vi "WVDIAL+HSRL_v5.7.vi"() -> ()   [LabVIEW 2012]
uses:
  C:/Users/eol-lidar/Desktop/20171016_WVDIALLabviewSlimmed/DLLs/PowerMeterCommands.dll
  DLLs/PowerMeterCommands.dll
  <vilib>/DAQmx/write.llb/DAQmx Write (Digital 1D Bool NChan 1Samp 1Line).vi
  <vilib>/DAQmx/miscellaneous.llb/DAQmx Fill In Error Info.vi
  <vilib>/Analysis/baseanly.llb/Mean (DBL).vi
  WVD-MCSupdate/WVDMCSupdate/Subroutines/AMCS_Data.vi
  Shared Telescope WV DIAL Code/Libraries and VIs/Scalar_Data.vi
  <vilib>/Analysis/NI_AALBase.lvlib
  Shared Telescope WV DIAL Code/Libraries and VIs/Scalar_Data_2.vi
  Shared Telescope WV DIAL Code/Libraries and VIs/Scalar_Data_4.vi
  Shared Telescope WV DIAL Code/Libraries and VIs/Scalar_Data_3.vi
  DLLs/CLDevIFace.dll
panel:
  out "WV_averaged_energy":dbl
  out "HSRL Pulse Energy":dbl=268435849.0
  out "sigma_off_total":dbl[](array[numeric])=[2.332364381390243e-25, 2.320697167741241e-25, 2.3090708671335277e-25, 2.2974854045109554e-25, 2.2859407047236247e-25, 2.2744366925441805e-25, 2.26297329267526e-25, 2.251550429733533e-25, 2.2401680282644585e-25, 2.2288260127492416e-25, 2.2175243076078264e-25, 2.206262837187045e-25, 2.1950415257769166e-25, 2.1838602976065434e-25, 2.1727190768500615e-25, 2.161617787640884e-25, 2.150556354040113e-25, 2.139534700076229e-25, 2.128552749731104e-25, 2.1176104269312273e-25, 2.106707655578666e-25, 2.095844359523096e-25, 2.0850204625897537e-25, 2.07423588855007e-25, 2.0634905611586077e-25, 2.0527844041435244e-25, 2.042117341187966e-25, 2.0314892959637173e-25, 2.0209001921078091e-25, 2.0103499532413001e-25, 1.999838502961473e-25, 1.9893657648563364e-25, 1.9789316624809672e-25, 1.968536119385491e-25, 1.9581790591098874e-25, 1.9478604051732858e-25, 1.9375800811030392e-25, 1.927338010402081e-25, 1.9171341165660125e-25, 1.906968323104925e-25, 1.896840553510801e-25, 1.886750731283709e-25, 1.8766987799273976e-25, 1.8666846229359852e-25, 1.8567081838116636e-25, 1.8467693860806868e-25, 1.836868153253588e-25, 1.8270044088719615e-25, 1.817178076472234e-25, 1.8073890796061964e-25, 1.79763734185635e-25, 1.7879227868062795e-25, 1.7782453380578935e-25, 1.768604919240875e-25, 1.7590014540037582e-25, 1.749434866014823e-25, 1.7399050789715296e-25, 1.730412016588477e-25, 1.7209556026229894e-25, 1.7115357608504846e-25, 1.702152415083449e-25, 1.6928054891539068e-25, 1.683494906948679e-25, 1.6742205923727613e-25, 1.6649824693748224e-25, 1.6557804619481728e-25, 1.6466144941105022e-25, 1.6374844899312795e-25, 1.628390373525037e-25, 1.6193320690437255e-25, 1.6103095006874383e-25, 1.6013225927008365e-25, 1.5923712693844951e-25, 1.583455455079352e-25, 1.574575074182417e-25, 1.5657300511364835e-25, 1.5569203104400362e-25, 1.5481457766563459e-25, 1.5394063743870112e-25, 1.5307020282994145e-25, 1.5220326631172624e-25, 1.5133982036225366e-25, 1.504798574650267e-25, 1.4962337011087375e-25, 1.487703507953352e-25, 1.4792079202121825e-25, 1.4707468629670718e-25, 1.4623202613699525e-25, 1.4539280406325658e-25, 1.445570126035909e-25, 1.437246442916907e-25, 1.4289569166816877e-25, 1.420701472813628e-25, 1.4124800368397896e-25, 1.404292534373148e-25, 1.3961388910802234e-25, 1.3880190327064917e-25, 1.379932885048454e-25, 1.3718803739826132e-25, 1.363861425446402e-25, 1.3558759654469082e-25, 1.3479239200466308e-25, 1.340005215388192e-25, 1.3321197776706568e-25, 1.3242675331561804e-25, 1.3164484081795858e-25, 1.3086623291318859e-25, 1.3009092224713183e-25, 1.2931890147120559e-25, 1.2855016324406373e-25, 1.2778470022930174e-25, 1.2702250509659302e-25, 1.262635705221593e-25, 1.2550788918685104e-25, 1.247554537782134e-25, 1.2400625698773462e-25, 1.2326029151422749e-25, 1.2251755005947574e-25, 1.217780253321077e-25, 1.210417100438592e-25, 1.2030859691283492e-25, 1.195786786605972e-25, 1.18851948012544e-25, 1.1812839769908239e-25, 1.1740802045427834e-25, 1.1669080901584555e-25, 1.159767561249783e-25, 1.152658545258569e-25, 1.1455809696620013e-25, 1.1385347619616093e-25, 1.131519849688941e-25, 1.1245361603937508e-25, 1.117583621651525e-25, 1.1106621610513389e-25, 1.1037717062058639e-25, 1.0969121847338734e-25, 1.0900835242690863e-25, 1.083285652457594e-25, 1.0765184969416566e-25, 1.0697819853741232e-25, 1.0630760454058555e-25, 1.0564006046922136e-25, 1.0497555908692916e-25, 1.0431409315784699e-25, 1.0365565544491242e-25, 1.0300023870946222e-25, 1.0234783571134161e-25, 1.0169843920857879e-25, 1.0105204195706285e-25, 1.0040863671053026e-25, 9.976821621998412e-26, 9.913077323333622e-26, 9.849630049554962e-26, 9.786479074821712e-26, 9.723623672876652e-26, 9.661063117109184e-26, 9.598796680486343e-26, 9.536823635511549e-26, 9.475143254257759e-26, 9.413754808236696e-26, 9.352657568504201e-26, 9.291850805513504e-26, 9.23133378922368e-26, 9.171105788951196e-26, 9.111166073406451e-26, 9.051513910691544e-26, 8.992148568247254e-26, 8.933069312831499e-26, 8.874275410530924e-26, 8.81576612669431e-26, 8.757540725943283e-26, 8.699598472176303e-26, 8.641938628496673e-26, 8.584560457246932e-26, 8.527463219959786e-26, 8.470646177359393e-26, 8.414108589358719e-26, 8.357849715001561e-26, 8.301868812469757e-26, 8.246165139113372e-26, 8.190737951368418e-26, 8.135586504842031e-26, 8.080710054163341e-26, 8.026107853101331e-26, 7.971779154486073e-26, 7.917723210229574e-26, 7.863939271325362e-26, 7.810426587789643e-26, 7.757184408704574e-26, 7.704211982217247e-26, 7.651508555513636e-26, 7.599073374786113e-26, 7.546905685292702e-26, 7.495004731290133e-26, 7.443369756106717e-26, 7.392000002064816e-26, 7.340894710500448e-26, 7.290053121808379e-26, 7.239474475327379e-26, 7.189158009533459e-26, 7.139102961790172e-26, 7.08930856857546e-26, 7.039774065355878e-26, 6.990498686564234e-26, 6.941481665748396e-26, 6.892722235390593e-26, 6.844219627029562e-26, 6.795973071186417e-26, 6.747981797479669e-26, 6.700245034457727e-26, 6.65276200971648e-26, 6.605531949891227e-26, 6.558554080616818e-26, 6.511827626512511e-26, 6.465351811259903e-26, 6.419125857514812e-26, 6.373148986943393e-26, 6.327420420220038e-26, 6.281939377011968e-26, 6.236705075965837e-26, 6.191716734741186e-26, 6.146973569929855e-26, 6.102474797122153e-26, 6.058219630831991e-26, 6.014207284541432e-26, 5.970436970619037e-26, 5.926907900376932e-26, 5.883619284018171e-26, 5.840570330591657e-26, 5.797760248023143e-26, 5.755188243052344e-26, 5.7128535211937e-26, 5.67075528677253e-26, 5.628892742806664e-26, 5.587265091058773e-26, 5.545871531927239e-26, 5.504711264423169e-26, 5.463783486157487e-26, 5.423087393251913e-26, 5.382622180326292e-26, 5.342387040404202e-26, 5.302381164874635e-26, 5.262603743431294e-26, 5.223053963979678e-26, 5.183731012619226e-26, 5.1446340734933826e-26, 5.1057623287742163e-26, 5.0671149585204396e-26, 5.02869114061869e-26, 4.9904900506887876e-26, 4.952510861986862e-26, 4.914752745251303e-26, 4.8772148686291695e-26, 4.8398963975726275e-26, 4.802796494689824e-26, 4.7659143195831185e-26, 4.7292490287976645e-26, 4.6927997756069023e-26, 4.656565709905916e-26, 4.6205459780420596e-26, 4.5847397226655986e-26, 4.5491460825835027e-26, 4.5137641925350806e-26, 4.4785931831311394e-26, 4.443632180571596e-26, 4.408880306506575e-26, 4.3743366778969376e-26, 4.340000406767262e-26, 4.3058706000731246e-26, 4.2719463594760814e-26, 4.238226781216286e-26, 4.204710955839959e-26, 4.171397968143844e-26, 4.138286896858962e-26, 4.10537681461195e-26, 4.072666787674034e-26, 4.040155875820923e-26, 4.0078431322471164e-26, 3.9757276033364395e-26, 3.9438083286394643e-26, 3.912084340726284e-26, 3.880554665095062e-26, 3.849218320163894e-26, 3.8180743171758126e-26, 3.7871216602626614e-26, 3.756359346426346e-26, 3.725786365612738e-26, 3.695401700813683e-26, 3.66520432821765e-26, 3.63519321737591e-26, 3.60536733146003e-26, 3.5757256275222147e-26, 3.546267056861835e-26, 3.516990565412017e-26, 3.48789509420622e-26, 3.458979579878315e-26, 3.430242955313054e-26, 3.40168415023669e-26, 3.3733020919928976e-26, 3.345095706363949e-26, 3.317063918393493e-26, 3.2892056533936244e-26, 3.2615198379443223e-26, 3.234005401005175e-26, 3.206661275068879e-26, 3.179486397425954e-26, 3.1524797114255725e-26, 3.125640167867499e-26, 3.09896672641198e-26, 3.0724583570023383e-26, 3.046114041394335e-26, 3.0199327746539526e-26, 2.9939135667250263e-26, 2.968055443914684e-26, 2.9423574505128714e-26, 2.9168186502296844e-26, 2.891438127743385e-26, 2.8662149900966553e-26, 2.841148368095994e-26, 2.816237417598619e-26, 2.791481320722609e-26, 2.7668792869488795e-26, 2.742430554080934e-26, 2.718134389112318e-26, 2.693990088912774e-26, 2.66999698074146e-26, 2.6461544226517236e-26, 2.6224618036475193e-26, 2.598918543714353e-26, 2.5755240935978997e-26, 2.55227793446944e-26, 2.5291795773344677e-26, 2.506228562275398e-26, 2.4834244575138018e-26, 2.4607668582883306e-26, 2.438255385569937e-26, 2.4158896845945432e-26, 2.3936694232798251e-26, 2.371594290486372e-26, 2.349663994197427e-26, 2.3278782595424064e-26, 2.3062368268002568e-26, 2.2847394493076405e-26, 2.2633858913405882e-26, 2.2421759259664502e-26, 2.2211093328951717e-26, 2.2001858963497252e-26, 2.1794054029696938e-26, 2.158767639770168e-26, 2.138272392158188e-26, 2.1179194420452825e-26, 2.0977085660508756e-26, 2.0776395337905693e-26, 2.0577121063165076e-26, 2.037926034667947e-26, 2.018281058531128e-26, 1.99877690506497e-26, 1.9794132878407814e-26, 1.9601899059288993e-26, 1.9411064431318812e-26, 1.9221625673258913e-26, 1.9033579299585288e-26, 1.8846921656793268e-26, 1.8661648920586673e-26, 1.847775709457811e-26, 1.8295242010014096e-26, 1.8114099326188242e-26, 1.7934324532407428e-26, 1.775591295030433e-26, 1.7578859736980766e-26, 1.7403159889222226e-26, 1.7228808247949143e-26, 1.7055799503287488e-26, 1.688412820024058e-26, 1.6713788744552824e-26, 1.6544775409065492e-26, 1.637708234013833e-26, 1.621070356441011e-26, 1.6045632995668e-26, 1.588186444155174e-26, 1.571939161069008e-26, 1.5558208119481574e-26, 1.539830749889085e-26, 1.5239683201286934e-26, 1.5082328606968512e-26, 1.492623703067143e-26, 1.4771401727800933e-26, 1.461781590053534e-26, 1.4465472703745876e-26, 1.4314365250563953e-26, 1.4164486617845617e-26, 1.4015829851356042e-26, 1.3868387970670347e-26, 1.372215397393606e-26, 1.3577120842198647e-26, 1.3433281543732342e-26, 1.3290629037929928e-26, 1.3149156278959545e-26, 1.3008856219417433e-26, 1.2869721813426649e-26, 1.2731746019815118e-26, 1.2594921804819474e-26, 1.245924214476847e-26, 1.2324700028536295e-26, 1.2191288459758865e-26, 1.205900045887559e-26, 1.1927829065033005e-26, 1.1797767337869046e-26, 1.1668808358980381e-26, 1.1540945233430018e-26, 1.1414171091057127e-26, 1.1288479087555434e-26, 1.1163862405612263e-26, 1.104031425576237e-26, 1.091782787727406e-26, 1.0796396538871236e-26, 1.0676013539317827e-26, 1.0556672208023929e-26, 1.0438365905502061e-26, 1.0321088023734669e-26, 1.0204831986549954e-26, 1.0089591249905554e-26, 9.975359302025957e-27, 9.862129663617662e-27, 9.749895887973517e-27, 9.63865156105144e-27, 9.528390301448673e-27, 9.419105760458501e-27, 9.310791622019825e-27, 9.203441602575011e-27, 9.097049451061688e-27, 8.991608948776884e-27, 8.887113909137442e-27, 8.783558177658376e-27, 8.680935631666101e-27, 8.579240180169365e-27, 8.478465763623746e-27, 8.378606353692343e-27, 8.279655953065625e-27, 8.181608595193189e-27, 8.084458344058879e-27, 7.988199293893197e-27, 7.892825568987107e-27, 7.798331323397119e-27, 7.704710740628208e-27, 7.611958033526109e-27, 7.520067443844823e-27, 7.429033242095497e-27, 7.338849727257468e-27, 7.249511226494639e-27, 7.161012094933005e-27, 7.073346715375045e-27, 6.986509498044532e-27, 6.90049488038543e-27, 6.81529732672126e-27, 6.730911328102361e-27, 6.64733140200458e-27, 6.564552092115001e-27, 6.482567968084595e-27, 6.401373625321456e-27, 6.320963684734177e-27, 6.2413327925242824e-27, 6.162475619977861e-27, 6.084386863225426e-27, 6.0070612430594456e-27, 5.93049350473708e-27, 5.854678417728619e-27, 5.7796107755822155e-27, 5.705285395699283e-27, 5.631697119157481e-27, 5.558840810516501e-27, 5.486711357676057e-27, 5.415303671645201e-27, 5.3446126864241e-27, 5.274633358812004e-27, 5.205360668273596e-27, 5.136789616728847e-27, 5.068915228464904e-27, 5.001732549942197e-27, 4.935236649672937e-27, 4.869422618068433e-27, 4.804285567298274e-27, 4.7398206311792526e-27, 4.67602296502107e-27, 4.612887745512478e-27, 4.5504101705978505e-27, 4.488585459351163e-27, 4.4274088518740324e-27, 4.366875609158459e-27, 4.306981013010063e-27, 4.247720365906535e-27, 4.18908899092025e-27, 4.1310822316100614e-27, 4.0736954519098816e-27, 4.016924036061156e-27, 3.960763388494195e-27, 3.905208933744127e-27, 3.850256116386455e-27, 3.79590040090594e-27, 3.742137271667819e-27, 3.6889622327949254e-27, 3.63637080812266e-27, 3.58435854108821e-27, 3.532920994696357e-27, 3.482053751411668e-27, 3.4317524131156784e-27, 3.3820126010277366e-27, 3.332829955639945e-27, 3.284200136649963e-27, 3.2361188229165776e-27, 3.1885817123724097e-27, 3.1415845219948863e-27, 3.095122987735941e-27, 3.0491928644700905e-27, 3.0037899259518407e-27, 2.958909964743249e-27, 2.914548792187844e-27, 2.8707022383363006e-27, 2.8273661519104936e-27, 2.7845364002578585e-27, 2.742208869297717e-27, 2.700379463492681e-27, 2.659044105789684e-27, 2.6181987375948592e-27, 2.5778393187241496e-27, 2.5379618273728972e-27, 2.4985622600683314e-27, 2.4596366316510014e-27, 2.4211809752142476e-27, 2.3831913420937183e-27, 2.3456638018206104e-27, 2.3085944420907525e-27, 2.271979368742305e-27, 2.235814705714131e-27, 2.200096595014933e-27, 2.164821196714334e-27, 2.1299846888874138e-27, 2.0955832676121665e-27, 2.061613146922824e-27, 2.0280705588054778e-27, 1.9949517531484858e-27, 1.9622529977418628e-27, 1.929970578245345e-27, 1.8981007981568767e-27, 1.866639978803457e-27, 1.8355844593123698e-27, 1.804930596599854e-27, 1.774674765337153e-27, 1.7448133579373653e-27, 1.715342784545853e-27, 1.686259473007412e-27, 1.657559868855308e-27, 1.629240435298082e-27, 1.6012976531931827e-27, 1.5737280210392883e-27, 1.5465280549576587e-27, 1.5196942886780578e-27]
  out "sigma_on_total":dbl[](array[numeric])=[2.4625508330472582e-23, 2.4527159853669705e-23, 2.4428740710389365e-23, 2.4330256235021162e-23, 2.4231711731485397e-23, 2.413311246438279e-23, 2.4034463665998014e-23, 2.3935770531217886e-23, 2.3837038220808932e-23, 2.3738271855481437e-23, 2.363947652194091e-23, 2.354065726790698e-23, 2.3441819104494084e-23, 2.3342967003119844e-23, 2.3244105897895672e-23, 2.31452406834776e-23, 2.304637621655468e-23, 2.2947517312839898e-23, 2.284866874947935e-23, 2.274983526208387e-23, 2.2651021548034267e-23, 2.2552232261770784e-23, 2.2453472020760115e-23, 2.2354745396413204e-23, 2.2256056922707838e-23, 2.2157411090680185e-23, 2.2058812350863854e-23, 2.1960265109616345e-23, 2.186177373417321e-23, 2.176334254726737e-23, 2.16649758304535e-23, 2.1566677823093633e-23, 2.1468452720517898e-23, 2.137030467733218e-23, 2.1272237803888927e-23, 2.1174256167903837e-23, 2.1076363794365574e-23, 2.0978564665455582e-23, 2.0880862718807766e-23, 2.0783261851638762e-23, 2.0685765914020924e-23, 2.0588378716350403e-23, 2.049110402431887e-23, 2.039394555974215e-23, 2.0296907001380106e-23, 2.019999198493379e-23, 2.0103204103051482e-23, 2.0006546904536104e-23, 1.991002389599258e-23, 1.981363853864059e-23, 1.9717394252391202e-23, 1.9621294413479896e-23, 1.952534235533098e-23, 1.9429541367045723e-23, 1.9333894696646757e-23, 1.9238405547999238e-23, 1.914307708248763e-23, 1.9047912419885998e-23, 1.895291463612763e-23, 1.8858086764984376e-23, 1.876343179818248e-23, 1.8668952684763187e-23, 1.857465233274633e-23, 1.8480533606982316e-23, 1.8386599332337e-23, 1.8292852289311177e-23, 1.8199295218736272e-23, 1.8105930821158984e-23, 1.801276175403204e-23, 1.7919790634879415e-23, 1.782702003925766e-23, 1.7734452504618375e-23, 1.764209052536127e-23, 1.754993655815298e-23, 1.7457993017035543e-23, 1.736626227799225e-23, 1.7274746676980947e-23, 1.718344851157997e-23, 1.7092370038359167e-23, 1.7001513476664478e-23, 1.6910881006007085e-23, 1.682047476841214e-23, 1.673029686585863e-23, 1.664034936539259e-23, 1.6550634294490077e-23, 1.6461153642030332e-23, 1.637190936129231e-23, 1.6282903368814e-23, 1.6194137543294374e-23, 1.6105613727888785e-23, 1.601733372844626e-23, 1.5929299315126343e-23, 1.584151222397945e-23, 1.5753974153233175e-23, 1.566668676754455e-23, 1.5579651696281607e-23, 1.5492870534454802e-23, 1.5406344842343154e-23, 1.53200761464224e-23, 1.5234065938363693e-23, 1.5148315678510935e-23, 1.506282679169264e-23, 1.497760067132952e-23, 1.4892638678431833e-23, 1.4807942139395617e-23, 1.4723512351289847e-23, 1.4639350577157742e-23, 1.4555458050642286e-23, 1.4471835972573456e-23, 1.4388485513719354e-23, 1.430540781325041e-23, 1.422260398085087e-23, 1.414007509639349e-23, 1.4057822209041305e-23, 1.397584633933156e-23, 1.3894148477689867e-23, 1.3812729587076428e-23, 1.373159060034607e-23, 1.365073242288479e-23, 1.35701559323074e-23, 1.3489861978173715e-23, 1.340985138229009e-23, 1.3330124939573234e-23, 1.3250683417775063e-23, 1.3171527559452338e-23, 1.3092658079451777e-23, 1.3014075666890917e-23, 1.2935780985987886e-23, 1.2857774674695026e-23, 1.278005734609298e-23, 1.2702629589208426e-23, 1.2625491966604325e-23, 1.2548645018972756e-23, 1.2472089261122236e-23, 1.2395825185468206e-23, 1.2319853260187866e-23, 1.2244173930563517e-23, 1.2168787619771422e-23, 1.2093694727085487e-23, 1.201889563074398e-23, 1.1944390685652608e-23, 1.1870180226217995e-23, 1.1796264564579593e-23, 1.172264399190066e-23, 1.164931877912693e-23, 1.1576289174773247e-23, 1.1503555409156319e-23, 1.1431117690705314e-23, 1.1358976208694298e-23, 1.1287131133002929e-23, 1.1215582613893397e-23, 1.1144330782277625e-23, 1.1073375750454047e-23, 1.1002717612825146e-23, 1.0932356443802581e-23, 1.0862292301349351e-23, 1.0792525225341324e-23, 1.072305523736658e-23, 1.0653882341902861e-23, 1.0585006526555719e-23, 1.0516427762743505e-23, 1.0448146003690532e-23, 1.0380161187372578e-23, 1.0312473235839991e-23, 1.02450820545726e-23, 1.017798753360374e-23, 1.01111895481767e-23, 1.0044687956810886e-23, 9.978482604560173e-24, 9.912573321075102e-24, 9.846959922109027e-24, 9.781642208049517e-24, 9.716619965832612e-24, 9.651892968316416e-24, 9.587460975732818e-24, 9.52332373302031e-24, 9.459480973330377e-24, 9.395932416584771e-24, 9.332677769690737e-24, 9.269716726754081e-24, 9.207048969290063e-24, 9.144674167996041e-24, 9.082591980187603e-24, 9.02080205158559e-24, 8.959304016889022e-24, 8.898097498808089e-24, 8.83718210940996e-24, 8.776557449163434e-24, 8.7162231078921e-24, 8.656178665324571e-24, 8.596423689788587e-24, 8.536957739886005e-24, 8.477780363928673e-24, 8.418891100483173e-24, 8.360289478541112e-24, 8.301975016976582e-24, 8.243947225442954e-24, 8.18620560453709e-24, 8.128749645613794e-24, 8.071578831649707e-24, 8.014692636017133e-24, 7.958090524040087e-24, 7.901771952798669e-24, 7.845736370274257e-24, 7.789983217537724e-24, 7.734511926875921e-24, 7.679321923290004e-24, 7.624412623323213e-24, 7.569783437184724e-24, 7.515433766925708e-24, 7.461363007572737e-24, 7.40757054726645e-24, 7.354055767082815e-24, 7.300818041492451e-24, 7.247856738183225e-24, 7.195171218202832e-24, 7.142760836711679e-24, 7.090624942188402e-24, 7.038762877181533e-24, 6.987173978433868e-24, 6.935857576708368e-24, 6.884812996920365e-24, 6.834039558853511e-24, 6.783536576104506e-24, 6.733303357674044e-24, 6.683339207201171e-24, 6.633643422518733e-24, 6.584215297489166e-24, 6.535054120403026e-24, 6.486159174952553e-24, 6.437529740614361e-24, 6.389165091649568e-24, 6.341064498325356e-24, 6.293227226467728e-24, 6.2456525381077956e-24, 6.1983396902435295e-24, 6.151287936822558e-24, 6.104496527501172e-24, 6.0579647080188635e-24, 6.011691720302102e-24, 5.965676803332971e-24, 5.919919192206112e-24, 5.8744181179864905e-24, 5.829172809574231e-24, 5.784182492018668e-24, 5.7394463868786454e-24, 5.694963713545303e-24, 5.650733687844412e-24, 5.6067555226267894e-24, 5.5630284285725715e-24, 5.519551613069912e-24, 5.476324281024295e-24, 5.43334563516773e-24, 5.3906148752017374e-24, 5.34813119904406e-24, 5.3058938017475215e-24, 5.2639018765006215e-24, 5.222154614242014e-24, 5.180651203738997e-24, 5.13939083210488e-24, 5.0983726842026865e-24, 5.057595942945583e-24, 5.017059789585322e-24, 4.976763403989191e-24, 4.936705964060656e-24, 4.896886645818459e-24, 4.857304624305925e-24, 4.817959073015348e-24, 4.778849163546343e-24, 4.7399740669056344e-24, 4.7013329523320734e-24, 4.662924987776317e-24, 4.624749340755355e-24, 4.586805176615996e-24, 4.549091660777239e-24, 4.5116079568120655e-24, 4.474353227687181e-24, 4.437326635994939e-24, 4.400527342481393e-24, 4.363954508194969e-24, 4.327607292829392e-24, 4.291484855352226e-24, 4.255586354786274e-24, 4.21991094878835e-24, 4.1844577951629254e-24, 4.149226050818604e-24, 4.114214872712741e-24, 4.079423416657998e-24, 4.044850839129298e-24, 4.010496295553295e-24, 3.976358941574372e-24, 3.942437932236539e-24, 3.908732422878395e-24, 3.875241568493912e-24, 3.841964524111771e-24, 3.8089004445060674e-24, 3.77604848472963e-24, 3.743407799821842e-24, 3.7109775448496736e-24, 3.6787568751051834e-24, 3.646744945826577e-24, 3.614940912861531e-24, 3.583343931919993e-24, 3.551953159080269e-24, 3.520767750819167e-24, 3.48978686389268e-24, 3.459009655371579e-24, 3.428435282822815e-24, 3.398062904337347e-24, 3.367891678126286e-24, 3.3379207634216245e-24, 3.308149319353983e-24, 3.278576506269015e-24, 3.2492014844797096e-24, 3.2200234154212834e-24, 3.1910414609759742e-24, 3.1622547835091576e-24, 3.1336625464392295e-24, 3.105263913718335e-24, 3.077058049866742e-24, 3.0490441205265137e-24, 3.0212212919554575e-24, 2.993588731187521e-24, 2.9661456063117672e-24, 2.938891086110655e-24, 2.9118243402152735e-24, 2.8849445392530034e-24, 2.8582508548661334e-24, 2.83174245960934e-24, 2.805418526973212e-24, 2.7792782314072863e-24, 2.7533207485771068e-24, 2.7275452549106983e-24, 2.7019509282066268e-24, 2.676536946955093e-24, 2.65130249127828e-24, 2.6262467418057974e-24, 2.601368880939825e-24, 2.5766680916364768e-24, 2.552143558429287e-24, 2.5277944668893196e-24, 2.5036200038621456e-24, 2.4796193572700426e-24, 2.4557917163440066e-24, 2.432136271843243e-24, 2.408652215237557e-24, 2.3853387397641406e-24, 2.3621950397159215e-24, 2.3392203108656813e-24, 2.3164137500783173e-24, 2.2937745558238835e-24, 2.2713019277921793e-24, 2.2489950670083638e-24, 2.22685317584767e-24, 2.2048754582373562e-24, 2.1830611194759734e-24, 2.1614093661554926e-24, 2.1399194064524524e-24, 2.118590449772077e-24, 2.0974217072161272e-24, 2.0764123913175484e-24, 2.0555617157912343e-24, 2.0348688963376748e-24, 2.014333149601918e-24, 1.9939536942280065e-24, 1.9737297501740007e-24, 1.9536605387321687e-24, 1.9337452830413488e-24, 1.9139832077558902e-24, 1.8943735388152807e-24, 1.8749155039447973e-24, 1.8556083325745714e-24, 1.836451255374024e-24, 1.8174435048180336e-24, 1.7985843149555666e-24, 1.779872921494777e-24, 1.7613085616590394e-24, 1.7428904742740746e-24, 1.7246178999963703e-24, 1.706490080876167e-24, 1.688506260735766e-24, 1.67066568509952e-24, 1.652967600988165e-24, 1.6354112573505205e-24, 1.6179959045079075e-24, 1.6007207947196642e-24, 1.5835851817734365e-24, 1.5665883211992682e-24, 1.549729470273379e-24, 1.5330078878919895e-24, 1.5164228347105305e-24, 1.4999735731470965e-24, 1.4836593672601718e-24, 1.4674794829453382e-24, 1.4514331876891116e-24, 1.4355197508254798e-24, 1.419738443475347e-24, 1.4040885383117088e-24, 1.388569310046027e-24, 1.3731800348365029e-24, 1.3579199909426112e-24, 1.342788458086281e-24, 1.327784718035644e-24, 1.3129080540946768e-24, 1.2981577515607805e-24, 1.2835330973375337e-24, 1.26903338027142e-24, 1.2546578909355328e-24, 1.2404059216902307e-24, 1.2262767667918795e-24, 1.2122697222380488e-24, 1.1983840857753642e-24, 1.1846191571075761e-24, 1.1709742376439593e-24, 1.1574486307543798e-24, 1.1440416414751332e-24, 1.1307525767609108e-24, 1.1175807454362942e-24, 1.1045254581039964e-24, 1.0915860272441287e-24, 1.0787617671245363e-24, 1.0660519939877606e-24, 1.0534560258245474e-24, 1.04097318247118e-24, 1.0286027857002782e-24, 1.0163441591336192e-24, 1.0041966282035836e-24, 9.92159520201455e-25, 9.802321644465981e-25, 9.684138919121806e-25, 9.56704035604766e-25, 9.451019303983845e-25, 9.336069129593208e-25, 9.222183219101463e-25, 9.109354977514304e-25, 8.997577829031332e-25, 8.886845216306286e-25, 8.77715060087434e-25, 8.668487464281262e-25, 8.560849305520192e-25, 8.454229644363315e-25, 8.348622018112683e-25, 8.244019984154291e-25, 8.1404171188931855e-25, 8.037807017106822e-25, 7.936183294026076e-25, 7.835539582967759e-25, 7.735869536732837e-25, 7.637166827936458e-25, 7.539425147725231e-25, 7.442638207102039e-25, 7.346799736295037e-25, 7.251903484175774e-25, 7.157943220136464e-25, 7.064912731956171e-25, 6.9728058273561595e-25, 6.88161633340924e-25, 6.791338096567603e-25, 6.701964982690402e-25, 6.61349087734962e-25, 6.525909685563692e-25, 6.439215331824889e-25, 6.353401760126324e-25, 6.268462934252213e-25, 6.184392837266436e-25, 6.101185472583387e-25, 6.0188348621694805e-25, 5.937335048636966e-25, 5.8566800942157565e-25, 5.776864079808227e-25, 5.697881107478359e-25, 5.619725298250847e-25, 5.542390792885821e-25, 5.465871752134281e-25, 5.390162356973914e-25, 5.315256807486063e-25, 5.241149324030067e-25, 5.1678341470200395e-25, 5.095305536292852e-25, 5.023557772008194e-25, 4.952585154435521e-25, 4.882382003144208e-25, 4.812942658286226e-25, 4.744261479979235e-25, 4.676332848135732e-25, 4.609151162889621e-25, 4.542710844416201e-25, 4.477006333333286e-25, 4.412032089587425e-25, 4.347782594176257e-25, 4.284252347666972e-25, 4.221435871147735e-25, 4.159327705702398e-25, 4.097922412620583e-25, 4.0372145739307014e-25, 3.97719879138551e-25, 3.9178696871826257e-25, 3.8592219041386377e-25, 3.801250105051675e-25, 3.743948973222074e-25, 3.687313212310302e-25, 3.6313375466665607e-25, 3.57601672058255e-25, 3.521345499384773e-25, 3.4673186682507077e-25, 3.41393103342396e-25, 3.361177421349018e-25, 3.309052679134557e-25, 3.2575516744308053e-25, 3.2066692955889386e-25, 3.156400451278687e-25, 3.1067400711850723e-25, 3.057683105489688e-25, 3.0092245249061445e-25, 2.9613593210871453e-25, 2.9140825062631734e-25, 2.8673891136375487e-25, 2.8212741969193266e-25, 2.775732830716305e-25, 2.7307601105501903e-25, 2.686351152759651e-25, 2.6425010943041874e-25, 2.5992050934598855e-25, 2.5564583291660275e-25, 2.5142560011733776e-25, 2.472593330387952e-25, 2.4314655586748254e-25, 2.390867948982882e-25, 2.35079578506624e-25, 2.3112443719124123e-25, 2.2722090354652053e-25, 2.233685122844375e-25, 2.195668002362015e-25, 2.158153063268651e-25, 2.121135716059416e-25, 2.0846113925777074e-25, 2.0485755456818577e-25, 2.0130236495370295e-25, 1.977951199549295e-25, 1.9433537124710145e-25, 1.9092267261784236e-25, 1.8755658001017306e-25, 1.8423665149969254e-25, 1.809624472667617e-25, 1.7773352967583335e-25, 1.7454946320086584e-25, 1.7140981448046972e-25, 1.683141522831366e-25, 1.6526204752468635e-25, 1.6225307329089313e-25, 1.592868047980234e-25, 1.5636281943616514e-25, 1.5348069673765125e-25, 1.5064001839312553e-25, 1.4784036827229053e-25, 1.450813323820404e-25, 1.423624989244445e-25]
  out "FileHour":i32=6
  out "L_Count":i32
  out "background start":u32=534
  in  "Tab Control 2":enum32{"WV ND ", "Aerosol Backscatter"}(tab)=enum."Aerosol Backscatter"
  out "Absolute Humdity":dbl[][](graph)=[[3.7891452578622107, 3.6848538050283244, 3.4581562862034234, 2.778190123006674, 0.7605224233485954, 2.7235239960819384, 1.8477030284137896, 1.3789174154224018, 3.858909817141913, 2.2998052504653157, 1.8697427873996968, 2.720429333025646, 1.7582764295120719, 1.8343313251572997, 1.160757957156007, 1.3664787572167836, 1.0278245657680662, 0.9747102705897372, 2.2692052714590547, 2.447303873258803, 2.2600819196275466, 2.0700601873456366, 2.0466223675290682, 1.6983309570610874, 1.7492798993149568, 1.7861585039993737, 1.5832308094702108, 1.5864879871964421, 1.5030372754279626, 1.4564317158867097, 1.4228817850819906, 2.096958434429432, 2.4022604300017574, 2.66591970440604, 2.8116941850803556, 1.9044240843725713, 1.66818020635356, 1.534265057004012, 1.772166434272927, 2.497662922277854, 1.6957482922208336, 1.2977864394369667, 1.362279941674365, 1.629191662274515, 1.657338578258699, 1.6301344411474732, 1.516535077188046, 1.3406588492672837, 1.6412452976171872, 1.8344293332702541, 1.9351027937999632, 2.5531676991990513, 2.659011166233257, 1.742648255830912, 1.7524741749995578, 1.6769853502577594, 1.4000548013411225, 1.4245808617975315, 1.37878612948763, 1.7417128820940007, 1.7571933484059967, 1.4600862013864073, 1.1537350022625028, 1.4142394580617093, 1.1174683443965145, 1.2022225697660078, 1.4769074840251073, 1.6984425714113995, 1.8751873013694706, 0.7714280687239269, 0.7769992656400687, 0.9738206307167362, 1.0399777595055186, 1.5775455874643123, 1.9662515652956385, 2.890017835586726, 2.984091683481171, 1.7840363622336388, 1.5747914857098424, 3.3692935433573963, 3.9625775177433993, 2.7959569186438222, 2.8123955756125945, 2.372892243619342, 1.4831028352176765, 0.06273774369447636, -0.5977961214933015, 1.5843209354443428, 2.8625329307407408, 2.5733621942741647, 0.6933039516447836, 0.6539560692382185, 0.8040980030154087, 0.8084018088922339, 1.6344508657792636, 0.37454636863898716, 0.440972361188328, 1.373103149482538, 0.7494498912843306, -1.4788274396233316, -1.1562199736918923, -0.5463545775679522, 1.0349505513673738, 1.138127242006889, -1.0589464926009615, 1.9469246537317555, 2.688644087271129, -0.2951872731857954, -2.6561570659511995, -1.4087504983005419, 0.9568858008879041, -0.27670896981197296, -2.0798321684324503, -0.0002528932543105229, 6.422466595855947, 4.958249789600535, -0.772999155805734, -1.1846414669496275, 0.052326411990904466, -0.47672243031922984, -0.17931113920046696, 5.842686469331913, 3.28233118981728, -0.9449483030259822, -0.32664929120777414, -1.5692345779065195, 4.032753921147751, 9.877331127854655, 8.25122205980245, 7.00075444422831, -0.5203550683182948, -7.139395363542666, -2.245960526012101, 0.9022165152520595, 2.163914779345491, 2.217229143883716, 1.0363924828691926, -1.3944188053069932, -4.557806574544715, 2.1301279232496753, 11.253191554758521, 2.064944061831564, -2.6177477476732083, 1.6398384571905356, -4.091283656679752, -8.308017355766843, -8.23837798110966, -9.616699249521794, -3.0581988015017414, -5.361741358485176, -5.748951386641595, 7.916782763362802, 8.58613890353965, 1.805003746330035, -2.7606593015623857, 2.8229983856836904, 8.179047139473575, -1.0584671044673364, -2.6399610247117584, 0.237764480846984, -8.03257612525808, -1.9612530530287045, -0.6576984232446915, -1.0310392201536338, 4.081560129871335, 5.607657340538373, -1.9846456305856168, -3.748929894242704, 9.722430027786967, 13.624903283470438, 11.587839001539427, -2.055100939382735, -9.402788923073796, 10.094955958347954, 13.62741394978795, -10.632580762183446, -12.734663168850785, 10.311651343461506, 20.85224512815382, -4.3275848189848425, -5.989923962964441, 5.178401649012232, 10.319226015000389, 2.5382716479921736, 10.949170850907755, 32.327800616503794, 45.83620146719581, 38.116654598360626, -24.661951290179545, -21.930144450377615, 4.687848975824733, -11.869457319667122, -4.929093686741239, 26.118574237518214, 0.3978284325576861, -10.279325555109535, -39.884984474783764, -52.386616489245945, 14.978277519868852, 39.35943905108406, 22.648280256525634, 26.27910985615595, 15.653043046574338, -2.153617510982033, 2.7151347485545148, -4.225796293412116, 13.941645753941094, -2.4014760480976967, -32.47515403044753, -26.04348444985774, -21.11142576095537, 6.588726145252684, 32.710853341574456, -6.867298147707661, -7.8382790473753206, -1.3192131900762427, -30.277295702455284, -7.683781400205925, 21.229002625990447, 17.554097782409254, 9.57279553418554, -22.841402169478357, -58.25256018396276, -49.69608950783632, -56.94824512078988, -35.259449579757224, 6.158572431930525, 15.224298784487187, -13.68715652650741, -49.62018273724492, -21.05078140588219, 0.0021830788129874375, 10.687032340398043, 71.35524204081668, 86.33524750768028, 37.130163911814606, 21.443941954669604, 19.156569157740908, 16.3362725474402, 34.76161064908747, -23.80598198719804, -17.464931362142504, 26.53857841970044, -47.46454821109903, -43.310613526313446, 42.05912741409695, 29.89120971129882, -22.772869569089604, -11.34748079308518, 27.089137996134312, 51.58360797663678, 519.5216737651713, 267.90532470515126, -3.8406150092167337, -33.96897578835663, -72.09049673577762, -33.68326806976822, -38.07872702781121, -51.10703820612141, -15.525332356936735, -47.815517079384435, -544.6933847259934, -334.25449125707706, 26.127866920500402, 73.36798280169113, -15.270782998101042, -17.48610203876438, 52.828253341246125, 62.303899593586806, -16.50288980048265, 19.969658387364394, 36.46081737344103, 39.51915177206713, -28.356294716050183, -44.492871490811794, 44.29362891629997, 35.48733731073473, 4.194075784201305, 2.095847410586148, 24.171725569204437, 20.01904503791074, 10.50035475239806, 17.83235800493499, -3.4224236879255336, -78.87187438004007, -94.81248998820931, 87.86322549359974, 247.39835388441986, -17.43457965663944, -25.428031525062913, -122.75601693044112, -81.92764316479855, -19.88928623071795, -44.21108066246693, 55.09017109350039, 150.30511463298143, -158.19341303985513, -356.69290295635045, -33.09718562692851, -20.67864485957666, 33.8931351602775, 124.01000974483895, 62.36626980698904, -107.84589818593308, -101.67266701731596, -245.1081550291804, -35.19835381490422, 188.1152914234046, -29.566356703706784, 44.86913335259721, 92.64476538761167, -39.16590666833693, -115.14393723590348, 418.7096326303462, 39.2917301702867, 472.37361036549163, 102.40312762280362, -183.00844504061064, 18.482851898926672, -55.16435420299342, 95.97084035327337, -55.93876185079815, 334.1340494792696, -226.31634564517833, 105.8703342150248, -79.40424453497434, -134.04960975245834, 251.12510765502915, -80.98998024227055, -252.76662576333678, 108.70915319573854, 19.096752246660266, -333.611892349151, -17.89108575609415, 60.895773394876876, -240.4838824781284, 182.8829822532551, -118.42442070761707, -83.25810028510192, 52.192223057925474, -838.65983196708, 249.97784369432594, 59.36087636245584, -79.92236485506722, -266.64510264213305, -249.26521570172204, -193.66047759048476, -98.8781564717847, 174.56192059816868, 279.80223640531045, 596.1125725480475, -187.19813920651282, 151.4100790790567, 270.68515987663557, -76.09001228539832, -218.57131022295502, -217.6303286775662, 82.14828593934855, 558.4170943181765, -249.38651639694498, -354.8232394089802, -108.17912895447277, 75.81909810073923, -439.57674462484505, 677.522117376858, 453.4638761137788, 174.05803558045963, -292.8657137732941, -670.1998920169691, 106.56626857230592, 435.35535825156376, 62.76307965005727, 37.71263794469746, -192.29584269690054, -798.9239547108301, 100.5167007167806, 141.62062704412352, 480.279457941861, 125.64316156897276, -154.80092143614473, -659.5268368862085, -820.2356625580233, -536.0990382961583, 993.9553843130275, 267.9571397651825, 37.14505704952786, -297.01747669244173, -1324.2132172245103, -1311.3205571152982, 508.58289607659736, 1097.1708071591079, 66.58310375415361, 16.26303923273612, -1247.133159983727, -726.6196253064362, 43.71040394718472, 427.9382917880595, 1595.3253551307507, 1139.0822537618337, -448.69246220068464, -334.7705466259942, 190.482633701428, -1199.5255614849482, -51.14419897443197, 1397.5822325414642, -154.5107028559919, -219.57153056271454, -633.1290478570163, -128.5457652537974, -417.97323330579326, -210.69341672612083, 926.4212039947977, 1753.780308170262, 208.3990380132587, -814.0634849813144, -698.1146115626569, 829.1423962858821, 166.17667567279784, 439.4569229889019, -30.972247411393962, 179.38200940264596, 505.5911230824318, -918.2246418491548, 877.1834325018763, -172.96271214104183, -634.3396199889318, -905.3794681655005, 1005.6004239202559, 74.00757274912135, -242.1271413755767, -261.191198838452, -1483.6660198136576, 755.7939418391852, -164.48058273529773, 464.0442715930656, 419.69396401521044, -154.993036378201, -542.0981883975094, -199.91160457006708, 467.6080881758015, -84.3906123421621, 828.58413464251, -633.1581916903907, -1168.6653917890994, -666.9836750340943, 466.7676012644678, -1559.982584274613, -1200.0308972871112, -820.5177152473607, -1372.3514036116119, -947.4733929751944, -623.3661340694022, 558.5685404099348, 2205.4891705284454, -416.97310893874607, 1440.9834011391074, 1405.4354183317216, -55.03931004697145, -826.1927059583878, -343.94785565379925, 1628.656121117055, -922.9170677826108, 408.1883705978928, -3138.2738676050585, 299.3685795903448, -2398.8450377266904, 386.2385382705187, -1445.7717921580922, 1395.1748385638098, -353.9937790270451, -1763.3184421397464, 1337.1494929403727, -2108.2782562757993, 251.57257689210763, 817.4918321565656, 377.7262144230666, 60.787259400091216, 1645.975719043345, -57.357168196870006, 3027.7370068355117, 216.58080107005247, -470.277313193831, 2104.4819842819625, 1975.317474173985, 1094.6716205818523, 722.7910357231889, 522.3770312481151, -1723.199954801544, -395.73758502408845, -2409.316726764381, -110.4702457244176, 394.12983818033297, -2251.591471953941, -4469.593268193903, -3357.7436822036666, 28.172754159949438, -1136.948109653774, -3397.5700401874415, 1342.8884409858586, 1506.7693189458953, 1704.6653097079704, -1090.1677301745158, 88.54938929449003, 3976.6871795479046, 1633.171202676323, -3754.546639755709, 744.4514789168554, 6416.5643521853235, 859.8818569426231, 602.7365870816462, 1120.1235987768039, 3790.8982611171255, 2637.848421630551, 249.3967546336423, 681.8093734762921, 1038.8743983525299, 870.7775894992534, -166.6296660686713, -1745.0083012879118, -1551.3328850085857, 3675.3181009519994, 4841.85927908997, -3506.466187953114, 2233.0550829048893, -1447.390366501281, 2569.198406613939, -653.2732426709086, 971.1049068314007, 2482.1525468856257, 3571.446295341718, -6647.674676255461, -7125.370977477677, 9485.106555908935, -833.2713838673917, -1550.0017462475544, -4416.63339590602, -1132.1804791240177, -3032.571375007294, 12861.657711070708, -241.5480761185041, 3248.8554971940325, -4501.5950139371835, -8900.716162175044, 3903.2352876565187, 5082.963365614041, 3267.817788107922, -450.47936593911055, 2047.9524790476805, -17650.7604544819, 1311.0641222840604, -3003.296620662897, 3073.0435587641555, 885.5662541074555, -6468.983509459631, -3296.19469372451, 493.967866263296, 0.0, 0.0, 0.0, 0.0]] caption="Water Vapor Number Density"
  out "Backscatter coef":dbl[][](graph)=[[-6.21843595794976, -6.549540022672395, -6.2422521030397515, -6.2965877173945906, -6.662418290190171, -6.429653945846613, -5.924353821499211, -6.051984355656097, -6.433612899413857, -6.599497650811813, -6.558926620056004, -6.760030632932293, -6.718925744856284, -6.809239409280793, -6.70636245157723, -6.593919782010744, -6.677612094263719, -6.670518612306596, -6.771425101476374, -6.695268049620202, -6.631570463641731, -6.7539522703696395, -6.773811177815455, -6.816445041548573, -6.749935965084725, -6.693501871437421, -6.821279586266254, -6.839849222560982, -6.802649130089231, -6.985346277759823, -7.056047751304795, -6.892559255477837, -6.7511921327643964, -6.73617500559804, -6.726884996505748, -6.749017098541033, -6.763024285766058, -6.675660469867444, -6.689268884208179, -6.7286546346820675, -6.716346198567756, -6.7456549250803635, -6.793305250625749, -6.776369910992359, -6.727919542131779, -6.643737304163345, -6.72330845447237, -6.762840576734769, -6.728860588338079, -6.7547328990229865, -6.804341984325519, -6.788695742046736, -6.628209614394328, -6.7071224164724015, -6.743027553407623, -6.706859116769193, -6.715448957373234, -6.58474249875318, -6.486435910417849, -6.645563912078905, -6.779086814441657, -6.6557890073334915, -6.682354875733151, -6.717902053687029, -6.639803234613179, -6.7392662344393015, -6.804426559970572, -6.901486104089262, -6.976476065486026, -6.811684507372176, -6.784855493192014, -6.914042819267215, -7.138490622274654, -7.147985781811261, -7.17896984010223, -7.158533342811933, -6.878657857531719, -6.953067233444325, -6.854320240892002, -6.849908073204693, -7.121245549605077, -7.155498235827838, -7.211542001154472, -6.938216843584059, -6.839598104389673, -7.270752397561136, -6.954400151067234, -6.783639622013585, -7.235012104942924, -7.012219571140947, -6.678865988943931, -7.217272626699833, -7.218877842424724, -6.81999845125471, -6.79903137402031, -6.757677277686154, -7.151873073097048, -7.243489462347358, -7.191556882387252, -6.769394897242261, -6.898269257265338, -7.168762942489076, -6.877880258424954, -6.807867815586103, -5.215817113668122, -5.971827084728676, -6.354818822995461, -6.728742048963516, -7.3134395509254935, -7.48138803327221, nan, nan, nan, -7.7356099437458425, -7.214792912117745, -6.927129142190539, -6.802121975139265, -7.7242965446392535, -7.178534250083907, -7.494256378549081, -9.706089974856223, -8.197381786330194, -7.887495891021734, -7.306689815244858, nan, -8.393503714553479, -6.92945227428538, -7.214689409139375, -7.421437399112728, -6.379785650707478, -6.288704968997288, -7.110410244318912, -7.033999863302572, -7.90540267794295, -7.387486306290954, -6.664515579597104, nan, nan, nan, nan, -7.21440086900962, -9.19841995587716, -7.298388924911925, -7.0107377266166795, -7.115510977505481, -6.743248665065608, nan, nan, -6.814683426746929, -6.680689032275566, -6.763396169407364, -7.431121033493272, -7.3919634009137924, nan, nan, -7.475268810668631, nan, nan, nan, nan, nan, -7.0253757817173295, -6.237048210058241, -7.4415539557268575, -7.345612214334548, -7.981405770636829, nan, nan, -6.741092536407123, -7.659217692822013, -6.797854926652502, nan, nan, nan, nan, nan, -6.181647882539599, -7.6962997739573975, -6.924699707914136, -6.428280425452268, -7.948150416754166, nan, nan, nan, -7.160196371581371, -6.684409828895361, nan, nan, -6.553681885488777, nan, nan, -7.743318588004079, -8.011277645187352, nan, nan, -7.349021366999787, nan, nan, -6.43777889010261, -7.432154245535317, nan, nan, -6.604563359277414, -6.2869034529791135, nan, -7.324770864464089, -7.538003639323684, -6.726761274308878, nan, nan, nan, -7.073871611914858, nan, nan, nan, nan, -8.054529169207957, nan, nan, -7.826743207082516, -7.485924982574887, nan, -8.178539334334072, nan, -7.450232617337361, nan, -7.338053388035876, nan, nan, nan, nan, nan, nan, nan, nan, nan, nan, nan, nan, nan, nan, nan, nan, nan, nan, nan, -7.352507714835287, -6.728447082486616, nan, nan, nan, nan, nan, nan, -7.554917054092685, -7.563154032406854, nan, nan, -7.795809101236794, nan, nan, nan, nan, nan, nan, nan, -7.709702113428104, -8.530020665207765, -8.218147279827184, nan, nan, nan, nan, nan, nan, nan, nan, nan, nan, nan, -5.5636441048421705, -7.859956203276619, -7.093171293035744, -7.7119948448198565, nan, nan, -6.902221719637082, -6.483175066541441, -6.07964723620741, nan, nan, nan, nan, nan, nan, nan, nan, nan, -8.010560185077477, nan, nan, nan, nan, nan, nan, nan, nan, nan, nan, nan, nan, nan, nan, nan, nan, nan, nan, nan, nan, nan, nan, nan, nan, nan, nan, nan, nan, -8.016301127150046, nan, nan, nan, nan, nan, nan, -6.104415956427648, -7.644304185816954, -7.784314455176924, nan, nan, nan, nan, nan, nan, nan, nan, nan, nan, -8.24113742062349, -7.240006895111019, -7.907909757115395, -8.05186208923642, nan, nan, nan, nan, -7.702865029263553, -9.24748744490411, nan, nan, nan, nan, -7.016742960376026, nan, nan, nan, nan, -7.4948810327872435, nan, nan, nan, nan, nan, nan, -7.886242509619053, nan, nan, nan, nan, nan, nan, -6.739532757108717, nan, nan, nan, nan, nan, nan, nan, nan, -9.340605125304167, nan, nan, nan, nan, nan, nan, nan, -7.449072053505574, nan, nan, nan, nan, nan, nan, -8.45107146001299, nan, nan, nan, nan, nan, -7.652389496071041, nan, nan, nan, nan, nan, -8.236349519985836, nan, nan, nan, -8.746136974199334, nan, nan, nan, -8.239750907734917, nan, nan, nan, nan, nan, -8.298879877613823, -9.875562065654941, nan, nan, nan, -8.180877596346638, nan, -7.320044755655616, nan, nan, nan, nan, nan, nan, nan, nan, nan, nan, nan, nan, nan, -7.9152186573270225, -8.41993205208269, nan, nan, nan, nan, nan, nan, nan, -8.255434669292468, -8.427694753620143, -9.496701810403387, nan, nan, nan, nan, nan, nan, -7.872733867729281, nan, nan, -8.703544935134733, -8.368491139959035, nan, nan, nan, nan, nan, nan, nan, nan, nan, nan, nan, nan, nan, nan, nan, nan, nan, nan, nan, nan, nan, -7.492330855999456, -8.916240882437338, nan, -9.976634894453156, nan, nan, nan, nan, nan, nan, nan, nan, nan, nan, nan, nan, nan, nan, nan, nan, nan, nan, nan, nan, -9.167391780327812, nan, nan, -7.780670055251402, nan, nan, nan, nan, nan, nan, nan, nan, nan, nan, nan, nan, nan, nan, -8.571541084375804, nan, nan, nan, -8.178952996214345, nan, nan, nan, nan, nan, nan, nan, nan, nan, nan, nan, nan, nan, nan, nan, 0.0, 0.0, 0.0]] caption="Water Vapor Number Density"
  out "CH3 RingBuffer short":dbl[][](array[numeric])=[[99.44, 31.439999999999998, 23.439999999999998, 27.439999999999998, 21.439999999999998, 14.44, 15.44, 44.44, 33.44, 38.44, 39.44, 40.44, 50.44, 72.44, 85.44, 99.44, 134.44, 134.44, 143.44, 170.44, 210.44, 171.44, 221.44, 210.44, 207.44, 228.44, 233.44, 215.44, 238.44, 217.44, 170.44, 197.44, 178.44, 224.44, 214.44, 192.44, 197.44, 204.44, 170.44, 194.44, 154.44, 160.44, 165.44, 163.44, 156.44, 155.44, 169.44, 150.44, 160.44, 150.44, 132.44, 144.44, 132.44, 133.44, 120.44, 123.44, 134.44, 114.44, 109.44, 132.44, 101.44, 102.44, 86.44, 88.44, 63.44, 76.44, 75.44, 76.44, 76.44, 40.44, 49.44, 64.44, 52.44, 36.44, 39.44, 28.439999999999998, 33.44, 65.44, 45.44, 41.44, 55.44, 35.44, 22.439999999999998, 30.439999999999998, 31.439999999999998, 28.439999999999998, 34.44, 38.44, 21.439999999999998, 38.44, 18.439999999999998, 41.44, 29.439999999999998, 33.44, 19.439999999999998, 27.439999999999998, 19.439999999999998, 14.44, 29.439999999999998, 21.439999999999998, 16.439999999999998, 23.439999999999998, 24.439999999999998, 20.439999999999998, 24.439999999999998, 11.44, 17.439999999999998, 15.44, 14.44, 14.44, 13.44, 8.44, 13.44, 13.44, 17.439999999999998, 13.44, 11.44, 10.44, 3.4399999999999995, 16.439999999999998, 9.44, 17.439999999999998, 13.44, 9.44, 21.439999999999998, 3.4399999999999995, 11.44, 5.4399999999999995, 11.44, 12.44, 22.439999999999998, 13.44, 16.439999999999998, 9.44, 2.4399999999999995, 18.439999999999998, 13.44, 10.44, 8.44, 7.4399999999999995, 12.44, 8.44, 6.4399999999999995, 7.4399999999999995, 7.4399999999999995, 2.4399999999999995, 0.4399999999999995, 10.44, 5.4399999999999995, 5.4399999999999995, 6.4399999999999995, -0.5600000000000005, 3.4399999999999995, 4.4399999999999995, -2.5600000000000005, 13.44, 8.44, 8.44, 4.4399999999999995, 5.4399999999999995, 7.4399999999999995, 3.4399999999999995, 7.4399999999999995, 9.44, 5.4399999999999995, 6.4399999999999995, 9.44, 9.44, 6.4399999999999995, 4.4399999999999995, 5.4399999999999995, 1.4399999999999995, 8.44, 7.4399999999999995, 7.4399999999999995, 8.44, 10.44, 3.4399999999999995, 7.4399999999999995, 2.4399999999999995, 7.4399999999999995, 2.4399999999999995, 4.4399999999999995, 7.4399999999999995, 2.4399999999999995, 4.4399999999999995, 8.44, 9.44, 6.4399999999999995, 5.4399999999999995, 4.4399999999999995, 1.4399999999999995, 1.4399999999999995, 4.4399999999999995, 5.4399999999999995, 8.44, 21.439999999999998, 1.4399999999999995, -1.5600000000000005, 9.44, 3.4399999999999995, 0.4399999999999995, 3.4399999999999995, 6.4399999999999995, 0.4399999999999995, 2.4399999999999995, 1.4399999999999995, 2.4399999999999995, 5.4399999999999995, 9.44, 6.4399999999999995, 6.4399999999999995, 7.4399999999999995, 3.4399999999999995, 4.4399999999999995, -2.5600000000000005, -2.5600000000000005, 1.4399999999999995, -0.5600000000000005, 3.4399999999999995, 5.4399999999999995, 3.4399999999999995, 1.4399999999999995, 5.4399999999999995, 1.4399999999999995, 2.4399999999999995, -8.56, 2.4399999999999995, -3.5600000000000005, 4.4399999999999995, 5.4399999999999995, -0.5600000000000005, -2.5600000000000005, 6.4399999999999995, 5.4399999999999995, 3.4399999999999995, -5.5600000000000005, 4.4399999999999995, 4.4399999999999995, -0.5600000000000005, 4.4399999999999995, 1.4399999999999995, -1.5600000000000005, -0.5600000000000005, 6.4399999999999995, -0.5600000000000005, 2.4399999999999995, -2.5600000000000005, -1.5600000000000005, -1.5600000000000005, -3.5600000000000005, 2.4399999999999995, 6.4399999999999995, -2.5600000000000005, 0.4399999999999995, -2.5600000000000005, 5.4399999999999995, 0.4399999999999995, -2.5600000000000005, 6.4399999999999995, -0.5600000000000005, -1.5600000000000005, -5.5600000000000005, -2.5600000000000005, 7.4399999999999995, 6.4399999999999995, -3.5600000000000005, 0.4399999999999995, 0.4399999999999995, -0.5600000000000005, -2.5600000000000005, -3.5600000000000005, -0.5600000000000005, -0.5600000000000005, 7.4399999999999995, 13.44, 15.44, 23.439999999999998, 21.439999999999998, 9.44, 7.4399999999999995, 11.44, 6.4399999999999995, 6.4399999999999995, 0.4399999999999995, 1.4399999999999995, 11.44, 25.439999999999998, 23.439999999999998, 16.439999999999998, 3.4399999999999995, -0.5600000000000005, 1.4399999999999995, -4.5600000000000005, 0.4399999999999995, -5.5600000000000005, 2.4399999999999995, 2.4399999999999995, 5.4399999999999995, -4.5600000000000005, -1.5600000000000005, 3.4399999999999995, 9.44, 0.4399999999999995, 6.4399999999999995, 0.4399999999999995, -0.5600000000000005, -0.5600000000000005, -4.5600000000000005, 1.4399999999999995, 3.4399999999999995, 4.4399999999999995, 2.4399999999999995, -1.5600000000000005, -2.5600000000000005, 7.4399999999999995, 7.4399999999999995, 1.4399999999999995, -1.5600000000000005, -4.5600000000000005, 2.4399999999999995, 0.4399999999999995, -1.5600000000000005, -3.5600000000000005, -1.5600000000000005, 3.4399999999999995, 2.4399999999999995, 8.44, -3.5600000000000005, -0.5600000000000005, -1.5600000000000005, 1.4399999999999995, -0.5600000000000005, 3.4399999999999995, -1.5600000000000005, 1.4399999999999995, 2.4399999999999995, -2.5600000000000005, 6.4399999999999995, 1.4399999999999995, 4.4399999999999995, 1.4399999999999995, -4.5600000000000005, 1.4399999999999995, 1.4399999999999995, -3.5600000000000005, 5.4399999999999995, 3.4399999999999995, 1.4399999999999995, 8.44, 5.4399999999999995, 14.44, -3.5600000000000005, 0.4399999999999995, -0.5600000000000005, 3.4399999999999995, 9.44, -2.5600000000000005, 2.4399999999999995, -6.5600000000000005, 1.4399999999999995, 5.4399999999999995, 0.4399999999999995, -0.5600000000000005, -0.5600000000000005, -5.5600000000000005, -0.5600000000000005, 0.4399999999999995, -2.5600000000000005, -0.5600000000000005, 7.4399999999999995, 8.44, -0.5600000000000005, -5.5600000000000005, -4.5600000000000005, 0.4399999999999995, -1.5600000000000005, -4.5600000000000005, -3.5600000000000005, -4.5600000000000005, -3.5600000000000005, 1.4399999999999995, 7.4399999999999995, -0.5600000000000005, 2.4399999999999995, -4.5600000000000005, 4.4399999999999995, -1.5600000000000005, 4.4399999999999995, 3.4399999999999995, -2.5600000000000005, 3.4399999999999995, 4.4399999999999995, 1.4399999999999995, 10.44, 4.4399999999999995, 0.4399999999999995, 1.4399999999999995, -3.5600000000000005, 7.4399999999999995, 7.4399999999999995, -1.5600000000000005, -5.5600000000000005, -5.5600000000000005, 5.4399999999999995, -0.5600000000000005, -3.5600000000000005, 5.4399999999999995, 1.4399999999999995, 4.4399999999999995, 5.4399999999999995, -0.5600000000000005, 2.4399999999999995, 2.4399999999999995, -3.5600000000000005, 8.44, 5.4399999999999995, 3.4399999999999995, -1.5600000000000005, 6.4399999999999995, 0.4399999999999995, 3.4399999999999995, -2.5600000000000005, -1.5600000000000005, -4.5600000000000005, -2.5600000000000005, 4.4399999999999995, -1.5600000000000005, 5.4399999999999995, 0.4399999999999995, 5.4399999999999995, 11.44, -1.5600000000000005, 5.4399999999999995, 1.4399999999999995, -2.5600000000000005, -4.5600000000000005, -1.5600000000000005, -0.5600000000000005, 4.4399999999999995, 2.4399999999999995, -3.5600000000000005, 4.4399999999999995, -3.5600000000000005, -0.5600000000000005, 0.4399999999999995, 0.4399999999999995, 7.4399999999999995, 10.44, 5.4399999999999995, -0.5600000000000005, 4.4399999999999995, 3.4399999999999995, -1.5600000000000005, -3.5600000000000005, 5.4399999999999995, 1.4399999999999995, 6.4399999999999995, 4.4399999999999995, 2.4399999999999995, -0.5600000000000005, 1.4399999999999995, 1.4399999999999995, 6.4399999999999995, -1.5600000000000005, -4.5600000000000005, 1.4399999999999995, -2.5600000000000005, -4.5600000000000005, -2.5600000000000005, -4.5600000000000005, -2.5600000000000005, -0.5600000000000005, 3.4399999999999995, 2.4399999999999995, 3.4399999999999995, 4.4399999999999995, 0.4399999999999995, 1.4399999999999995, 6.4399999999999995, -3.5600000000000005, 1.4399999999999995, -2.5600000000000005, 2.4399999999999995, -5.5600000000000005, 0.4399999999999995, 0.4399999999999995, -2.5600000000000005, 1.4399999999999995, -1.5600000000000005, -3.5600000000000005, 5.4399999999999995, 5.4399999999999995, 4.4399999999999995, 2.4399999999999995, -0.5600000000000005, 5.4399999999999995, -2.5600000000000005, -0.5600000000000005, -3.5600000000000005, -0.5600000000000005, 4.4399999999999995, 1.4399999999999995, -1.5600000000000005, -4.5600000000000005, -3.5600000000000005, -2.5600000000000005, -3.5600000000000005, 2.4399999999999995, -2.5600000000000005, -2.5600000000000005, -4.5600000000000005, 3.4399999999999995, -2.5600000000000005, -1.5600000000000005, -1.5600000000000005, 4.4399999999999995, 7.4399999999999995, -2.5600000000000005, 1.4399999999999995, -3.5600000000000005, -4.5600000000000005, -4.5600000000000005, 2.4399999999999995, 3.4399999999999995, -8.56, 7.4399999999999995, 6.4399999999999995, 1.4399999999999995, 3.4399999999999995, -4.5600000000000005, -1.5600000000000005, 9.44, 2.4399999999999995, -0.5600000000000005, -0.5600000000000005, 2.4399999999999995, -6.5600000000000005, -4.5600000000000005, -3.5600000000000005, 2.4399999999999995, 0.4399999999999995, 5.4399999999999995, 2.4399999999999995, -1.5600000000000005, -2.5600000000000005, -3.5600000000000005, 0.4399999999999995, -1.5600000000000005, -1.5600000000000005, 4.4399999999999995, 2.4399999999999995, -0.5600000000000005, 0.4399999999999995, -1.5600000000000005, 2.4399999999999995, 7.4399999999999995, -5.5600000000000005, 3.4399999999999995], [99.44, 31.439999999999998, 23.439999999999998, 27.439999999999998, 21.439999999999998, 14.44, 15.44, 44.44, 33.44, 38.44, 39.44, 40.44, 50.44, 72.44, 85.44, 99.44, 134.44, 134.44, 143.44, 170.44, 210.44, 171.44, 221.44, 210.44, 207.44, 228.44, 233.44, 215.44, 238.44, 217.44, 170.44, 197.44, 178.44, 224.44, 214.44, 192.44, 197.44, 204.44, 170.44, 194.44, 154.44, 160.44, 165.44, 163.44, 156.44, 155.44, 169.44, 150.44, 160.44, 150.44, 132.44, 144.44, 132.44, 133.44, 120.44, 123.44, 134.44, 114.44, 109.44, 132.44, 101.44, 102.44, 86.44, 88.44, 63.44, 76.44, 75.44, 76.44, 76.44, 40.44, 49.44, 64.44, 52.44, 36.44, 39.44, 28.439999999999998, 33.44, 65.44, 45.44, 41.44, 55.44, 35.44, 22.439999999999998, 30.439999999999998, 31.439999999999998, 28.439999999999998, 34.44, 38.44, 21.439999999999998, 38.44, 18.439999999999998, 41.44, 29.439999999999998, 33.44, 19.439999999999998, 27.439999999999998, 19.439999999999998, 14.44, 29.439999999999998, 21.439999999999998, 16.439999999999998, 23.439999999999998, 24.439999999999998, 20.439999999999998, 24.439999999999998, 11.44, 17.439999999999998, 15.44, 14.44, 14.44, 13.44, 8.44, 13.44, 13.44, 17.439999999999998, 13.44, 11.44, 10.44, 3.4399999999999995, 16.439999999999998, 9.44, 17.439999999999998, 13.44, 9.44, 21.439999999999998, 3.4399999999999995, 11.44, 5.4399999999999995, 11.44, 12.44, 22.439999999999998, 13.44, 16.439999999999998, 9.44, 2.4399999999999995, 18.439999999999998, 13.44, 10.44, 8.44, 7.4399999999999995, 12.44, 8.44, 6.4399999999999995, 7.4399999999999995, 7.4399999999999995, 2.4399999999999995, 0.4399999999999995, 10.44, 5.4399999999999995, 5.4399999999999995, 6.4399999999999995, -0.5600000000000005, 3.4399999999999995, 4.4399999999999995, -2.5600000000000005, 13.44, 8.44, 8.44, 4.4399999999999995, 5.4399999999999995, 7.4399999999999995, 3.4399999999999995, 7.4399999999999995, 9.44, 5.4399999999999995, 6.4399999999999995, 9.44, 9.44, 6.4399999999999995, 4.4399999999999995, 5.4399999999999995, 1.4399999999999995, 8.44, 7.4399999999999995, 7.4399999999999995, 8.44, 10.44, 3.4399999999999995, 7.4399999999999995, 2.4399999999999995, 7.4399999999999995, 2.4399999999999995, 4.4399999999999995, 7.4399999999999995, 2.4399999999999995, 4.4399999999999995, 8.44, 9.44, 6.4399999999999995, 5.4399999999999995, 4.4399999999999995, 1.4399999999999995, 1.4399999999999995, 4.4399999999999995, 5.4399999999999995, 8.44, 21.439999999999998, 1.4399999999999995, -1.5600000000000005, 9.44, 3.4399999999999995, 0.4399999999999995, 3.4399999999999995, 6.4399999999999995, 0.4399999999999995, 2.4399999999999995, 1.4399999999999995, 2.4399999999999995, 5.4399999999999995, 9.44, 6.4399999999999995, 6.4399999999999995, 7.4399999999999995, 3.4399999999999995, 4.4399999999999995, -2.5600000000000005, -2.5600000000000005, 1.4399999999999995, -0.5600000000000005, 3.4399999999999995, 5.4399999999999995, 3.4399999999999995, 1.4399999999999995, 5.4399999999999995, 1.4399999999999995, 2.4399999999999995, -8.56, 2.4399999999999995, -3.5600000000000005, 4.4399999999999995, 5.4399999999999995, -0.5600000000000005, -2.5600000000000005, 6.4399999999999995, 5.4399999999999995, 3.4399999999999995, -5.5600000000000005, 4.4399999999999995, 4.4399999999999995, -0.5600000000000005, 4.4399999999999995, 1.4399999999999995, -1.5600000000000005, -0.5600000000000005, 6.4399999999999995, -0.5600000000000005, 2.4399999999999995, -2.5600000000000005, -1.5600000000000005, -1.5600000000000005, -3.5600000000000005, 2.4399999999999995, 6.4399999999999995, -2.5600000000000005, 0.4399999999999995, -2.5600000000000005, 5.4399999999999995, 0.4399999999999995, -2.5600000000000005, 6.4399999999999995, -0.5600000000000005, -1.5600000000000005, -5.5600000000000005, -2.5600000000000005, 7.4399999999999995, 6.4399999999999995, -3.5600000000000005, 0.4399999999999995, 0.4399999999999995, -0.5600000000000005, -2.5600000000000005, -3.5600000000000005, -0.5600000000000005, -0.5600000000000005, 7.4399999999999995, 13.44, 15.44, 23.439999999999998, 21.439999999999998, 9.44, 7.4399999999999995, 11.44, 6.4399999999999995, 6.4399999999999995, 0.4399999999999995, 1.4399999999999995, 11.44, 25.439999999999998, 23.439999999999998, 16.439999999999998, 3.4399999999999995, -0.5600000000000005, 1.4399999999999995, -4.5600000000000005, 0.4399999999999995, -5.5600000000000005, 2.4399999999999995, 2.4399999999999995, 5.4399999999999995, -4.5600000000000005, -1.5600000000000005, 3.4399999999999995, 9.44, 0.4399999999999995, 6.4399999999999995, 0.4399999999999995, -0.5600000000000005, -0.5600000000000005, -4.5600000000000005, 1.4399999999999995, 3.4399999999999995, 4.4399999999999995, 2.4399999999999995, -1.5600000000000005, -2.5600000000000005, 7.4399999999999995, 7.4399999999999995, 1.4399999999999995, -1.5600000000000005, -4.5600000000000005, 2.4399999999999995, 0.4399999999999995, -1.5600000000000005, -3.5600000000000005, -1.5600000000000005, 3.4399999999999995, 2.4399999999999995, 8.44, -3.5600000000000005, -0.5600000000000005, -1.5600000000000005, 1.4399999999999995, -0.5600000000000005, 3.4399999999999995, -1.5600000000000005, 1.4399999999999995, 2.4399999999999995, -2.5600000000000005, 6.4399999999999995, 1.4399999999999995, 4.4399999999999995, 1.4399999999999995, -4.5600000000000005, 1.4399999999999995, 1.4399999999999995, -3.5600000000000005, 5.4399999999999995, 3.4399999999999995, 1.4399999999999995, 8.44, 5.4399999999999995, 14.44, -3.5600000000000005, 0.4399999999999995, -0.5600000000000005, 3.4399999999999995, 9.44, -2.5600000000000005, 2.4399999999999995, -6.5600000000000005, 1.4399999999999995, 5.4399999999999995, 0.4399999999999995, -0.5600000000000005, -0.5600000000000005, -5.5600000000000005, -0.5600000000000005, 0.4399999999999995, -2.5600000000000005, -0.5600000000000005, 7.4399999999999995, 8.44, -0.5600000000000005, -5.5600000000000005, -4.5600000000000005, 0.4399999999999995, -1.5600000000000005, -4.5600000000000005, -3.5600000000000005, -4.5600000000000005, -3.5600000000000005, 1.4399999999999995, 7.4399999999999995, -0.5600000000000005, 2.4399999999999995, -4.5600000000000005, 4.4399999999999995, -1.5600000000000005, 4.4399999999999995, 3.4399999999999995, -2.5600000000000005, 3.4399999999999995, 4.4399999999999995, 1.4399999999999995, 10.44, 4.4399999999999995, 0.4399999999999995, 1.4399999999999995, -3.5600000000000005, 7.4399999999999995, 7.4399999999999995, -1.5600000000000005, -5.5600000000000005, -5.5600000000000005, 5.4399999999999995, -0.5600000000000005, -3.5600000000000005, 5.4399999999999995, 1.4399999999999995, 4.4399999999999995, 5.4399999999999995, -0.5600000000000005, 2.4399999999999995, 2.4399999999999995, -3.5600000000000005, 8.44, 5.4399999999999995, 3.4399999999999995, -1.5600000000000005, 6.4399999999999995, 0.4399999999999995, 3.4399999999999995, -2.5600000000000005, -1.5600000000000005, -4.5600000000000005, -2.5600000000000005, 4.4399999999999995, -1.5600000000000005, 5.4399999999999995, 0.4399999999999995, 5.4399999999999995, 11.44, -1.5600000000000005, 5.4399999999999995, 1.4399999999999995, -2.5600000000000005, -4.5600000000000005, -1.5600000000000005, -0.5600000000000005, 4.4399999999999995, 2.4399999999999995, -3.5600000000000005, 4.4399999999999995, -3.5600000000000005, -0.5600000000000005, 0.4399999999999995, 0.4399999999999995, 7.4399999999999995, 10.44, 5.4399999999999995, -0.5600000000000005, 4.4399999999999995, 3.4399999999999995, -1.5600000000000005, -3.5600000000000005, 5.4399999999999995, 1.4399999999999995, 6.4399999999999995, 4.4399999999999995, 2.4399999999999995, -0.5600000000000005, 1.4399999999999995, 1.4399999999999995, 6.4399999999999995, -1.5600000000000005, -4.5600000000000005, 1.4399999999999995, -2.5600000000000005, -4.5600000000000005, -2.5600000000000005, -4.5600000000000005, -2.5600000000000005, -0.5600000000000005, 3.4399999999999995, 2.4399999999999995, 3.4399999999999995, 4.4399999999999995, 0.4399999999999995, 1.4399999999999995, 6.4399999999999995, -3.5600000000000005, 1.4399999999999995, -2.5600000000000005, 2.4399999999999995, -5.5600000000000005, 0.4399999999999995, 0.4399999999999995, -2.5600000000000005, 1.4399999999999995, -1.5600000000000005, -3.5600000000000005, 5.4399999999999995, 5.4399999999999995, 4.4399999999999995, 2.4399999999999995, -0.5600000000000005, 5.4399999999999995, -2.5600000000000005, -0.5600000000000005, -3.5600000000000005, -0.5600000000000005, 4.4399999999999995, 1.4399999999999995, -1.5600000000000005, -4.5600000000000005, -3.5600000000000005, -2.5600000000000005, -3.5600000000000005, 2.4399999999999995, -2.5600000000000005, -2.5600000000000005, -4.5600000000000005, 3.4399999999999995, -2.5600000000000005, -1.5600000000000005, -1.5600000000000005, 4.4399999999999995, 7.4399999999999995, -2.5600000000000005, 1.4399999999999995, -3.5600000000000005, -4.5600000000000005, -4.5600000000000005, 2.4399999999999995, 3.4399999999999995, -8.56, 7.4399999999999995, 6.4399999999999995, 1.4399999999999995, 3.4399999999999995, -4.5600000000000005, -1.5600000000000005, 9.44, 2.4399999999999995, -0.5600000000000005, -0.5600000000000005, 2.4399999999999995, -6.5600000000000005, -4.5600000000000005, -3.5600000000000005, 2.4399999999999995, 0.4399999999999995, 5.4399999999999995, 2.4399999999999995, -1.5600000000000005, -2.5600000000000005, -3.5600000000000005, 0.4399999999999995, -1.5600000000000005, -1.5600000000000005, 4.4399999999999995, 2.4399999999999995, -0.5600000000000005, 0.4399999999999995, -1.5600000000000005, 2.4399999999999995, 7.4399999999999995, -5.5600000000000005, 3.4399999999999995], [91.88, 21.880000000000003, 26.880000000000003, 31.880000000000003, 26.880000000000003, 19.880000000000003, 18.880000000000003, 34.88, 20.880000000000003, 32.88, 23.880000000000003, 30.880000000000003, 70.88, 60.88, 67.88, 74.88, 89.88, 118.88, 150.88, 171.88, 171.88, 198.88, 194.88, 191.88, 186.88, 196.88, 198.88, 213.88, 213.88, 187.88, 192.88, 184.88, 187.88, 213.88, 224.88, 208.88, 188.88, 199.88, 200.88, 199.88, 179.88, 170.88, 158.88, 188.88, 180.88, 160.88, 152.88, 158.88, 148.88, 140.88, 169.88, 137.88, 133.88, 137.88, 123.88, 120.88, 136.88, 114.88, 95.88, 115.88, 111.88, 91.88, 108.88, 88.88, 80.88, 98.88, 97.88, 66.88, 68.88, 64.88, 71.88, 68.88, 57.88, 36.88, 57.88, 58.88, 49.88, 37.88, 56.88, 41.88, 34.88, 40.88, 35.88, 28.880000000000003, 32.88, 30.880000000000003, 31.880000000000003, 38.88, 39.88, 30.880000000000003, 30.880000000000003, 32.88, 42.88, 27.880000000000003, 33.88, 44.88, 37.88, 36.88, 25.880000000000003, 20.880000000000003, 21.880000000000003, 26.880000000000003, 20.880000000000003, 23.880000000000003, 15.88, 21.880000000000003, 11.88, 13.88, 27.880000000000003, 13.88, 17.880000000000003, 14.88, 7.880000000000001, 19.880000000000003, 15.88, 18.880000000000003, 4.880000000000001, 4.880000000000001, 15.88, 5.880000000000001, 2.880000000000001, 9.88, 10.88, 16.880000000000003, 15.88, 6.880000000000001, 6.880000000000001, 9.88, 9.88, 1.8800000000000008, 15.88, 9.88, 22.880000000000003, 15.88, 10.88, 12.88, 14.88, 7.880000000000001, 5.880000000000001, 12.88, 3.880000000000001, 2.880000000000001, 7.880000000000001, 10.88, 12.88, 9.88, 7.880000000000001, 11.88, 4.880000000000001, 8.88, 6.880000000000001, 11.88, 20.880000000000003, 12.88, 15.88, 4.880000000000001, 8.88, 13.88, 11.88, 2.880000000000001, 3.880000000000001, 6.880000000000001, 5.880000000000001, 6.880000000000001, 5.880000000000001, 4.880000000000001, 0.8800000000000008, 5.880000000000001, 2.880000000000001, 5.880000000000001, 4.880000000000001, -2.119999999999999, 3.880000000000001, 10.88, 5.880000000000001, 2.880000000000001, 6.880000000000001, 6.880000000000001, 7.880000000000001, 14.88, 2.880000000000001, 0.8800000000000008, -4.119999999999999, -2.119999999999999, -3.119999999999999, 20.880000000000003, 3.880000000000001, 1.8800000000000008, 11.88, 4.880000000000001, 2.880000000000001, 1.8800000000000008, 12.88, -4.119999999999999, 1.8800000000000008, 2.880000000000001, 5.880000000000001, 5.880000000000001, -2.119999999999999, 6.880000000000001, 2.880000000000001, 1.8800000000000008, 3.880000000000001, 5.880000000000001, -0.11999999999999922, 1.8800000000000008, 11.88, -5.119999999999999, -1.1199999999999992, 6.880000000000001, 4.880000000000001, -3.119999999999999, 8.88, 6.880000000000001, -2.119999999999999, -1.1199999999999992, 3.880000000000001, 8.88, 1.8800000000000008, 5.880000000000001, -1.1199999999999992, 1.8800000000000008, 11.88, -1.1199999999999992, -0.11999999999999922, 8.88, -4.119999999999999, 0.8800000000000008, -0.11999999999999922, 4.880000000000001, 2.880000000000001, 0.8800000000000008, -1.1199999999999992, 8.88, 4.880000000000001, -2.119999999999999, 1.8800000000000008, -0.11999999999999922, 2.880000000000001, 6.880000000000001, 3.880000000000001, 8.88, -2.119999999999999, 1.8800000000000008, 2.880000000000001, 2.880000000000001, 1.8800000000000008, 12.88, 5.880000000000001, 1.8800000000000008, 1.8800000000000008, 1.8800000000000008, 7.880000000000001, 2.880000000000001, 5.880000000000001, 2.880000000000001, 4.880000000000001, -2.119999999999999, -0.11999999999999922, 1.8800000000000008, 4.880000000000001, 3.880000000000001, 4.880000000000001, 1.8800000000000008, -3.119999999999999, 1.8800000000000008, 4.880000000000001, 4.880000000000001, 8.88, 5.880000000000001, 4.880000000000001, 1.8800000000000008, 0.8800000000000008, -2.119999999999999, 5.880000000000001, 11.88, 21.880000000000003, 20.880000000000003, 21.880000000000003, 15.88, 3.880000000000001, -0.11999999999999922, 4.880000000000001, 5.880000000000001, 9.88, 6.880000000000001, 23.880000000000003, 9.88, 16.880000000000003, 18.880000000000003, 2.880000000000001, 3.880000000000001, 4.880000000000001, 7.880000000000001, -0.11999999999999922, -5.119999999999999, -0.11999999999999922, 0.8800000000000008, 5.880000000000001, -0.11999999999999922, 6.880000000000001, -0.11999999999999922, -1.1199999999999992, 5.880000000000001, -0.11999999999999922, 2.880000000000001, 1.8800000000000008, -2.119999999999999, -1.1199999999999992, 0.8800000000000008, -0.11999999999999922, -2.119999999999999, -0.11999999999999922, 8.88, 2.880000000000001, -0.11999999999999922, -1.1199999999999992, -0.11999999999999922, 4.880000000000001, 4.880000000000001, 1.8800000000000008, 1.8800000000000008, 9.88, -1.1199999999999992, -0.11999999999999922, 1.8800000000000008, 1.8800000000000008, -1.1199999999999992, 8.88, 5.880000000000001, 5.880000000000001, -5.119999999999999, 0.8800000000000008, 1.8800000000000008, 8.88, 9.88, 5.880000000000001, 4.880000000000001, 0.8800000000000008, -4.119999999999999, -3.119999999999999, -0.11999999999999922, -0.11999999999999922, -0.11999999999999922, -0.11999999999999922, 2.880000000000001, -2.119999999999999, 1.8800000000000008, 1.8800000000000008, 4.880000000000001, 1.8800000000000008, 6.880000000000001, -2.119999999999999, 0.8800000000000008, 3.880000000000001, 8.88, -0.11999999999999922, 6.880000000000001, 1.8800000000000008, 2.880000000000001, 6.880000000000001, -1.1199999999999992, -1.1199999999999992, 3.880000000000001, -4.119999999999999, 4.880000000000001, 2.880000000000001, -4.119999999999999, -3.119999999999999, 5.880000000000001, 0.8800000000000008, -3.119999999999999, 5.880000000000001, -3.119999999999999, -0.11999999999999922, 5.880000000000001, 2.880000000000001, 7.880000000000001, -0.11999999999999922, 0.8800000000000008, 6.880000000000001, 10.88, 1.8800000000000008, -1.1199999999999992, -6.119999999999999, -1.1199999999999992, -1.1199999999999992, -0.11999999999999922, -2.119999999999999, 5.880000000000001, 1.8800000000000008, 3.880000000000001, -3.119999999999999, -5.119999999999999, -4.119999999999999, -0.11999999999999922, 2.880000000000001, -2.119999999999999, 0.8800000000000008, -4.119999999999999, 4.880000000000001, -0.11999999999999922, 1.8800000000000008, -1.1199999999999992, -2.119999999999999, 5.880000000000001, 2.880000000000001, 0.8800000000000008, 0.8800000000000008, 1.8800000000000008, 4.880000000000001, 5.880000000000001, 2.880000000000001, 0.8800000000000008, -3.119999999999999, -0.11999999999999922, -0.11999999999999922, 0.8800000000000008, -2.119999999999999, -1.1199999999999992, -1.1199999999999992, -3.119999999999999, -1.1199999999999992, -0.11999999999999922, -1.1199999999999992, -0.11999999999999922, -3.119999999999999, -2.119999999999999, 0.8800000000000008, -5.119999999999999, 5.880000000000001, 0.8800000000000008, -1.1199999999999992, 7.880000000000001, -0.11999999999999922, -1.1199999999999992, -2.119999999999999, 0.8800000000000008, -0.11999999999999922, 0.8800000000000008, 1.8800000000000008, 6.880000000000001, 2.880000000000001, 4.880000000000001, 0.8800000000000008, 1.8800000000000008, -0.11999999999999922, -6.119999999999999, -1.1199999999999992, -4.119999999999999, -2.119999999999999, -0.11999999999999922, 0.8800000000000008, 1.8800000000000008, -3.119999999999999, -1.1199999999999992, -1.1199999999999992, 2.880000000000001, -5.119999999999999, 0.8800000000000008, 4.880000000000001, 0.8800000000000008, 0.8800000000000008, -1.1199999999999992, -1.1199999999999992, -1.1199999999999992, 1.8800000000000008, -1.1199999999999992, 4.880000000000001, -0.11999999999999922, 4.880000000000001, 4.880000000000001, 0.8800000000000008, 2.880000000000001, 2.880000000000001, -4.119999999999999, -1.1199999999999992, 2.880000000000001, -1.1199999999999992, 0.8800000000000008, -6.119999999999999, 5.880000000000001, -4.119999999999999, -3.119999999999999, -4.119999999999999, 5.880000000000001, 0.8800000000000008, 4.880000000000001, -3.119999999999999, 4.880000000000001, 0.8800000000000008, 6.880000000000001, 0.8800000000000008, -2.119999999999999, -1.1199999999999992, 3.880000000000001, 0.8800000000000008, 4.880000000000001, -2.119999999999999, -6.119999999999999, 3.880000000000001, -0.11999999999999922, -2.119999999999999, -1.1199999999999992, -0.11999999999999922, -3.119999999999999, -3.119999999999999, -3.119999999999999, -0.11999999999999922, -1.1199999999999992, -0.11999999999999922, -2.119999999999999, 7.880000000000001, -1.1199999999999992, 2.880000000000001, 2.880000000000001, 1.8800000000000008, -0.11999999999999922, -3.119999999999999, -1.1199999999999992, -3.119999999999999, 1.8800000000000008, 2.880000000000001, 3.880000000000001, -0.11999999999999922, 4.880000000000001, -0.11999999999999922, -0.11999999999999922, -1.1199999999999992, 4.880000000000001, -0.11999999999999922, -1.1199999999999992, -1.1199999999999992, 4.880000000000001, 0.8800000000000008, 1.8800000000000008, 0.8800000000000008, -4.119999999999999, -6.119999999999999, 0.8800000000000008, 0.8800000000000008, 2.880000000000001, 1.8800000000000008, -3.119999999999999, -2.119999999999999, 3.880000000000001, -3.119999999999999, -1.1199999999999992, -0.11999999999999922, -1.1199999999999992, -0.11999999999999922, 0.8800000000000008, -4.119999999999999, 8.88, -2.119999999999999, 0.8800000000000008, 0.8800000000000008, 1.8800000000000008, -0.11999999999999922], [80.24, 29.240000000000002, 27.240000000000002, 29.240000000000002, 24.240000000000002, 33.24, 30.240000000000002, 33.24, 23.240000000000002, 30.240000000000002, 37.24, 43.24, 59.24, 67.24, 86.24, 83.24, 113.24, 127.24, 154.24, 156.24, 180.24, 153.24, 211.24, 213.24, 233.24, 242.24, 214.24, 198.24, 210.24, 192.24, 177.24, 212.24, 223.24, 220.24, 190.24, 207.24, 186.24, 190.24, 198.24, 180.24, 174.24, 182.24, 164.24, 179.24, 176.24, 153.24, 154.24, 143.24, 117.24, 136.24, 134.24, 137.24, 109.24, 118.24, 101.24, 125.24, 117.24, 108.24, 124.24, 107.24, 111.24, 68.24, 84.24, 84.24, 102.24, 65.24, 54.24, 74.24, 64.24, 60.24, 46.24, 67.24, 41.24, 48.24, 43.24, 51.24, 52.24, 46.24, 43.24, 46.24, 45.24, 43.24, 41.24, 37.24, 49.24, 26.240000000000002, 31.240000000000002, 30.240000000000002, 20.240000000000002, 20.240000000000002, 30.240000000000002, 27.240000000000002, 17.240000000000002, 32.24, 18.240000000000002, 23.240000000000002, 29.240000000000002, 14.24, 30.240000000000002, 22.240000000000002, 20.240000000000002, 19.240000000000002, 27.240000000000002, 23.240000000000002, 17.240000000000002, 14.24, 20.240000000000002, 18.240000000000002, 11.24, 17.240000000000002, 9.24, 9.24, 12.24, 16.240000000000002, 10.24, 9.24, 13.24, 11.24, 13.24, 16.240000000000002, 5.24, 14.24, 14.24, 9.24, 11.24, 11.24, 9.24, 14.24, 14.24, 8.24, 23.240000000000002, 11.24, 10.24, 6.24, 7.24, 6.24, 20.240000000000002, 15.24, 4.24, 12.24, 9.24, 6.24, 10.24, 9.24, 7.24, 11.24, 9.24, 5.24, 8.24, 5.24, 5.24, -2.76, 6.24, 17.240000000000002, 5.24, 4.24, 2.24, -2.76, -3.76, 13.24, 5.24, 7.24, 6.24, -1.7599999999999998, 4.24, 13.24, 2.24, 8.24, 9.24, 9.24, 4.24, 13.24, 0.2400000000000002, 8.24, 6.24, 2.24, 9.24, 11.24, 3.24, 5.24, 6.24, 0.2400000000000002, 11.24, -1.7599999999999998, 3.24, 5.24, 3.24, 4.24, -6.76, 6.24, 4.24, 1.2400000000000002, -0.7599999999999998, 8.24, -2.76, 1.2400000000000002, 0.2400000000000002, 2.24, 12.24, 8.24, 1.2400000000000002, 0.2400000000000002, 3.24, 6.24, -2.76, 9.24, 1.2400000000000002, 5.24, 2.24, 5.24, 3.24, -1.7599999999999998, -1.7599999999999998, 2.24, -1.7599999999999998, 0.2400000000000002, 8.24, 6.24, 3.24, 3.24, 6.24, -1.7599999999999998, 0.2400000000000002, -0.7599999999999998, 5.24, 10.24, 2.24, -0.7599999999999998, 3.24, 2.24, 9.24, 3.24, -5.76, 3.24, 7.24, -4.76, 8.24, -3.76, -2.76, 10.24, -7.76, -7.76, 7.24, -0.7599999999999998, 2.24, -0.7599999999999998, 0.2400000000000002, 5.24, -3.76, 10.24, -5.76, 6.24, 5.24, 12.24, 2.24, 4.24, -1.7599999999999998, -0.7599999999999998, -2.76, 8.24, 3.24, 6.24, 6.24, 7.24, -1.7599999999999998, -1.7599999999999998, 6.24, 2.24, 9.24, -3.76, -0.7599999999999998, -2.76, 4.24, 6.24, 1.2400000000000002, 14.24, 24.240000000000002, 20.240000000000002, 19.240000000000002, 15.24, 0.2400000000000002, 4.24, 3.24, 1.2400000000000002, 10.24, -8.76, 10.24, 15.24, 21.240000000000002, 20.240000000000002, 7.24, 4.24, -4.76, 0.2400000000000002, -5.76, 11.24, -2.76, 0.2400000000000002, 0.2400000000000002, 6.24, 5.24, 8.24, 4.24, -1.7599999999999998, 1.2400000000000002, 2.24, 2.24, 6.24, 6.24, -1.7599999999999998, -1.7599999999999998, 0.2400000000000002, -6.76, 5.24, 5.24, 4.24, -3.76, 1.2400000000000002, 4.24, -1.7599999999999998, 7.24, -1.7599999999999998, 0.2400000000000002, 2.24, -4.76, 1.2400000000000002, 3.24, 2.24, -2.76, -0.7599999999999998, -4.76, 0.2400000000000002, -0.7599999999999998, -0.7599999999999998, -2.76, 4.24, 1.2400000000000002, 2.24, -1.7599999999999998, -2.76, 6.24, 7.24, -8.76, 2.24, 1.2400000000000002, 1.2400000000000002, 4.24, 2.24, 12.24, 1.2400000000000002, 1.2400000000000002, -6.76, 0.2400000000000002, 4.24, 0.2400000000000002, 3.24, 4.24, -0.7599999999999998, 2.24, 8.24, 1.2400000000000002, -1.7599999999999998, 6.24, 2.24, -5.76, 0.2400000000000002, 7.24, 0.2400000000000002, 4.24, 4.24, 5.24, -4.76, -4.76, -4.76, -0.7599999999999998, -4.76, 6.24, 5.24, -4.76, 5.24, -0.7599999999999998, -5.76, 0.2400000000000002, 0.2400000000000002, 9.24, 0.2400000000000002, -1.7599999999999998, 8.24, -5.76, 0.2400000000000002, -3.76, 8.24, 3.24, 3.24, -2.76, 2.24, -1.7599999999999998, -2.76, -7.76, 1.2400000000000002, -0.7599999999999998, 7.24, 1.2400000000000002, 2.24, 1.2400000000000002, 2.24, -0.7599999999999998, 2.24, -3.76, 3.24, 7.24, 1.2400000000000002, -5.76, 4.24, -2.76, 4.24, -1.7599999999999998, 6.24, -5.76, -3.76, 0.2400000000000002, 3.24, 2.24, -1.7599999999999998, 4.24, -1.7599999999999998, 3.24, 9.24, 2.24, -3.76, 2.24, 2.24, 11.24, 4.24, 2.24, 1.2400000000000002, -0.7599999999999998, -2.76, -0.7599999999999998, 0.2400000000000002, -5.76, -2.76, -5.76, -4.76, 1.2400000000000002, 7.24, 0.2400000000000002, 10.24, -0.7599999999999998, -5.76, 3.24, -2.76, 3.24, -4.76, 5.24, -2.76, 4.24, -0.7599999999999998, 8.24, -1.7599999999999998, 3.24, 3.24, 3.24, 4.24, 0.2400000000000002, 4.24, -1.7599999999999998, -3.76, 5.24, 1.2400000000000002, 0.2400000000000002, 4.24, 1.2400000000000002, 10.24, 0.2400000000000002, -1.7599999999999998, 0.2400000000000002, 5.24, -0.7599999999999998, 5.24, -3.76, -0.7599999999999998, -5.76, -2.76, 4.24, 1.2400000000000002, 8.24, 0.2400000000000002, -6.76, 1.2400000000000002, -5.76, -5.76, 7.24, 2.24, 7.24, -1.7599999999999998, 3.24, 3.24, 5.24, -4.76, 0.2400000000000002, -0.7599999999999998, -7.76, 8.24, 1.2400000000000002, 3.24, -3.76, 2.24, 8.24, -2.76, 5.24, 5.24, -0.7599999999999998, 5.24, -0.7599999999999998, 4.24, 2.24, 4.24, 2.24, 0.2400000000000002, 2.24, 1.2400000000000002, 0.2400000000000002, -8.76, 3.24, 5.24, 7.24, 3.24, 0.2400000000000002, 7.24, -3.76, 1.2400000000000002, 3.24, 2.24, 2.24, -0.7599999999999998, -1.7599999999999998, 1.2400000000000002, -6.76, -2.76, 0.2400000000000002, 5.24, 5.24, 3.24, -2.76, 5.24, -0.7599999999999998, -0.7599999999999998, 1.2400000000000002, 4.24, -1.7599999999999998, 3.24, -0.7599999999999998, 0.2400000000000002, -5.76, 2.24, -4.76, 0.2400000000000002, -4.76]]
  in  "?":T1(tab)
  out "NRB WV Offline":dbl[][](graph)=[[7.967208445594253e-06, 3.0697958718715426e-05, 6.951608509367255e-05, 0.00012986993455436322, 0.000216842841535583, 0.000337926540973799, 0.0005076815861465128, 0.0007426918459880069, 0.001092430102179687, 0.0015123713611379075, 0.0019892882707577423, 0.0026390033654037216, 0.003497442943913479, 0.004643967329382619, 0.006173960496074581, 0.008328479475960807, 0.01104771203277444, 0.014357619031198964, 0.018537486187540444, 0.02284437942631526, 0.02731439498646449, 0.032167911487225434, 0.0371910236767036, 0.04181371837917466, 0.04616169752438771, 0.05136406975454068, 0.056487730592191296, 0.06036156860361439, 0.06387329389177361, 0.06751840213948934, 0.07060362405818353, 0.07469393470751398, 0.07927291264737414, 0.08412842587038581, 0.08929060907719427, 0.09381898689685429, 0.09884959085297315, 0.10353318313260292, 0.10754256832568426, 0.11107562156643695, 0.11462961832668304, 0.11918731178071652, 0.12225260866476097, 0.12471405585959554, 0.12564448349151236, 0.12578472163260596, 0.1279348375008544, 0.12890443102176827, 0.12903926860322068, 0.13114998882126758, 0.1336971659565267, 0.13770021660900042, 0.1420001328534482, 0.1448588556751449, 0.14778827140929005, 0.149784015949724, 0.1504233424730118, 0.15132620106718814, 0.15117776291569507, 0.14772169747399203, 0.14513965811730897, 0.1425779392020619, 0.13836979852086917, 0.1327953172892106, 0.12926860954706076, 0.12674512454972442, 0.12290045205100276, 0.1183654638342986, 0.11141097006689128, 0.1039790019948737, 0.09870557797137029, 0.09462740258002188, 0.09022170740737552, 0.08703136499708622, 0.08510185101856088, 0.0843342662475137, 0.08417937900179324, 0.08370114015861757, 0.0837039104440391, 0.08306778298283372, 0.0830269883315648, 0.08420894228124409, 0.08331806380310935, 0.08245648317017443, 0.08452684692517227, 0.0866250999194714, 0.08787657004236697, 0.08922644819467765, 0.09151867592734131, 0.09110837715411145, 0.08797645275853236, 0.08418234692654473, 0.08152000091151373, 0.07969429185042892, 0.08010775896440492, 0.0831824695384769, 0.08208728249254513, 0.07734143579040814, 0.07302825144092452, 0.06964720412510024, 0.06660200487630666, 0.06493941028416385, 0.06458466708247654, 0.0665589078897689, 0.06765093898769521, 0.06806785626639567, 0.06581824826178936, 0.06322968352968339, 0.06454982486066392, 0.06420858451669281, 0.06428322097475654, 0.06412169569657233, 0.061267735176394486, 0.06045514128516717, 0.06114208447027039, 0.06250615080003744, 0.06176605373445482, 0.05931815058292283, 0.06063941335437224, 0.06150441055313468, 0.058844903785118835, 0.05695582082561253, 0.05736070493757662, 0.05797577025497415, 0.057315892595598536, 0.05633273208169081, 0.05586408015595137, 0.05595416841700372, 0.05913871987113571, 0.05859028010892939, 0.05677636438521961, 0.0572822648326117, 0.05714148692004891, 0.05675943476027412, 0.05550443225468628, 0.05726580916343009, 0.05821429528099743, 0.05716064095282886, 0.058332159076238996, 0.057169108072979404, 0.05518907824881084, 0.05519825582424094, 0.055685972462240205, 0.0537528138416211, 0.05198075386468535, 0.055748780810254035, 0.055611703708432346, 0.05251531277501485, 0.05181078462090955, 0.05132042762475772, 0.05356218968981228, 0.05531608629704088, 0.05357404284657004, 0.050415254464271524, 0.04982990113093072, 0.04929695892877396, 0.04768032152539379, 0.05018460200128213, 0.04959813908812425, 0.04622488329324016, 0.04788809577200135, 0.049495313915097906, 0.048763737757360835, 0.04578373075265562, 0.04625392115440549, 0.047968212184435394, 0.04480487107922834, 0.04583984470220321, 0.045727369951705794, 0.045697858645801115, 0.048939146165209974, 0.045770535645957525, 0.03945606580899681, 0.040812778785714536, 0.04583136620261968, 0.045606976289387674, 0.04623010284692278, 0.0449763548398343, 0.040971459264710595, 0.04282056683992751, 0.04423469767395314, 0.04060726024405095, 0.04201256224666555, 0.04474484910285757, 0.045044278287975484, 0.0411559019575878, 0.03759895893317052, 0.04189021114371698, 0.044694760618059146, 0.04536753423760257, 0.042675960689795366, 0.03724388739216042, 0.035133332716123164, 0.041832797088956604, 0.0397135668385558, 0.03454367317647515, 0.03869662787997506, 0.04025489832747296, 0.04096748277038311, 0.039576164973876525, 0.041395098492856296, 0.044321666316277424, 0.04149766692952321, 0.039206516406154794, 0.03959183611996963, 0.04362021683965829, 0.045553101193290445, 0.04275798743020648, 0.03898965544499158, 0.036501451538949584, 0.04164947124266302, 0.04204518846230424, 0.040995443790875864, 0.039215042361264205, 0.0364805802492103, 0.038565722331308505, 0.03726604502115902, 0.03776713712201024, 0.036637168345061186, 0.03409746354202667, 0.03677212656669456, 0.036238231460504505, 0.03235326139340195, 0.034962275950328546, 0.0392290790157339, 0.03609505767212853, 0.035791669315103664, 0.03616489317820255, 0.03838649374836251, 0.03703491498266279, 0.028846348924864304, 0.030695251877164556, 0.02964661149444965, 0.03243142350667006, 0.038115886612909655, 0.038563502289821326, 0.040621063812325366, 0.041961547920184555, 0.04300609409340843, 0.03943828439285334, 0.037211982882530026, 0.04325502774502028, 0.03335023617656217, 0.02347420213311059, 0.03172251263935929, 0.03118317182358953, 0.03210832240547122, 0.03568397835153294, 0.033789845171813486, 0.0333742789350679, 0.03620600805769903, 0.029020495688846504, 0.02643482963353996, 0.03019265565718972, 0.029572515136351236, 0.030886275411573422, 0.02822183755820622, 0.03173686766209077, 0.04010035096854548, 0.0400387944526791, 0.035701415249269626, 0.034012253509465615, 0.03564195934737697, 0.02855348132453926, 0.019654886765570357, 0.016923713279721836, 0.02144263822228168, 0.027055065762616303, 0.02829212323470087, 0.028342482201526412, 0.021120496139181728, 0.05863202507105306, 0.22533897542846304, 0.5462631332369434, 0.9053133227093881, 1.1248098221979268, 1.1296811741343566, 0.9456742762454364, 0.647672753347128, 0.3813516151293528, 0.22570865254211242, 0.1439432032643959, 0.12470169030994174, 0.14146699091009812, 0.14934535994700104, 0.16191320447196794, 0.16368174800412222, 0.15433095597811494, 0.13243433241610442, 0.08117357377402142, 0.036089886572425615, 0.02020621475576613, 0.01940050534301787, 0.020959361446067675, 0.02627151423656671, 0.03531678127869631, 0.034197372133827855, 0.03100904432787465, 0.03524954892673712, 0.024892599462377343, 0.019577426356421304, 0.022316176183446886, 0.023272135304952885, 0.020986200881113762, 0.025115297054066024, 0.027752270677653058, 0.021402445970871833, 0.018202872067084267, 0.01664079219394103, 0.017805777854480644, 0.014941822649454907, 0.00797088789924125, 0.00726770511432291, 0.014255377153254025, 0.013036548262431636, 0.021028072723972224, 0.03110986290629684, 0.037980715559208976, 0.030384272180123992, 0.016044416419947066, 0.021925474097404137, 0.02400119662466479, 0.013821892743169814, 0.009173191661593248, 0.02398575428570421, 0.040383353469651495, 0.02839866833736226, 0.014016442122635501, 0.02315101655304985, 0.02640652577024353, 0.03235167752889604, 0.0247876195937388, 0.021277811189143476, 0.024473603469476198, 0.018447969185296047, 0.009865270593537867, 0.01067363453646796, 0.027199684063135946, 0.033807988715647, 0.02358054273912813, 0.023463636322929252, 0.018969662350196904, 0.008857054446398662, 0.01515691303124852, 0.014983307443041933, 0.007959167163719189, 0.00045562510797786344, 0.0168435945018628, 0.03355427890665085, 0.03401634491081071, 0.024859981068456646, 0.02309370493916225, 0.02884500125576613, 0.013845374385048313, 0.009764885426562956, 0.023482133841472012, 0.018006468960647264, 0.01232728720674739, 0.019768250563363038, 0.02116157686387112, 0.01439834526504104, 0.009288887348450313, 0.013978542047900095, 0.023674891812784357, 0.025417181314882503, 0.026146053355843198, 0.013991990678970516, 0.006917969537706456, 0.013695576314807723, 0.014824037457419897, 0.014147250278163001, 0.013462506887704407, 0.011239357051845119, -0.002855690627633497, -0.005964709392623226, 0.013598066197536895, 0.019142461113378927, 0.02647409742934041, 0.025824328711068427, 0.010235610429445267, 0.016995986142098882, 0.021740302692353688, 0.009752433025483679, 0.0047751919927023585, 0.01882215915217897, 0.01301982229091171, 0.003861624535664043, 0.0004040578246666286, -0.001424830072976456, 0.008439080685126414, 0.01874071827804102, 0.007680707759138374, 0.0014338967046263146, -0.0002663834477377498, -9.611085138633845e-05, 0.01473814750038092, 0.008224632534570949, -0.0018400098284368648, 0.004455058706347926, -0.0039705348074994635, -0.0031060128582476166, 0.01501037718161178, 0.0215165464877979, 0.036884213911239576, 0.03165418115473244, 0.014041341372370841, 0.015568305500016569, 0.010151599082658919, -0.0004710605798558112, 0.0034097228118580816, 0.01922045520445779, 0.029396911522765534, 0.00965143572967557, 0.022518641733310467, 0.02831099570450088, 0.00864999324477724, 0.02208106886701466, 0.0169977963741998, -0.005515388423848872, 0.007846942120025407, 0.023091614164355644, 0.006354719251758436, -0.012313085684432177, -0.0056478060006827, 0.004855898295392094, 0.005677267542463277, 0.019542695413353326, 0.020641849563911147, 0.008389287254614717, 0.004360659485327462, 0.006219991400084702, 0.0007061812667762466, 0.013702394431599872, 0.034899324594782066, 0.027775151574899466, 0.005110515390233113, -0.004318927750992592, 0.006212646027614956, -0.01962191708448671, -0.03206293538456542, -0.009318686806432584, -0.005277920030809478, 0.01434260785863194, 0.03349021129594917, 0.015561540200397007, -0.005373880248400415, 0.010866366354159893, 0.027473108907404866, 0.01695135950033277, -0.006584446888604986, 0.008824308829463506, 0.018077574326395184, 0.00032504921939067565, 0.00418083537828043, 0.00351609415787925, -0.0015004573506283499, -0.005412496185801975, -0.0058976866919077334, -0.005459973995187645, 0.009878290307077242, -0.004105030184188164, -0.012340389291168336, 0.006706287144362394, -0.004395455756291155, -0.002511654536209699, 0.0010605840035222656, -0.021724973225722723, 0.0037198841049889742, 0.03228669634332916, -0.0013510164927091654, -0.006725288111742423, 0.005254111210271459, -0.008505224745590484, -0.0008798261174418966, -0.0026208442813380186, -0.0006380343370819771, 0.009120230143010511, -0.013712596039516734, -0.0034223211332864894, 0.0008718287244151168, -0.02279257146251628, -0.005509761184783253, 0.03347317471785593, 0.019697112966254888, 0.008652475524850378, 0.01856115919289469, 0.008463098370545905, 0.0027348309558902955, 0.019580114699976045, -0.011504551612879735, -0.038600543067015436, 0.00224730993343216, 0.02177322900506438, -0.0012240774470913135, -0.006350027426160176, 0.0049901628035816615, 0.0077273919327972345, -0.006154428214994346, -0.0009750822654362269, -0.0004289975388082388, -0.004572205999956808, 0.016476964096071824, 0.004018773760982905, 0.0001229430457828254, -0.019793867312449625, -0.010015036863813765, 0.0117172689754536, -0.008391154083263965, -0.007569261593784968, -0.006740708636034136, -0.013373478993707257, 0.0015686610142753258, 0.017785944086854997, 0.008555681855631459, -0.023502990023473315, -0.017443898736835113, 0.02041652779869328, 0.021085896794502342, 0.0016118473032616257, -0.008197393202406917, -0.0031530397454655836, 0.001630535231833647, -0.009796649670229016, -0.018593049458800453, -0.010174904702292797, -0.0019964822731150435, -0.03347049152050197, -0.04678394288221302, -0.004481906056649347, 0.03536073144927939, 0.01285285248177536, -0.003598911495164026, -0.006112420672247582, -0.01805480445161835, 0.029419262508025998, 0.03648190950099114, 0.005532042200332328, -0.03106170779709676, -0.012003084267132265, 0.008480852617430923, -0.011448433049797199, 0.0030504288466040746, 0.00987267641928917, -0.009622591972475069, -0.04592436917606674, -0.03559950577372528, -0.014665925952486078, -0.0021669809182782067, 0.011086682009418342, 0.023106074919299766, 0.005824251372592401, -0.024655236037454623, 0.01124882511543829, 0.02648184953108608, 0.017090386772097736, 0.0463962865529548, 0.012094690579580658, 0.0, 0.0, 0.0]] caption="Water Vapor Number Density"
  out "NRB HSRL Combined":dbl[][](graph)=[[2.389069914098909e-05, 4.234807003473767e-05, 9.616976172942455e-05, 0.00016545185298133647, 0.00021665359711793312, 0.0002871592867011848, 0.0005718629713476907, 0.0008446557877503887, 0.0010011846180066218, 0.0013788904960228728, 0.0017578733176398266, 0.002737670627751683, 0.004195802683406986, 0.005774414899018649, 0.0075607506165869896, 0.010458641776297288, 0.014059982183563035, 0.01768194356231083, 0.022446385561486835, 0.028447976226560853, 0.03193047820843167, 0.03686177725429714, 0.043714744081852594, 0.04719996541286336, 0.05337846895063979, 0.059238500398346466, 0.06197225840830924, 0.06746195150987228, 0.07120227174106032, 0.06774394915128157, 0.07124311042011164, 0.07879836135776848, 0.08869903199604134, 0.09850016185023722, 0.09941285261100244, 0.10043382849545202, 0.10595564411473735, 0.10961919479891787, 0.11320936110282993, 0.11300131296442976, 0.1108322307004857, 0.1155203611577188, 0.12300494649532019, 0.13032290017616024, 0.12931177806424685, 0.13261448967861383, 0.13604278783469875, 0.13518034913991822, 0.13790757715816815, 0.1413719762935417, 0.1452855018134052, 0.14289568858999066, 0.14275948174164346, 0.14215256897738646, 0.14298747289143138, 0.1570564841487504, 0.1561411390253393, 0.14772343525140966, 0.15904489703104932, 0.16217255420947319, 0.14504259040645603, 0.13846064980341116, 0.1400268389825841, 0.13319548945583637, 0.13051526516769488, 0.13305851607884137, 0.13203045000356234, 0.13212543063827337, 0.11538632592114428, 0.1020912852441899, 0.11968760252085826, 0.11976114797220885, 0.09501062685750417, 0.09115584596163681, 0.09613055564794873, 0.09558059341515904, 0.11213545480447543, 0.12166282452810119, 0.11127065532326581, 0.11410546291762559, 0.11180340358639777, 0.09172284830117101, 0.08447142773048548, 0.09451369045367154, 0.09215046803834488, 0.08959517545862306, 0.10362246581525177, 0.09495525277179265, 0.09010236023563456, 0.09014358354412418, 0.09827648806086284, 0.10920400445086158, 0.104774022788214, 0.09485256077848049, 0.09510330127341397, 0.10392523072410413, 0.08617380444804958, 0.09221693440906308, 0.09700491525881808, 0.07927398021878318, 0.08438412582762603, 0.09733634832278523, 0.09664167960245826, 0.09053686489007284, 0.07654049140194276, 0.0697055521599543, 0.07328215873240229, 0.07523271168284572, 0.07487712949382662, 0.06791544747141644, 0.05762848709852866, 0.05434785835771752, 0.06915533134746057, 0.07934423161414915, 0.07553237487905384, 0.06359975308271842, 0.05256835871913167, 0.05004286361065397, 0.06344548479590699, 0.05813486741957846, 0.06199144847669024, 0.08134283360606177, 0.07225214383220009, 0.08706029172653437, 0.07308214519231478, 0.050023178064017605, 0.058761788123501496, 0.06614456026405371, 0.06718210616175037, 0.09901815361950833, 0.11153341355701413, 0.09779824435883967, 0.09318831654115946, 0.056576983202160515, 0.0708848267820362, 0.107458412224096, 0.09795369962934505, 0.06656879185308588, 0.06373181788839805, 0.07526772086310035, 0.06264240382279757, 0.05658454422082574, 0.06644577193021682, 0.0714622383631685, 0.06314142330885152, 0.046173984460568786, 0.05957559816827863, 0.06685966723230245, 0.0535562788367162, 0.05538534459855245, 0.037042527403163154, 0.047772097013616094, 0.08413195879501573, 0.06421689216691213, 0.06150496912284322, 0.07667952011627188, 0.06795681980887129, 0.055305231508792026, 0.054762830791313555, 0.06427662184442168, 0.057425368768602714, 0.06201724663615279, 0.06670959241345467, 0.05958538321825311, 0.06969709820476198, 0.07190118914593134, 0.07551631411886543, 0.08059227161755332, 0.06889873788817852, 0.06260218384830353, 0.04894456541898726, 0.05097518840645286, 0.08104011492930988, 0.09092364956474619, 0.07387780007091725, 0.08997559971133251, 0.09562849318484312, 0.07955236275463502, 0.08044872033269983, 0.07815969705461938, 0.04838486049340366, 0.03587501119162384, 0.04451386913943718, 0.02666728742839209, 0.06739693743429104, 0.10049056842759749, 0.08435698908342547, 0.07482083591955951, 0.07034290729263144, 0.06753460866011426, 0.03951081642560164, 0.038110774789404896, 0.05134552667980351, 0.042614602996169725, 0.05803133584185652, 0.13239261906633298, 0.11463880967601464, 0.034739792806738515, 0.07993321595134194, 0.08861597742155428, 0.027844680480024375, 0.03414879913502209, 0.0791211943679834, 0.04712108933703368, 0.028963953792555244, 0.06685234302041178, 0.0442981930596574, 0.03620756900739132, 0.09246969595411608, 0.11289777891019298, 0.06356139711785483, 0.06637798510471397, 0.08487472743215302, 0.047344863342436705, -0.002275571941453722, 0.0022967952305399265, 0.057954578610980544, 0.05147095857597909, 0.047221925174553314, 0.07624784150692644, 0.05530183401360201, 0.05337712992295583, 0.05875552095867187, 0.04199221020975562, 0.07975303670016841, 0.01257198655988423, -0.03551289584964051, 0.0025590835747682523, 0.03097941224241941, 0.10156789007416638, 0.06830085595301677, -0.023846663828101168, 0.03474375228940063, 0.1293940084137015, 0.06253032868698781, -0.0027418118951045207, 0.011060458899355823, 0.039039481228447345, 0.0703014182683391, 0.05954808560844515, 0.025733322934599824, 0.017298146476975595, 0.005813770457596669, 0.05275656322166066, 0.0561449462641778, 0.02383301104206938, 0.06006885663297935, 0.03633336073983645, 0.024417848463535983, -0.006153512693423888, 0.00620287138815302, 0.1219275480391278, 0.11344307946471067, 0.060345645200827906, 0.0352122232447199, 0.051620609313182415, 0.03901831008561162, -0.0327678539745381, 0.04953514492192135, 0.09983872804108812, 0.04694951805598229, 0.023654772367087965, 0.013620340073876037, 0.0480350201909799, 0.0795145736902439, 0.059215577678600695, 0.04211382924333702, 0.09546908349221944, 0.07124592330343095, 0.0, -0.03253795403908254, -0.014568329720385695, 0.025682747650875526, 0.0923994551550888, 0.27924348851906333, 0.48758334558472144, 0.623376635761768, 0.6545291842812454, 0.5135737312328953, 0.26632883038771427, 0.17881772323062467, 0.18792331662450137, 0.161656809987804, 0.16280127940636438, 0.08797089071487882, 0.2335645354743974, 0.5393919601317375, 0.6575301015266752, 0.6456510703290498, 0.36851085268464956, 0.10005180619560601, 0.041974500911045425, 0.008452410371288532, -0.025530348839767868, -0.042840311461663644, -0.012939491275703707, 0.034739342835116295, 0.10055125955127688, 0.06161585801328333, 0.026583450292463007, 0.10704637041518286, 0.16613098366005732, 0.12203331875608675, 0.08644217166097885, 0.09159149286634603, 0.0414862937329624, 0.027838484517937176, -0.004669980673965729, -0.0094006967276929, 0.03311612995275849, 0.05713773062106076, 0.02396051882851771, 0.0434060693614058, 0.06795312285855508, 0.10746582494532289, 0.14256164215989112, 0.06925779304366647, 0.049782199171145604, 0.0, 0.040328183136821745, 0.07608936759886849, 0.04083386074568579, 0.005135938563250173, -0.07234764413654182, 0.010399490331481449, 0.10463829611248364, 0.14739525416372812, 0.09003686908494796, 0.01598560034520197, 0.010721936067203123, -0.021573864247609986, -0.016278333710431477, 0.038212430117912984, 0.060409608247412115, 0.11049562254152842, 0.16117848855635183, 0.07827262982193234, 0.07873784502264562, 0.04525932748307317, 0.04552673799430267, 0.1259383581805703, -0.04606296737785324, -0.0752902072335588, 0.052429856627620126, 0.005859397554762834, 0.05893483006974472, 0.14226494647213336, 0.16693464691752596, 0.2398543280185269, 0.22313764197137215, 0.2608081090461083, 0.12199465017051046, -0.018402769681041847, 0.05552241002862058, 0.13649161591065068, 0.2620517870116711, 0.15058280662514364, 0.06309368472934916, 0.04441248641458343, 0.05742047575496526, 0.12189696863130219, 0.0903165344626201, 0.0713553163357708, -0.03913495649814758, -0.11149086896545617, 0.019783326834026616, 0.03978331484935055, -0.046666362745567284, 0.03351504154554775, 0.20218819332581306, 0.20328257938318653, 0.06131230800057957, -0.130129208924708, -0.19968208481859195, -0.05538118384725738, 0.05567809784327452, 0.06996849596530746, -0.056270827184579736, -0.10606582005818453, -0.02843407779551923, 0.05002258626506114, 0.1795953179984439, 0.10832069995157677, 0.043554324959171394, -0.014593670703724094, -0.029339084869952792, 0.08110264456960328, 0.04446643267587279, 0.10429159909204648, 0.044926030994262484, 0.09031413441836199, 0.21181666653400968, 0.07603349234389725, 0.11463212768294123, 0.19202707910081424, 0.10035875147846982, 0.0, -0.12476458874843716, -0.015674325988892422, 0.2441818207678381, 0.1820722387179054, -0.031821750055866266, -0.14390857904348825, 0.0, 0.1372722472826683, 0.016229210776616106, 0.07339231781122098, 0.114728271365233, 0.11529135406002224, 0.30619949073785846, 0.24116382746445852, 0.06685026482789716, 0.10076328381947781, -0.025312466292577968, 0.06782735684315551, 0.2555871437851856, 0.19689155862474642, 0.025804159557977744, -0.02592757062470117, 0.06947159673179058, 0.061077377616616725, 0.026300382035226458, -0.07927429607792649, -0.09734920820102544, -0.11559208902380433, 0.017867530484221798, 0.11668650391744413, 0.1623246149757573, 0.0543604975030576, 0.10012672169086827, 0.41153481454513363, 0.30318953704170526, 0.27690330298366234, 0.25963752109589705, 0.0, -0.159084017465621, -0.15981459752647173, -0.0661083832596926, 0.07589929474913497, 0.10483793033722065, -0.019147860834076345, 0.028852383346791303, -0.009660978213917823, -0.058227484484201925, 0.1072341485280378, 0.10771664127561252, 0.19672996074315216, 0.3754699749728414, 0.1984943461795025, 0.009968729299218432, 0.060078893032636325, 0.1709816747985872, 0.0505107054187345, -0.11161239207437343, 0.020383001049703642, 0.13307441426529884, 0.21591246755621804, 0.27882012739003564, 0.16594667954575473, 0.11458525857105313, 0.14647111062338214, 0.14710724933487596, 0.24272637447353354, 0.12718566652321517, -0.10644235961847996, -0.03207049131969861, -0.07515226536520868, -0.09703834160014178, -0.03248474525765912, -0.08699522497322067, 0.0, 0.05483666406447742, 0.23129572300506637, 0.3097024766386086, 0.09996523798004658, 0.10038658730445224, 0.1904186383293902, 0.11248008381215173, 0.22590533420851697, 0.02268442672069421, -0.10250423584150782, -0.08005756777603062, -0.18374666135030782, -0.13838194548634553, -0.03473899556390845, 0.2093000740174577, 0.11675561088585724, -0.08206310764473339, -0.04708576950514094, -0.106376040151737, -2.108178643759601e-17, 0.3694226766396622, 0.3350285622164237, 0.2402754265319174, 0.14474801175985993, 0.1937789279295637, 0.21888178454748683, 0.061044383953276084, -0.19612198784721088, -0.18460227243298313, 0.13592161855667728, 0.01240572670775428, -0.03736540983581215, -0.0500187721974142, -0.18831277810888608, -0.23947388492871036, -0.25307478519902266, 0.06352057991209109, 0.05101665958275928, -0.1152370180902407, -0.07712654703351644, 0.10324014883026365, 0.16842230555451881, -0.026011735032829077, 0.039169823371515346, 0.22282919964940795, 0.4210787047220012, 0.17172139087662572, -0.05304038524292835, -0.07986725815948484, -0.1870724439116279, -0.16096435538001747, -0.08079146174965136, 0.13517065305581732, 0.040705750086808996, 0.20430801205136342, 0.5195656323702181, 0.24703852662569611, 0.28930548306862663, 0.08296990207947622, -0.22208244872666155, 0.2507957126654005, 0.4615312735159519, 0.19653171225865276, 0.028180772734942273, 0.056572586301150654, -0.17034809455447023, -0.5414283415376182, -0.4433390632172001, -0.04306468745429144, 0.21612670876839735, 0.39047365564446906, 0.3338525103310035, -0.04370504576979832, -0.05848775593638573, -0.10272912774882986, -0.17675160306256385, -0.04435012997693257, -0.029674798068970446, 0.10424172019468725, 0.23913678906389613, 0.0450002897939267, 0.06021805400760394, -0.01510891158427713, -0.04549039901614582, 0.2891532546159578, 0.030546096812797994, 0.0, 0.0, 0.0]] caption="Water Vapor Number Density"
  out "CH 1 (WV off) counts display":dbl[][](graph)=[[24.12, 11.120000000000001, 19.12, 19.12, 18.12, 15.120000000000001, 34.12, 23.12, 27.12, 33.12, 37.12, 43.12, 47.12, 52.12, 67.12, 66.12, 89.12, 111.12, 128.12, 135.12, 149.12, 157.12, 169.12, 192.12, 171.12, 183.12, 205.12, 206.12, 192.12, 185.12, 198.12, 194.12, 178.12, 151.12, 170.12, 175.12, 199.12, 153.12, 198.12, 186.12, 168.12, 188.12, 186.12, 166.12, 171.12, 146.12, 159.12, 157.12, 128.12, 144.12, 109.12, 113.12, 137.12, 148.12, 112.12, 112.12, 122.12, 103.12, 131.12, 99.12, 82.12, 94.12, 104.12, 76.12, 77.12, 70.12, 84.12, 60.12, 54.12, 55.12, 38.12, 58.12, 43.12, 44.12, 44.12, 41.12, 40.12, 35.12, 38.12, 31.12, 26.12, 29.12, 39.12, 33.12, 21.12, 26.12, 40.12, 32.12, 30.12, 36.12, 29.12, 35.12, 23.12, 21.12, 18.12, 16.12, 19.12, 18.12, 19.12, 15.120000000000001, 7.12, 15.120000000000001, 17.12, 13.120000000000001, 30.12, 12.120000000000001, 12.120000000000001, 11.120000000000001, 16.12, 14.120000000000001, 11.120000000000001, 10.120000000000001, 7.12, 12.120000000000001, 14.120000000000001, 21.12, 15.120000000000001, 14.120000000000001, 17.12, 12.120000000000001, 14.120000000000001, 6.12, 5.12, 10.120000000000001, 11.120000000000001, 15.120000000000001, 9.120000000000001, 11.120000000000001, 16.12, 9.120000000000001, 8.120000000000001, 14.120000000000001, 7.12, 11.120000000000001, 8.120000000000001, 8.120000000000001, 10.120000000000001, 9.120000000000001, 15.120000000000001, 4.12, 5.12, 12.120000000000001, 6.12, 7.12, 7.12, 4.12, 8.120000000000001, 9.120000000000001, 14.120000000000001, 7.12, 1.12, 11.120000000000001, 4.12, 5.12, 9.120000000000001, 10.120000000000001, 9.120000000000001, 1.12, 10.120000000000001, 9.120000000000001, 11.120000000000001, 12.120000000000001, 1.12, 1.12, -2.88, 1.12, 3.12, 5.12, 0.1200000000000001, 2.12, 1.12, 4.12, 6.12, 5.12, 7.12, 5.12, 4.12, 5.12, 4.12, 3.12, 3.12, 1.12, -1.88, 0.1200000000000001, 8.120000000000001, 4.12, 2.12, -2.88, 2.12, 9.120000000000001, 7.12, 7.12, 0.1200000000000001, 0.1200000000000001, 5.12, 7.12, 1.12, 3.12, 3.12, 6.12, -0.8799999999999999, 5.12, -2.88, 0.1200000000000001, 6.12, 3.12, 1.12, 0.1200000000000001, 3.12, 7.12, 6.12, 3.12, 2.12, 1.12, -3.88, 3.12, 0.1200000000000001, -2.88, -2.88, 0.1200000000000001, 4.12, 2.12, 3.12, 1.12, 6.12, 4.12, 3.12, 1.12, 1.12, 1.12, 0.1200000000000001, 7.12, -0.8799999999999999, 1.12, 9.120000000000001, 1.12, 3.12, 3.12, 2.12, 1.12, 0.1200000000000001, 5.12, 1.12, 2.12, 0.1200000000000001, 6.12, 7.12, 1.12, 2.12, 1.12, -0.8799999999999999, 2.12, 2.12, 4.12, 2.12, 2.12, 3.12, 0.1200000000000001, 2.12, 6.12, 4.12, 0.1200000000000001, -1.88, 0.1200000000000001, 7.12, 3.12, -1.88, 5.12, -0.8799999999999999, -0.8799999999999999, 1.12, -4.88, 9.120000000000001, -0.8799999999999999, 13.120000000000001, 27.12, 39.12, 45.12, 36.12, 17.12, 13.120000000000001, 3.12, 0.1200000000000001, 0.1200000000000001, 16.12, 10.120000000000001, 18.12, 19.12, 17.12, 18.12, 11.120000000000001, 4.12, 0.1200000000000001, -1.88, -1.88, -0.8799999999999999, 1.12, 0.1200000000000001, -2.88, 2.12, 0.1200000000000001, 3.12, 4.12, 1.12, 2.12, 2.12, -1.88, -1.88, -0.8799999999999999, 2.12, 2.12, 0.1200000000000001, -1.88, 3.12, 3.12, 5.12, 1.12, -0.8799999999999999, 3.12, -1.88, 5.12, 6.12, 1.12, 4.12, 0.1200000000000001, 0.1200000000000001, 0.1200000000000001, 1.12, 2.12, -3.88, 5.12, 2.12, 0.1200000000000001, 2.12, 2.12, 0.1200000000000001, -1.88, 3.12, 0.1200000000000001, 3.12, 1.12, 0.1200000000000001, -1.88, 1.12, -3.88, -0.8799999999999999, -0.8799999999999999, -2.88, 2.12, 1.12, 4.12, 5.12, -0.8799999999999999, 1.12, 2.12, -2.88, 1.12, -2.88, 1.12, 2.12, 3.12, -0.8799999999999999, 1.12, 0.1200000000000001, -1.88, 6.12, 0.1200000000000001, 0.1200000000000001, 7.12, 4.12, 0.1200000000000001, -2.88, -1.88, 3.12, 3.12, 3.12, -1.88, 1.12, 2.12, 5.12, 2.12, 4.12, -2.88, -0.8799999999999999, 2.12, 2.12, 2.12, -1.88, -0.8799999999999999, 2.12, -0.8799999999999999, -2.88, 2.12, 5.12, -1.88, -1.88, 3.12, 0.1200000000000001, 2.12, 1.12, 2.12, -0.8799999999999999, 3.12, -1.88, -2.88, 2.12, 2.12, -0.8799999999999999, -4.88, -0.8799999999999999, 3.12, -0.8799999999999999, 3.12, 1.12, 5.12, 1.12, -1.88, 0.1200000000000001, 3.12, -1.88, 2.12, 3.12, 3.12, 0.1200000000000001, -0.8799999999999999, 1.12, 1.12, -2.88, -0.8799999999999999, 1.12, 4.12, -0.8799999999999999, 2.12, 2.12, -1.88, -0.8799999999999999, 7.12, -1.88, 2.12, 3.12, -3.88, -0.8799999999999999, 0.1200000000000001, -0.8799999999999999, -0.8799999999999999, -0.8799999999999999, 7.12, -0.8799999999999999, -0.8799999999999999, 2.12, 6.12, 3.12, 1.12, 4.12, 7.12, 4.12, 1.12, 3.12, 1.12, 2.12, 1.12, -0.8799999999999999, -0.8799999999999999, -0.8799999999999999, 1.12, -2.88, 1.12, -0.8799999999999999, 1.12, 4.12, 0.1200000000000001, 2.12, 1.12, -2.88, 3.12, -0.8799999999999999, 0.1200000000000001, 2.12, 0.1200000000000001, -2.88, -0.8799999999999999, 1.12, 0.1200000000000001, 0.1200000000000001, 3.12, 1.12, -3.88, -1.88, -4.88, 3.12, 2.12, 0.1200000000000001, -1.88, 1.12, -2.88, -0.8799999999999999, 4.12, 4.12, 1.12, 4.12, 0.1200000000000001, 3.12, 2.12, 1.12, 3.12, -1.88, 0.1200000000000001, 2.12, 0.1200000000000001, 1.12, -0.8799999999999999, 2.12, -0.8799999999999999, 0.1200000000000001, 5.12, -0.8799999999999999, -2.88, 1.12, 1.12, 4.12, 2.12, -3.88, 0.1200000000000001, 1.12, 4.12, 6.12, 1.12, 0.1200000000000001, -0.8799999999999999, 6.12, 3.12, -2.88, -1.88, -0.8799999999999999, -0.8799999999999999, -1.88, -3.88, 3.12, 1.12, -0.8799999999999999, -1.88, 1.12, 8.120000000000001, 3.12, -1.88, -1.88, 2.12, -1.88, 3.12, -3.88, -3.88, -2.88, 1.12, 1.12, 2.12, 0.1200000000000001, 4.12, -0.8799999999999999, -3.88, 0.0]] caption="Water Vapor Number Density"
  out "CH 3 (HSRL comb) counts display":dbl[][](graph)=[[80.24, 29.240000000000002, 27.240000000000002, 29.240000000000002, 24.240000000000002, 33.24, 30.240000000000002, 33.24, 23.240000000000002, 30.240000000000002, 37.24, 43.24, 59.24, 67.24, 86.24, 83.24, 113.24, 127.24, 154.24, 156.24, 180.24, 153.24, 211.24, 213.24, 233.24, 242.24, 214.24, 198.24, 210.24, 192.24, 177.24, 212.24, 223.24, 220.24, 190.24, 207.24, 186.24, 190.24, 198.24, 180.24, 174.24, 182.24, 164.24, 179.24, 176.24, 153.24, 154.24, 143.24, 117.24, 136.24, 134.24, 137.24, 109.24, 118.24, 101.24, 125.24, 117.24, 108.24, 124.24, 107.24, 111.24, 68.24, 84.24, 84.24, 102.24, 65.24, 54.24, 74.24, 64.24, 60.24, 46.24, 67.24, 41.24, 48.24, 43.24, 51.24, 52.24, 46.24, 43.24, 46.24, 45.24, 43.24, 41.24, 37.24, 49.24, 26.240000000000002, 31.240000000000002, 30.240000000000002, 20.240000000000002, 20.240000000000002, 30.240000000000002, 27.240000000000002, 17.240000000000002, 32.24, 18.240000000000002, 23.240000000000002, 29.240000000000002, 14.24, 30.240000000000002, 22.240000000000002, 20.240000000000002, 19.240000000000002, 27.240000000000002, 23.240000000000002, 17.240000000000002, 14.24, 20.240000000000002, 18.240000000000002, 11.24, 17.240000000000002, 9.24, 9.24, 12.24, 16.240000000000002, 10.24, 9.24, 13.24, 11.24, 13.24, 16.240000000000002, 5.24, 14.24, 14.24, 9.24, 11.24, 11.24, 9.24, 14.24, 14.24, 8.24, 23.240000000000002, 11.24, 10.24, 6.24, 7.24, 6.24, 20.240000000000002, 15.24, 4.24, 12.24, 9.24, 6.24, 10.24, 9.24, 7.24, 11.24, 9.24, 5.24, 8.24, 5.24, 5.24, -2.76, 6.24, 17.240000000000002, 5.24, 4.24, 2.24, -2.76, -3.76, 13.24, 5.24, 7.24, 6.24, -1.7599999999999998, 4.24, 13.24, 2.24, 8.24, 9.24, 9.24, 4.24, 13.24, 0.2400000000000002, 8.24, 6.24, 2.24, 9.24, 11.24, 3.24, 5.24, 6.24, 0.2400000000000002, 11.24, -1.7599999999999998, 3.24, 5.24, 3.24, 4.24, -6.76, 6.24, 4.24, 1.2400000000000002, -0.7599999999999998, 8.24, -2.76, 1.2400000000000002, 0.2400000000000002, 2.24, 12.24, 8.24, 1.2400000000000002, 0.2400000000000002, 3.24, 6.24, -2.76, 9.24, 1.2400000000000002, 5.24, 2.24, 5.24, 3.24, -1.7599999999999998, -1.7599999999999998, 2.24, -1.7599999999999998, 0.2400000000000002, 8.24, 6.24, 3.24, 3.24, 6.24, -1.7599999999999998, 0.2400000000000002, -0.7599999999999998, 5.24, 10.24, 2.24, -0.7599999999999998, 3.24, 2.24, 9.24, 3.24, -5.76, 3.24, 7.24, -4.76, 8.24, -3.76, -2.76, 10.24, -7.76, -7.76, 7.24, -0.7599999999999998, 2.24, -0.7599999999999998, 0.2400000000000002, 5.24, -3.76, 10.24, -5.76, 6.24, 5.24, 12.24, 2.24, 4.24, -1.7599999999999998, -0.7599999999999998, -2.76, 8.24, 3.24, 6.24, 6.24, 7.24, -1.7599999999999998, -1.7599999999999998, 6.24, 2.24, 9.24, -3.76, -0.7599999999999998, -2.76, 4.24, 6.24, 1.2400000000000002, 14.24, 24.240000000000002, 20.240000000000002, 19.240000000000002, 15.24, 0.2400000000000002, 4.24, 3.24, 1.2400000000000002, 10.24, -8.76, 10.24, 15.24, 21.240000000000002, 20.240000000000002, 7.24, 4.24, -4.76, 0.2400000000000002, -5.76, 11.24, -2.76, 0.2400000000000002, 0.2400000000000002, 6.24, 5.24, 8.24, 4.24, -1.7599999999999998, 1.2400000000000002, 2.24, 2.24, 6.24, 6.24, -1.7599999999999998, -1.7599999999999998, 0.2400000000000002, -6.76, 5.24, 5.24, 4.24, -3.76, 1.2400000000000002, 4.24, -1.7599999999999998, 7.24, -1.7599999999999998, 0.2400000000000002, 2.24, -4.76, 1.2400000000000002, 3.24, 2.24, -2.76, -0.7599999999999998, -4.76, 0.2400000000000002, -0.7599999999999998, -0.7599999999999998, -2.76, 4.24, 1.2400000000000002, 2.24, -1.7599999999999998, -2.76, 6.24, 7.24, -8.76, 2.24, 1.2400000000000002, 1.2400000000000002, 4.24, 2.24, 12.24, 1.2400000000000002, 1.2400000000000002, -6.76, 0.2400000000000002, 4.24, 0.2400000000000002, 3.24, 4.24, -0.7599999999999998, 2.24, 8.24, 1.2400000000000002, -1.7599999999999998, 6.24, 2.24, -5.76, 0.2400000000000002, 7.24, 0.2400000000000002, 4.24, 4.24, 5.24, -4.76, -4.76, -4.76, -0.7599999999999998, -4.76, 6.24, 5.24, -4.76, 5.24, -0.7599999999999998, -5.76, 0.2400000000000002, 0.2400000000000002, 9.24, 0.2400000000000002, -1.7599999999999998, 8.24, -5.76, 0.2400000000000002, -3.76, 8.24, 3.24, 3.24, -2.76, 2.24, -1.7599999999999998, -2.76, -7.76, 1.2400000000000002, -0.7599999999999998, 7.24, 1.2400000000000002, 2.24, 1.2400000000000002, 2.24, -0.7599999999999998, 2.24, -3.76, 3.24, 7.24, 1.2400000000000002, -5.76, 4.24, -2.76, 4.24, -1.7599999999999998, 6.24, -5.76, -3.76, 0.2400000000000002, 3.24, 2.24, -1.7599999999999998, 4.24, -1.7599999999999998, 3.24, 9.24, 2.24, -3.76, 2.24, 2.24, 11.24, 4.24, 2.24, 1.2400000000000002, -0.7599999999999998, -2.76, -0.7599999999999998, 0.2400000000000002, -5.76, -2.76, -5.76, -4.76, 1.2400000000000002, 7.24, 0.2400000000000002, 10.24, -0.7599999999999998, -5.76, 3.24, -2.76, 3.24, -4.76, 5.24, -2.76, 4.24, -0.7599999999999998, 8.24, -1.7599999999999998, 3.24, 3.24, 3.24, 4.24, 0.2400000000000002, 4.24, -1.7599999999999998, -3.76, 5.24, 1.2400000000000002, 0.2400000000000002, 4.24, 1.2400000000000002, 10.24, 0.2400000000000002, -1.7599999999999998, 0.2400000000000002, 5.24, -0.7599999999999998, 5.24, -3.76, -0.7599999999999998, -5.76, -2.76, 4.24, 1.2400000000000002, 8.24, 0.2400000000000002, -6.76, 1.2400000000000002, -5.76, -5.76, 7.24, 2.24, 7.24, -1.7599999999999998, 3.24, 3.24, 5.24, -4.76, 0.2400000000000002, -0.7599999999999998, -7.76, 8.24, 1.2400000000000002, 3.24, -3.76, 2.24, 8.24, -2.76, 5.24, 5.24, -0.7599999999999998, 5.24, -0.7599999999999998, 4.24, 2.24, 4.24, 2.24, 0.2400000000000002, 2.24, 1.2400000000000002, 0.2400000000000002, -8.76, 3.24, 5.24, 7.24, 3.24, 0.2400000000000002, 7.24, -3.76, 1.2400000000000002, 3.24, 2.24, 2.24, -0.7599999999999998, -1.7599999999999998, 1.2400000000000002, -6.76, -2.76, 0.2400000000000002, 5.24, 5.24, 3.24, -2.76, 5.24, -0.7599999999999998, -0.7599999999999998, 1.2400000000000002, 4.24, -1.7599999999999998, 3.24, -0.7599999999999998, 0.2400000000000002, -5.76, 2.24, -4.76, 0.2400000000000002, -4.76, 0.0]] caption="Water Vapor Number Density"
  out "CH3 (HSRL combined) smooth":dbl[](array[numeric])=[60.625, 26.875, 27.125, 26.25, 22.0, 20.25, 29.625, 33.5, 31.375, 35.0, 36.875, 48.25, 63.0, 74.75, 85.25, 103.625, 123.375, 138.375, 157.625, 180.25, 183.5, 193.0, 209.375, 207.625, 216.375, 222.0, 215.375, 218.0, 214.5, 190.75, 187.875, 195.0, 206.375, 215.875, 205.625, 196.375, 196.125, 192.375, 188.625, 179.0, 167.125, 166.0, 168.625, 170.625, 161.875, 158.875, 156.125, 148.75, 145.625, 143.375, 141.625, 134.0, 128.875, 123.625, 119.875, 127.0, 121.875, 111.375, 115.875, 114.25, 98.875, 91.375, 89.5, 82.5, 78.375, 77.5, 74.625, 72.5, 61.5, 52.875, 60.25, 58.625, 45.25, 42.25, 43.375, 42.0, 48.0, 50.75, 45.25, 45.25, 43.25, 34.625, 31.125, 34.0, 32.375, 30.75, 34.75, 31.125, 28.875, 28.25, 30.125, 32.75, 30.75, 27.25, 26.75, 28.625, 23.25, 24.375, 25.125, 20.125, 21.0, 23.75, 23.125, 21.25, 17.625, 15.75, 16.25, 16.375, 16.0, 14.25, 11.875, 11.0, 13.75, 15.5, 14.5, 12.0, 9.75, 9.125, 11.375, 10.25, 10.75, 13.875, 12.125, 14.375, 11.875, 8.0, 9.25, 10.25, 10.25, 14.875, 16.5, 14.25, 13.375, 8.0, 9.875, 14.75, 13.25, 8.875, 8.375, 9.75, 8.0, 7.125, 8.25, 8.75, 7.625, 5.5, 7.0, 7.75, 6.125, 6.25, 4.125, 5.25, 9.125, 6.875, 6.5, 8.0, 7.0, 5.625, 5.5, 6.375, 5.625, 6.0, 6.375, 5.625, 6.5, 6.625, 6.875, 7.25, 6.125, 5.5, 4.25, 4.375, 6.875, 7.625, 6.125, 7.375, 7.75, 6.375, 6.375, 6.125, 3.75, 2.75, 3.375, 2.0, 5.0, 7.375, 6.125, 5.375, 5.0, 4.75, 2.75, 2.625, 3.5, 2.875, 3.875, 8.75, 7.5, 2.25, 5.125, 5.625, 1.75, 2.125, 4.875, 2.875, 1.75, 4.0, 2.625, 2.125, 5.375, 6.5, 3.625, 3.75, 4.75, 2.625, -0.125, 0.125, 3.125, 2.75, 2.5, 4.0, 2.875, 2.75, 3.0, 2.125, 4.0, 0.625, -1.75, 0.125, 1.5, 4.875, 3.25, -1.125, 1.625, 6.0, 2.875, -0.125, 0.5, 1.75, 3.125, 2.625, 1.125, 0.75, 0.25, 2.25, 2.375, 1.0, 2.5, 1.5, 1.0, -0.25, 0.25, 4.875, 4.5, 2.375, 1.375, 2.0, 1.5, -1.25, 1.875, 3.75, 1.75, 0.875, 0.5, 1.75, 2.875, 2.125, 1.5, 3.375, 2.5, 0.0, -1.125, -0.5, 0.875, 3.125, 9.375, 16.25, 20.625, 21.5, 16.75, 8.625, 5.75, 6.0, 5.125, 5.125, 2.75, 7.250000000000001, 16.625, 20.125, 19.625, 11.125, 3.0, 1.25, 0.25, -0.75, -1.2500000000000002, -0.3750000000000002, 1.0, 2.875, 1.75, 0.75, 3.0, 4.625, 3.375, 2.375, 2.5, 1.125, 0.75, -0.125, -0.25, 0.875, 1.5, 0.625, 1.125, 1.75, 2.75, 3.625, 1.75, 1.25, 0.0, 1.0, 1.875, 1.0, 0.125, -1.75, 0.25, 2.5, 3.5, 2.125, 0.375, 0.25, -0.5, -0.375, 0.875, 1.375, 2.5, 3.625, 1.75, 1.75, 1.0, 1.0, 2.75, -1.0, -1.625, 1.125, 0.125, 1.25, 3.0, 3.5, 5.0, 4.625, 5.375, 2.5, -0.375, 1.125, 2.75, 5.25, 3.0, 1.25, 0.875, 1.125, 2.375, 1.75, 1.375, -0.75, -2.125, 0.375, 0.75, -0.875, 0.625, 3.75, 3.75, 1.125, -2.375, -3.625, -1.0, 1.0, 1.25, -1.0, -1.875, -0.5, 0.875, 3.125, 1.875, 0.75, -0.25, -0.5, 1.375, 0.75, 1.75, 0.75, 1.5, 3.5, 1.25, 1.8749999999999998, 3.125, 1.625, 0.0, -2.0, -0.25, 3.875, 2.875, -0.5, -2.25, 0.0, 2.125, 0.25, 1.125, 1.75, 1.75, 4.625, 3.625, 1.0, 1.5, -0.375, 1.0, 3.75, 2.875, 0.375, -0.375, 1.0, 0.875, 0.375, -1.125, -1.375, -1.625, 0.25, 1.625, 2.25, 0.75, 1.375, 5.625, 4.125, 3.75, 3.5, 0.0, -2.125, -2.125, -0.875, 1.0, 1.375, -0.25, 0.375, -0.125, -0.75, 1.375, 1.375, 2.5, 4.75, 2.5, 0.125, 0.75, 2.125, 0.625, -1.375, 0.25, 1.625, 2.625, 3.375, 2.0, 1.375, 1.75, 1.75, 2.875, 1.5, -1.25, -0.375, -0.875, -1.125, -0.375, -1.0, 0.0, 0.625, 2.625, 3.5, 1.125, 1.125, 2.125, 1.25, 2.5, 0.25, -1.125, -0.875, -2.0, -1.5, -0.375, 2.25, 1.25, -0.875, -0.5, -1.125, -2.220446049250313e-16, 3.875, 3.5, 2.5, 1.5, 2.0, 2.25, 0.625, -2.0, -1.875, 1.375, 0.125, -0.375, -0.5, -1.875, -2.375, -2.5, 0.625, 0.5, -1.125, -0.75, 1.0, 1.625, -0.25, 0.375, 2.125, 4.0, 1.625, -0.5, -0.75, -1.75, -1.5, -0.75, 1.25, 0.375, 1.875, 4.75, 2.25, 2.625, 0.75, -2.0, 2.25, 4.125, 1.75, 0.25, 0.5, -1.5, -4.75, -3.875, -0.375, 1.875, 3.375, 2.875, -0.375, -0.5, -0.875, -1.5, -0.375, -0.25, 0.875, 2.0, 0.375, 0.5, -0.125, -0.375, 2.375, 0.25]
  out "CH3 Bin Readings":dbl[](array[numeric])=[94.0, 43.0, 41.0, 43.0, 38.0, 47.0, 44.0, 47.0, 37.0, 44.0, 51.0, 57.0, 73.0, 81.0, 100.0, 97.0, 127.0, 141.0, 168.0, 170.0, 194.0, 167.0, 225.0, 227.0, 247.0, 256.0, 228.0, 212.0, 224.0, 206.0, 191.0, 226.0, 237.0, 234.0, 204.0, 221.0, 200.0, 204.0, 212.0, 194.0, 188.0, 196.0, 178.0, 193.0, 190.0, 167.0, 168.0, 157.0, 131.0, 150.0, 148.0, 151.0, 123.0, 132.0, 115.0, 139.0, 131.0, 122.0, 138.0, 121.0, 125.0, 82.0, 98.0, 98.0, 116.0, 79.0, 68.0, 88.0, 78.0, 74.0, 60.0, 81.0, 55.0, 62.0, 57.0, 65.0, 66.0, 60.0, 57.0, 60.0, 59.0, 57.0, 55.0, 51.0, 63.0, 40.0, 45.0, 44.0, 34.0, 34.0, 44.0, 41.0, 31.0, 46.0, 32.0, 37.0, 43.0, 28.0, 44.0, 36.0, 34.0, 33.0, 41.0, 37.0, 31.0, 28.0, 34.0, 32.0, 25.0, 31.0, 23.0, 23.0, 26.0, 30.0, 24.0, 23.0, 27.0, 25.0, 27.0, 30.0, 19.0, 28.0, 28.0, 23.0, 25.0, 25.0, 23.0, 28.0, 28.0, 22.0, 37.0, 25.0, 24.0, 20.0, 21.0, 20.0, 34.0, 29.0, 18.0, 26.0, 23.0, 20.0, 24.0, 23.0, 21.0, 25.0, 23.0, 19.0, 22.0, 19.0, 19.0, 11.0, 20.0, 31.0, 19.0, 18.0, 16.0, 11.0, 10.0, 27.0, 19.0, 21.0, 20.0, 12.0, 18.0, 27.0, 16.0, 22.0, 23.0, 23.0, 18.0, 27.0, 14.0, 22.0, 20.0, 16.0, 23.0, 25.0, 17.0, 19.0, 20.0, 14.0, 25.0, 12.0, 17.0, 19.0, 17.0, 18.0, 7.0, 20.0, 18.0, 15.0, 13.0, 22.0, 11.0, 15.0, 14.0, 16.0, 26.0, 22.0, 15.0, 14.0, 17.0, 20.0, 11.0, 23.0, 15.0, 19.0, 16.0, 19.0, 17.0, 12.0, 12.0, 16.0, 12.0, 14.0, 22.0, 20.0, 17.0, 17.0, 20.0, 12.0, 14.0, 13.0, 19.0, 24.0, 16.0, 13.0, 17.0, 16.0, 23.0, 17.0, 8.0, 17.0, 21.0, 9.0, 22.0, 10.0, 11.0, 24.0, 6.0, 6.0, 21.0, 13.0, 16.0, 13.0, 14.0, 19.0, 10.0, 24.0, 8.0, 20.0, 19.0, 26.0, 16.0, 18.0, 12.0, 13.0, 11.0, 22.0, 17.0, 20.0, 20.0, 21.0, 12.0, 12.0, 20.0, 16.0, 23.0, 10.0, 13.0, 11.0, 18.0, 20.0, 15.0, 28.0, 38.0, 34.0, 33.0, 29.0, 14.0, 18.0, 17.0, 15.0, 24.0, 5.0, 24.0, 29.0, 35.0, 34.0, 21.0, 18.0, 9.0, 14.0, 8.0, 25.0, 11.0, 14.0, 14.0, 20.0, 19.0, 22.0, 18.0, 12.0, 15.0, 16.0, 16.0, 20.0, 20.0, 12.0, 12.0, 14.0, 7.0, 19.0, 19.0, 18.0, 10.0, 15.0, 18.0, 12.0, 21.0, 12.0, 14.0, 16.0, 9.0, 15.0, 17.0, 16.0, 11.0, 13.0, 9.0, 14.0, 13.0, 13.0, 11.0, 18.0, 15.0, 16.0, 12.0, 11.0, 20.0, 21.0, 5.0, 16.0, 15.0, 15.0, 18.0, 16.0, 26.0, 15.0, 15.0, 7.0, 14.0, 18.0, 14.0, 17.0, 18.0, 13.0, 16.0, 22.0, 15.0, 12.0, 20.0, 16.0, 8.0, 14.0, 21.0, 14.0, 18.0, 18.0, 19.0, 9.0, 9.0, 9.0, 13.0, 9.0, 20.0, 19.0, 9.0, 19.0, 13.0, 8.0, 14.0, 14.0, 23.0, 14.0, 12.0, 22.0, 8.0, 14.0, 10.0, 22.0, 17.0, 17.0, 11.0, 16.0, 12.0, 11.0, 6.0, 15.0, 13.0, 21.0, 15.0, 16.0, 15.0, 16.0, 13.0, 16.0, 10.0, 17.0, 21.0, 15.0, 8.0, 18.0, 11.0, 18.0, 12.0, 20.0, 8.0, 10.0, 14.0, 17.0, 16.0, 12.0, 18.0, 12.0, 17.0, 23.0, 16.0, 10.0, 16.0, 16.0, 25.0, 18.0, 16.0, 15.0, 13.0, 11.0, 13.0, 14.0, 8.0, 11.0, 8.0, 9.0, 15.0, 21.0, 14.0, 24.0, 13.0, 8.0, 17.0, 11.0, 17.0, 9.0, 19.0, 11.0, 18.0, 13.0, 22.0, 12.0, 17.0, 17.0, 17.0, 18.0, 14.0, 18.0, 12.0, 10.0, 19.0, 15.0, 14.0, 18.0, 15.0, 24.0, 14.0, 12.0, 14.0, 19.0, 13.0, 19.0, 10.0, 13.0, 8.0, 11.0, 18.0, 15.0, 22.0, 14.0, 7.0, 15.0, 8.0, 8.0, 21.0, 16.0, 21.0, 12.0, 17.0, 17.0, 19.0, 9.0, 14.0, 13.0, 6.0, 22.0, 15.0, 17.0, 10.0, 16.0, 22.0, 11.0, 19.0, 19.0, 13.0, 19.0, 13.0, 18.0, 16.0, 18.0, 16.0, 14.0, 16.0, 15.0, 14.0, 5.0, 17.0, 19.0, 21.0, 17.0, 14.0, 21.0, 10.0, 15.0, 17.0, 16.0, 16.0, 13.0, 12.0, 15.0, 7.0, 11.0, 14.0, 19.0, 19.0, 17.0, 11.0, 19.0, 13.0, 13.0, 15.0, 18.0, 12.0, 17.0, 13.0, 14.0, 8.0, 16.0, 9.0, 14.0, 9.0]
  out "CH2 (molecular) smoothed":dbl[](array[numeric])=[6.448, 6.648000000000001, 5.248000000000001, 3.9480000000000004, 4.948, 3.5480000000000005, 2.9480000000000004, 4.748, 6.748, 8.948, 9.948, 15.648, 19.448, 23.247999999999998, 24.048000000000002, 25.148000000000003, 31.548000000000002, 37.048, 48.548, 50.348, 47.748000000000005, 59.748000000000005, 65.648, 67.74799999999999, 63.548, 61.147999999999996, 70.74799999999999, 72.44799999999998, 69.04799999999999, 74.04799999999999, 78.94799999999998, 69.648, 59.748000000000005, 60.248, 56.647999999999996, 55.448, 58.348, 52.048, 49.748000000000005, 49.448, 45.448, 47.448, 49.147999999999996, 49.348, 46.348, 39.848, 41.44800000000001, 41.548, 40.548, 41.248000000000005, 42.548, 38.548, 30.148000000000003, 33.147999999999996, 33.748000000000005, 33.548, 30.648, 23.648, 21.548000000000002, 25.548000000000002, 27.247999999999998, 20.548, 21.348, 23.148, 22.247999999999998, 22.348, 21.247999999999998, 23.148000000000003, 21.848, 16.248, 17.548000000000002, 19.548000000000002, 16.548000000000002, 15.947999999999999, 19.247999999999998, 18.948, 15.248000000000003, 15.448, 12.648, 12.648, 16.048000000000002, 13.948000000000002, 14.048000000000002, 12.248000000000001, 9.548000000000002, 14.847999999999999, 13.248, 8.848, 13.148, 11.048000000000002, 7.848000000000001, 14.047999999999998, 13.148, 8.048, 8.148, 8.048, 9.448, 11.148, 10.848, 5.048, 6.248, 9.048, 6.248, 5.248, 1.3480000000000003, 1.6480000000000006, 2.8480000000000008, 6.048000000000001, 8.748000000000001, 7.648, 10.548, 12.648, 12.948, 8.948, 4.948, 4.148000000000001, 3.4480000000000004, 6.348000000000001, 4.848000000000001, 3.748, 6.148, 8.248000000000001, 8.948, 6.648000000000001, 7.648000000000001, 5.448, 3.4480000000000004, 4.648000000000001, 6.548000000000001, 2.048000000000001, 0.04800000000000049, 3.8480000000000003, 3.748, 5.448, 4.548, 3.048, -0.15199999999999947, -0.9519999999999995, -1.6519999999999997, -2.752, 2.148, 3.9480000000000004, 3.3480000000000008, 3.1480000000000006, 3.4480000000000004, 2.5480000000000005, 0.14800000000000035, 0.048000000000000376, 0.6480000000000005, 0.2480000000000004, -0.5519999999999996, 2.4480000000000004, 5.048, 0.7480000000000004, 0.4480000000000004, 5.748, 9.148, 11.048000000000002, 8.348, 6.648000000000001, 7.348000000000001, 2.0480000000000005, -0.0519999999999996, 3.7480000000000007, 2.7480000000000007, 2.5480000000000005, -0.5519999999999996, -3.0519999999999996, 1.4480000000000004, 3.748, 1.7480000000000002, -1.3519999999999996, 1.4480000000000002, 2.9480000000000004, 0.8480000000000003, -0.8519999999999996, 1.2480000000000002, 3.148, 2.8480000000000003, 2.248, 3.1480000000000006, 4.648, -0.2519999999999998, -1.8519999999999996, 1.8480000000000003, 0.7480000000000003, 2.2480000000000007, 1.9480000000000006, -1.1519999999999995, 3.1480000000000006, 3.5480000000000005, 1.3480000000000003, 2.048, 0.14800000000000035, -0.6519999999999996, 3.5480000000000005, -0.4519999999999995, -2.452, 1.1480000000000004, 1.8480000000000003, 3.3480000000000003, -0.5519999999999996, -0.9519999999999996, -0.25199999999999967, -1.3519999999999996, -0.8519999999999996, -0.4519999999999996, -0.8519999999999995, 3.6480000000000006, 5.148000000000001, 2.3480000000000008, 0.34800000000000053, -0.5519999999999996, 1.8480000000000003, 2.6480000000000006, 3.6480000000000006, 2.1480000000000006, -2.5519999999999996, -3.5519999999999996, 0.6480000000000004, 1.0480000000000005, -0.7519999999999996, 1.6480000000000001, 1.5480000000000003, 1.0480000000000005, 1.3480000000000005, 0.24800000000000041, 0.24800000000000041, -0.0519999999999996, 0.04800000000000039, -2.5519999999999996, -2.352, 0.14800000000000038, -2.1519999999999997, -2.5519999999999996, 1.3480000000000003, 2.0480000000000005, -2.6519999999999997, -1.4519999999999997, 3.748, 3.5480000000000005, 1.6480000000000006, 0.048000000000000376, 1.6480000000000004, 3.8480000000000003, 2.5480000000000005, 0.9480000000000004, 0.7480000000000004, 1.0480000000000005, 1.8480000000000003, 1.0480000000000005, -3.3519999999999994, -4.252, 0.6480000000000004, 2.3480000000000003, 0.9480000000000004, 0.6480000000000004, 2.0480000000000005, 1.3480000000000003, -0.0519999999999996, -0.5519999999999996, 1.8480000000000003, 2.8480000000000003, 0.3480000000000004, -1.0519999999999996, -2.1519999999999997, 0.048000000000000376, 2.3480000000000003, 2.3480000000000003, 1.5480000000000005, 2.248, 2.0480000000000005, -1.9519999999999997, -4.052, -0.0519999999999996, 0.6480000000000004, -1.0519999999999996, -1.5519999999999996, 1.0480000000000003, 1.0480000000000003, -0.7519999999999996, 0.8480000000000004, 0.8480000000000004, 2.5480000000000005, 3.4480000000000004, 4.048, 1.6480000000000006, 1.4480000000000004, 2.6480000000000006, 0.7480000000000004, -1.2519999999999998, -2.252, 1.4480000000000004, 1.7480000000000002, -1.6519999999999997, -0.7519999999999996, -1.4519999999999995, -2.252, 0.5480000000000004, 0.34800000000000036, -1.0519999999999996, -0.5519999999999996, -0.9519999999999995, -2.1519999999999992, -0.25199999999999956, 1.8480000000000003, -0.1519999999999997, -1.4519999999999995, -3.9519999999999995, 0.24800000000000066, 4.648000000000001, -0.7519999999999997, -1.9519999999999995, 0.24800000000000044, 2.5480000000000005, 4.448, 4.548, 3.048, 2.5480000000000005, 3.548, 5.248, 4.748, 4.148000000000001, 3.3480000000000003, 1.6480000000000004, 1.4480000000000004, 2.8480000000000008, 0.24800000000000066, -3.0519999999999996, 0.9480000000000004, 4.648000000000001, 2.3480000000000003, 1.0480000000000005, 0.8480000000000003, -0.15199999999999964, 1.3480000000000003, 0.6480000000000004, -0.9519999999999996, -0.7519999999999997, -2.6519999999999992, 0.34800000000000075, 2.2480000000000007, 1.2480000000000002, 2.3480000000000003, 3.3480000000000008, 5.248000000000001, 4.348000000000001, 1.2480000000000002, 0.14800000000000035, 2.048, 2.048, 1.8480000000000003, 1.4480000000000004, 0.04800000000000043, -0.15199999999999964, -0.15199999999999964, 0.2480000000000004, 0.9480000000000004, 0.0480000000000004, -2.5519999999999996, -1.9519999999999997, 0.6480000000000004, -0.8519999999999996, -3.252, -3.252, -1.3519999999999996, -0.5519999999999996, 0.1480000000000004, -1.3519999999999996, -1.5519999999999996, -3.252, -6.952, -2.452, -1.1519999999999995, -3.4519999999999995, -0.4519999999999996, 2.5480000000000005, 0.8480000000000004, -1.2519999999999996, -0.3519999999999996, 0.4480000000000004, -1.9519999999999997, -2.1519999999999997, 0.7480000000000004, -0.25199999999999956, -1.6519999999999997, -1.5519999999999996, 0.24800000000000033, 4.148000000000001, 2.0480000000000005, -1.1519999999999995, -0.7519999999999996, -4.151999999999999, -6.252, -3.452, 1.5480000000000003, 1.7480000000000002, -0.5519999999999996, -0.2519999999999996, -0.7519999999999997, -0.4519999999999996, -0.8519999999999996, -2.1519999999999997, -0.9519999999999996, 1.0480000000000003, -0.25199999999999956, -1.1519999999999995, -3.452, -2.452, 1.5480000000000005, 0.44800000000000045, -1.8519999999999996, -3.9519999999999995, 0.24800000000000066, 4.248000000000001, 2.2480000000000007, 0.3480000000000004, 0.04800000000000039, 3.5480000000000005, 2.6480000000000006, 1.2480000000000002, -0.35199999999999987, -0.9519999999999997, 0.24800000000000044, -0.5519999999999995, -1.1519999999999997, 0.14800000000000035, 4.748, 3.748, 3.748, 2.0480000000000005, 2.6480000000000006, 4.148000000000001, 0.4480000000000004, -2.6519999999999997, -1.5519999999999996, 2.1480000000000006, 0.04800000000000049, -1.7519999999999996, 0.34800000000000036, 4.648000000000001, 4.548, 3.5480000000000005, 4.648000000000001, -0.6519999999999997, -2.0519999999999996, -1.3519999999999996, -1.2519999999999996, -0.8519999999999996, -0.1519999999999997, 1.4480000000000004, 0.8480000000000004, 0.5480000000000004, -2.6519999999999992, -4.751999999999999, 0.14800000000000058, 1.8480000000000005, -0.35199999999999965, 0.04800000000000039, 1.6480000000000004, 0.6480000000000004, -0.5519999999999996, -0.0519999999999996, 1.5480000000000003, 2.748, -1.5519999999999996, -3.752, -3.1519999999999997, -2.0519999999999996, 0.9480000000000004, -0.6519999999999995, -0.15199999999999947, 1.5480000000000005, 0.6480000000000005, 0.4480000000000004, -2.452, -0.35199999999999965, 3.4480000000000004, 1.2480000000000002, 0.8480000000000004, 2.1480000000000006, -2.252, -2.6519999999999997, -1.9519999999999995, -2.9519999999999995, 5.048, 4.848, -1.7519999999999996, -0.9519999999999996, -0.9519999999999996, -3.1519999999999997, -5.452, -6.552, -3.0519999999999996, 0.4480000000000004, -0.0519999999999996, 1.8480000000000003, -1.0519999999999998, -1.5519999999999998, 2.748, 3.0480000000000005, 1.7480000000000004, 1.6480000000000004, 0.3480000000000003, 1.9480000000000004, 2.4480000000000004, -3.0519999999999996, -1.5519999999999996, 3.0480000000000005, 1.5480000000000005, 2.1480000000000006, 2.5480000000000005, -0.15199999999999958, 0.2480000000000004, 1.4480000000000004, 0.048000000000000265, -1.8519999999999996, -1.2519999999999996, -2.1519999999999997, 0.048000000000000265, 2.3480000000000003, -2.252, -1.7519999999999996, 2.248, 2.4480000000000004, -0.9519999999999995, -4.052, -2.4519999999999995, 0.7480000000000004, 0.6480000000000004, 1.8480000000000005, 7.248, 5.248, -0.8519999999999996, -0.6519999999999997, 3.9480000000000004, 3.6480000000000006, -1.2519999999999993, -3.5519999999999996, -0.7519999999999996, 3.3480000000000003, 0.9480000000000004, -0.0519999999999996, -1.7519999999999998, -3.952, 3.748, 7.048, 1.5480000000000005, 0.7480000000000004, 1.7480000000000004, -2.7519999999999993, -2.7519999999999993, -0.2519999999999996, -1.8519999999999996, -3.3519999999999994, -0.35199999999999965, -0.4519999999999995]
  out "CH 2 Bin Readings":dbl[](array[numeric])=[40.0, 41.0, 56.0, 48.0, 41.0, 41.0, 45.0, 49.0, 55.0, 46.0, 55.0, 57.0, 60.0, 67.0, 48.0, 77.0, 54.0, 71.0, 80.0, 93.0, 88.0, 98.0, 114.0, 105.0, 111.0, 90.0, 116.0, 111.0, 114.0, 115.0, 106.0, 129.0, 100.0, 98.0, 95.0, 93.0, 91.0, 115.0, 92.0, 93.0, 88.0, 87.0, 96.0, 73.0, 104.0, 90.0, 88.0, 74.0, 87.0, 88.0, 88.0, 83.0, 74.0, 76.0, 85.0, 77.0, 83.0, 56.0, 78.0, 58.0, 72.0, 63.0, 57.0, 68.0, 80.0, 86.0, 60.0, 66.0, 61.0, 66.0, 59.0, 68.0, 58.0, 38.0, 61.0, 63.0, 66.0, 52.0, 49.0, 54.0, 50.0, 53.0, 53.0, 60.0, 57.0, 48.0, 69.0, 55.0, 52.0, 59.0, 55.0, 54.0, 55.0, 52.0, 53.0, 56.0, 52.0, 50.0, 58.0, 49.0, 45.0, 51.0, 45.0, 48.0, 44.0, 50.0, 42.0, 54.0, 60.0, 51.0, 48.0, 47.0, 54.0, 57.0, 40.0, 44.0, 52.0, 46.0, 56.0, 39.0, 38.0, 41.0, 47.0, 63.0, 35.0, 46.0, 45.0, 51.0, 45.0, 63.0, 27.0, 44.0, 37.0, 49.0, 47.0, 44.0, 48.0, 41.0, 39.0, 35.0, 41.0, 38.0, 41.0, 47.0, 46.0, 50.0, 49.0, 47.0, 37.0, 41.0, 35.0, 35.0, 52.0, 48.0, 47.0, 51.0, 58.0, 50.0, 42.0, 47.0, 53.0, 58.0, 31.0, 47.0, 52.0, 36.0, 38.0, 43.0, 41.0, 47.0, 49.0, 44.0, 39.0, 72.0, 52.0, 60.0, 51.0, 40.0, 46.0, 53.0, 47.0, 48.0, 40.0, 44.0, 39.0, 49.0, 32.0, 34.0, 33.0, 33.0, 48.0, 40.0, 44.0, 41.0, 43.0, 42.0, 49.0, 34.0, 48.0, 42.0, 40.0, 56.0, 36.0, 32.0, 46.0, 31.0, 31.0, 37.0, 34.0, 44.0, 41.0, 36.0, 42.0, 39.0, 43.0, 48.0, 46.0, 42.0, 40.0, 36.0, 35.0, 48.0, 46.0, 37.0, 40.0, 40.0, 41.0, 48.0, 28.0, 39.0, 48.0, 48.0, 42.0, 48.0, 37.0, 41.0, 45.0, 37.0, 40.0, 47.0, 47.0, 36.0, 32.0, 42.0, 38.0, 38.0, 46.0, 39.0, 49.0, 45.0, 33.0, 44.0, 37.0, 32.0, 57.0, 44.0, 41.0, 35.0, 48.0, 40.0, 54.0, 34.0, 32.0, 41.0, 45.0, 41.0, 34.0, 43.0, 44.0, 49.0, 37.0, 53.0, 46.0, 43.0, 42.0, 53.0, 43.0, 47.0, 48.0, 54.0, 42.0, 32.0, 35.0, 48.0, 42.0, 33.0, 40.0, 42.0, 46.0, 59.0, 39.0, 42.0, 40.0, 42.0, 42.0, 44.0, 42.0, 31.0, 42.0, 38.0, 37.0, 62.0, 43.0, 35.0, 48.0, 42.0, 43.0, 48.0, 44.0, 38.0, 55.0, 42.0, 34.0, 50.0, 42.0, 42.0, 40.0, 48.0, 56.0, 37.0, 50.0, 47.0, 39.0, 45.0, 37.0, 38.0, 41.0, 42.0, 34.0, 29.0, 53.0, 51.0, 47.0, 39.0, 38.0, 42.0, 44.0, 39.0, 53.0, 35.0, 40.0, 50.0, 39.0, 36.0, 39.0, 42.0, 55.0, 44.0, 35.0, 42.0, 45.0, 37.0, 39.0, 42.0, 45.0, 36.0, 31.0, 36.0, 36.0, 55.0, 42.0, 35.0, 52.0, 31.0, 35.0, 35.0, 35.0, 40.0, 35.0, 43.0, 46.0, 42.0, 34.0, 45.0, 36.0, 48.0, 48.0, 37.0, 45.0, 41.0, 41.0, 45.0, 42.0, 46.0, 52.0, 37.0, 35.0, 46.0, 47.0, 45.0, 53.0, 41.0, 34.0, 34.0, 43.0, 37.0, 41.0, 31.0, 48.0, 45.0, 48.0, 49.0, 41.0, 46.0, 36.0, 47.0, 42.0, 49.0, 31.0, 30.0, 39.0, 41.0, 45.0, 38.0, 43.0, 38.0, 34.0, 41.0, 44.0, 48.0, 43.0, 47.0, 38.0, 42.0, 40.0, 42.0, 42.0, 49.0, 52.0, 50.0, 48.0, 34.0, 50.0, 48.0, 40.0, 34.0, 39.0, 44.0, 39.0, 43.0, 44.0, 42.0, 52.0, 54.0, 54.0, 26.0, 49.0, 42.0, 49.0, 36.0, 36.0, 39.0, 47.0, 38.0, 45.0, 39.0, 56.0, 47.0, 47.0, 37.0, 47.0, 36.0, 34.0, 31.0, 38.0, 52.0, 45.0, 31.0, 36.0, 49.0, 44.0, 36.0, 47.0, 39.0, 38.0, 36.0, 45.0, 40.0, 37.0, 32.0, 35.0, 40.0, 31.0, 51.0, 43.0, 37.0, 53.0, 45.0, 34.0, 42.0, 38.0, 21.0, 29.0, 36.0, 53.0, 35.0, 45.0, 45.0, 34.0, 44.0, 42.0, 36.0, 45.0, 38.0, 40.0, 54.0, 41.0, 48.0, 46.0, 46.0, 45.0, 41.0, 34.0, 47.0, 37.0, 40.0, 43.0, 51.0, 40.0, 42.0, 44.0, 38.0, 35.0, 30.0, 38.0, 38.0, 41.0, 32.0, 51.0, 51.0, 43.0, 43.0, 37.0, 39.0, 38.0, 41.0, 56.0, 37.0, 46.0, 38.0, 47.0, 40.0, 46.0, 36.0, 31.0, 41.0, 44.0, 41.0, 39.0, 45.0, 40.0, 40.0, 40.0, 33.0, 37.0, 42.0, 47.0, 34.0, 44.0]
  in  "stop":bool
  in  "Reset Average":bool=TRUE
  in  "Save Data?":bool=TRUE
  in  "Collect Data?":bool=TRUE
  in  "ILX Address":i32=6 min=0 step=1
  in  "Lambda On DBR Current":dbl=171.13999999999868
  in  "Lambda Off DBR Current":dbl=172.9499999999997
  in  "Tab Control":T2(tab)=enum."OD"
  out "Water Vapor Number Density":cluster{"Y":dbl[], "Y":dbl[]}[](graph)
  out "Absolute Humidity":cluster{"Y":dbl[], "Y":dbl[]}[](graph)
  out "NRB plot":cluster{"Y":dbl[], "Y":dbl[]}[](graph)
  in  "background length":i32=25
  out "Correction":cluster{"Y":dbl[], "Y":dbl[]}[](graph)
  in  "dead time":dbl=3.7e-08
  out "Optical Depth":cluster{"Y":dbl[], "Y":dbl[]}[](graph) caption="XY Graph"
  out "aerosol profile":cluster{"Y":dbl[], "Y":dbl[]}[](graph)
  out "CH1 RingBuffer long":dbl[][](array[numeric])
  in  "Weather":T3(tab)=enum."Pulse Energy (Micro Joule)"
  out "Temperature (C)":dbl(graph)=4.895909645909647
  out "Pressure (mb)":dbl(graph)=838.5714285714286
  out "Relative Humdity (%)":dbl(graph)=48.92551892551892
  out "Pulse Energy (Micro Joule)":T4(graph)={"WV Online Pulse Energy"=1618.0, "WV_averaged_energy"=1581.0, "HSRL"=268435849.0, "WV_averaged_energy"=0.0}
  out "?":cluster{"mean":dbl, "mean":dbl}(graph)={"mean"=1926.4963248162408, "mean"=3852.9926496324815}
  out "Index":i32=1
  out "CH1  Bin Readings":dbl[](array[numeric])=[31.0, 18.0, 26.0, 26.0, 25.0, 22.0, 41.0, 30.0, 34.0, 40.0, 44.0, 50.0, 54.0, 59.0, 74.0, 73.0, 96.0, 118.0, 135.0, 142.0, 156.0, 164.0, 176.0, 199.0, 178.0, 190.0, 212.0, 213.0, 199.0, 192.0, 205.0, 201.0, 185.0, 158.0, 177.0, 182.0, 206.0, 160.0, 205.0, 193.0, 175.0, 195.0, 193.0, 173.0, 178.0, 153.0, 166.0, 164.0, 135.0, 151.0, 116.0, 120.0, 144.0, 155.0, 119.0, 119.0, 129.0, 110.0, 138.0, 106.0, 89.0, 101.0, 111.0, 83.0, 84.0, 77.0, 91.0, 67.0, 61.0, 62.0, 45.0, 65.0, 50.0, 51.0, 51.0, 48.0, 47.0, 42.0, 45.0, 38.0, 33.0, 36.0, 46.0, 40.0, 28.0, 33.0, 47.0, 39.0, 37.0, 43.0, 36.0, 42.0, 30.0, 28.0, 25.0, 23.0, 26.0, 25.0, 26.0, 22.0, 14.0, 22.0, 24.0, 20.0, 37.0, 19.0, 19.0, 18.0, 23.0, 21.0, 18.0, 17.0, 14.0, 19.0, 21.0, 28.0, 22.0, 21.0, 24.0, 19.0, 21.0, 13.0, 12.0, 17.0, 18.0, 22.0, 16.0, 18.0, 23.0, 16.0, 15.0, 21.0, 14.0, 18.0, 15.0, 15.0, 17.0, 16.0, 22.0, 11.0, 12.0, 19.0, 13.0, 14.0, 14.0, 11.0, 15.0, 16.0, 21.0, 14.0, 8.0, 18.0, 11.0, 12.0, 16.0, 17.0, 16.0, 8.0, 17.0, 16.0, 18.0, 19.0, 8.0, 8.0, 4.0, 8.0, 10.0, 12.0, 7.0, 9.0, 8.0, 11.0, 13.0, 12.0, 14.0, 12.0, 11.0, 12.0, 11.0, 10.0, 10.0, 8.0, 5.0, 7.0, 15.0, 11.0, 9.0, 4.0, 9.0, 16.0, 14.0, 14.0, 7.0, 7.0, 12.0, 14.0, 8.0, 10.0, 10.0, 13.0, 6.0, 12.0, 4.0, 7.0, 13.0, 10.0, 8.0, 7.0, 10.0, 14.0, 13.0, 10.0, 9.0, 8.0, 3.0, 10.0, 7.0, 4.0, 4.0, 7.0, 11.0, 9.0, 10.0, 8.0, 13.0, 11.0, 10.0, 8.0, 8.0, 8.0, 7.0, 14.0, 6.0, 8.0, 16.0, 8.0, 10.0, 10.0, 9.0, 8.0, 7.0, 12.0, 8.0, 9.0, 7.0, 13.0, 14.0, 8.0, 9.0, 8.0, 6.0, 9.0, 9.0, 11.0, 9.0, 9.0, 10.0, 7.0, 9.0, 13.0, 11.0, 7.0, 5.0, 7.0, 14.0, 10.0, 5.0, 12.0, 6.0, 6.0, 8.0, 2.0, 16.0, 6.0, 20.0, 34.0, 46.0, 52.0, 43.0, 24.0, 20.0, 10.0, 7.0, 7.0, 23.0, 17.0, 25.0, 26.0, 24.0, 25.0, 18.0, 11.0, 7.0, 5.0, 5.0, 6.0, 8.0, 7.0, 4.0, 9.0, 7.0, 10.0, 11.0, 8.0, 9.0, 9.0, 5.0, 5.0, 6.0, 9.0, 9.0, 7.0, 5.0, 10.0, 10.0, 12.0, 8.0, 6.0, 10.0, 5.0, 12.0, 13.0, 8.0, 11.0, 7.0, 7.0, 7.0, 8.0, 9.0, 3.0, 12.0, 9.0, 7.0, 9.0, 9.0, 7.0, 5.0, 10.0, 7.0, 10.0, 8.0, 7.0, 5.0, 8.0, 3.0, 6.0, 6.0, 4.0, 9.0, 8.0, 11.0, 12.0, 6.0, 8.0, 9.0, 4.0, 8.0, 4.0, 8.0, 9.0, 10.0, 6.0, 8.0, 7.0, 5.0, 13.0, 7.0, 7.0, 14.0, 11.0, 7.0, 4.0, 5.0, 10.0, 10.0, 10.0, 5.0, 8.0, 9.0, 12.0, 9.0, 11.0, 4.0, 6.0, 9.0, 9.0, 9.0, 5.0, 6.0, 9.0, 6.0, 4.0, 9.0, 12.0, 5.0, 5.0, 10.0, 7.0, 9.0, 8.0, 9.0, 6.0, 10.0, 5.0, 4.0, 9.0, 9.0, 6.0, 2.0, 6.0, 10.0, 6.0, 10.0, 8.0, 12.0, 8.0, 5.0, 7.0, 10.0, 5.0, 9.0, 10.0, 10.0, 7.0, 6.0, 8.0, 8.0, 4.0, 6.0, 8.0, 11.0, 6.0, 9.0, 9.0, 5.0, 6.0, 14.0, 5.0, 9.0, 10.0, 3.0, 6.0, 7.0, 6.0, 6.0, 6.0, 14.0, 6.0, 6.0, 9.0, 13.0, 10.0, 8.0, 11.0, 14.0, 11.0, 8.0, 10.0, 8.0, 9.0, 8.0, 6.0, 6.0, 6.0, 8.0, 4.0, 8.0, 6.0, 8.0, 11.0, 7.0, 9.0, 8.0, 4.0, 10.0, 6.0, 7.0, 9.0, 7.0, 4.0, 6.0, 8.0, 7.0, 7.0, 10.0, 8.0, 3.0, 5.0, 2.0, 10.0, 9.0, 7.0, 5.0, 8.0, 4.0, 6.0, 11.0, 11.0, 8.0, 11.0, 7.0, 10.0, 9.0, 8.0, 10.0, 5.0, 7.0, 9.0, 7.0, 8.0, 6.0, 9.0, 6.0, 7.0, 12.0, 6.0, 4.0, 8.0, 8.0, 11.0, 9.0, 3.0, 7.0, 8.0, 11.0, 13.0, 8.0, 7.0, 6.0, 13.0, 10.0, 4.0, 5.0, 6.0, 6.0, 5.0, 3.0, 10.0, 8.0, 6.0, 5.0, 8.0, 15.0, 10.0, 5.0, 5.0, 9.0, 5.0, 10.0, 3.0, 3.0, 4.0, 8.0, 8.0, 9.0, 7.0, 11.0, 6.0, 3.0]
  out "CH1 (WV off) smooth":dbl[](array[numeric])=[20.227486033519547, 19.484469273743013, 19.61016759776536, 20.607374301675975, 22.020782122905025, 23.830837988826804, 26.30290502793295, 29.45932960893854, 34.235865921787706, 38.38949720670391, 41.730279329608926, 46.51519553072625, 52.523575418994426, 60.129720670391066, 69.62972067039104, 82.54312849162011, 96.97608938547484, 112.39787709497206, 130.2218994413408, 144.8084916201118, 157.02636871508383, 168.47888268156427, 178.19955307262572, 183.9900558659218, 187.19117318435752, 192.5626815642458, 196.36715083798885, 195.11575418994414, 192.47888268156427, 190.12972067039107, 186.20513966480445, 184.87553072625698, 184.49843575418996, 184.4509497206704, 184.7414525139665, 183.47888268156424, 183.0096089385475, 181.72748603351957, 179.21351955307264, 175.96770949720673, 172.85318435754192, 171.27217877094972, 167.607374301676, 163.3056983240224, 157.30290502793298, 150.71631284916205, 146.8448044692738, 141.8643575418995, 136.2833519553073, 133.0319553072626, 130.35318435754195, 129.14368715083805, 128.19955307262575, 125.98446927374306, 123.90346368715086, 121.13530726256985, 117.42581005586595, 114.09620111731846, 110.15765363128492, 104.08782122905028, 98.94815642458101, 94.09620111731843, 88.44815642458101, 82.2582122905028, 77.63251396648045, 73.8308379888268, 69.47329608938546, 64.95932960893853, 59.38670391061453, 53.8559776536313, 49.69675977653632, 46.330837988826815, 42.973296089385464, 40.342011173184346, 38.40346368715083, 37.06268156424581, 36.04033519553073, 34.92301675977654, 34.045921787709496, 32.948156424581, 32.12413407821229, 31.79173184357542, 30.70234636871508, 29.666033519553064, 29.699553072625683, 29.733072625698313, 29.473296089385464, 29.249832402234627, 29.330837988826804, 28.554301675977648, 26.970502793296085, 25.249832402234627, 23.9286033519553, 22.897877094972063, 22.534748603351954, 22.914636871508375, 22.149273743016757, 20.445363128491614, 18.917430167597757, 17.68279329608938, 16.57664804469274, 15.84759776536313, 15.456536312849163, 15.62413407821229, 15.579441340782124, 15.381117318435756, 14.596201117318437, 13.763798882681563, 13.794525139664803, 13.473296089385475, 13.247039106145252, 12.978882681564244, 12.182793296089384, 11.811284916201117, 11.738659217877094, 11.794525139664804, 11.456536312849162, 10.816871508379887, 10.872737430167597, 10.844804469273743, 10.20513966480447, 9.716312849162012, 9.626927374301676, 9.573854748603353, 9.314078212290504, 9.009608938547487, 8.794525139664804, 8.671620111731842, 9.023575418994412, 8.802905027932962, 8.400670391061453, 8.347597765363128, 8.202346368715084, 8.026368715083798, 7.733072625698323, 7.8615642458100545, 7.875530726256983, 7.621340782122903, 7.666033519553071, 7.406256983240224, 7.048715083798884, 6.950949720670392, 6.914636871508382, 6.58223463687151, 6.277765363128493, 6.640893854748605, 6.534748603351956, 6.087821229050279, 5.925810055865922, 5.79173184357542, 5.96491620111732, 6.079441340782124, 5.811284916201119, 5.397877094972068, 5.266592178770951, 5.143687150837989, 4.911843575418995, 5.104581005586594, 4.981675977653634, 4.5850279329608945, 4.691173184357542, 4.788938547486033, 4.660446927374303, 4.322458100558661, 4.314078212290504, 4.420223463687153, 4.0794413407821235, 4.124134078212291, 4.065474860335195, 4.015195530726258, 4.249832402234639, 3.928603351955308, 3.347597765363127, 3.4230167597765355, 3.8001117318435753, 3.738659217877095, 3.7470391061452513, 3.6045810055865912, 3.24703910614525, 3.3559776536312844, 3.4286033519553065, 3.112960893854748, 3.1855865921787703, 3.3559776536312835, 3.342011173184356, 3.020782122905027, 2.730279329608938, 3.009608938547485, 3.1772067039106133, 3.191173184357541, 2.9705027932960886, 2.565474860335195, 2.3950837988826814, 2.8224581005586584, 2.652067039106144, 2.283351955307262, 2.531955307262569, 2.607374301675977, 2.6269273743016757, 2.5124022346368715, 2.601787709497206, 2.758212290502793, 2.5570949720670386, 2.392290502793296, 2.392290502793297, 2.6101675977653636, 2.699553072625698, 2.509608938547486, 2.2665921787709493, 2.101787709497206, 2.375530726256983, 2.375530726256983, 2.2945251396648043, 2.174413407821229, 2.004022346368715, 2.0989944134078207, 2.0096089385474856, 2.0179888268156425, 1.9397765363128485, 1.7889385474860329, 1.9118435754189935, 1.867150837988826, 1.6520670391061447, 1.7693854748603348, 1.967709497206703, 1.794525139664804, 1.7637988826815643, 1.7665921787709493, 1.85877094972067, 1.7777653631284915, 1.3727374301675979, 1.448156424581006, 1.3867039106145254, 1.5040223463687146, 1.7526256983240218, 1.7582122905027928, 1.8364245810055864, 1.881117318435754, 1.911843575418994, 1.7386592178770948, 1.6269273743016754, 1.8755307262569825, 1.4341899441340782, 1.0012290502793297, 1.3420111731843578, 1.3084916201117323, 1.3364245810055868, 1.473296089385475, 1.3839106145251399, 1.3559776536312853, 1.459329608938548, 1.1604469273743017, 1.048715083798883, 1.1883798882681569, 1.154860335195531, 1.1967597765363132, 1.085027932960894, 1.2107262569832404, 1.5179888268156425, 1.504022346368715, 1.3308379888268158, 1.2582122905027933, 1.3084916201117323, 1.0403351955307267, 0.7107262569832402, 0.6073743016759776, 0.7637988826815647, 0.9565363128491625, 0.9928491620111737, 0.9872625698324025, 0.7302793296089385, 2.0124022346368706, 7.677206703910614, 18.473296089385467, 30.3894972067039, 37.48167597765362, 37.3727374301676, 31.062681564245807, 21.124134078212286, 12.350391061452513, 7.258212290502794, 4.5962011173184365, 3.953743016759777, 4.453743016759777, 4.668826815642459, 5.026368715083799, 5.0459217877094975, 4.724692737430169, 4.0263687150838, 2.4509497206703914, 1.0822346368715083, 0.6017877094972067, 0.573854748603352, 0.6157541899441341, 0.7665921787709498, 1.0235754189944135, 0.9844692737430168, 0.8867039106145252, 1.0012290502793304, 0.7023463687150843, 0.5487150837988826, 0.6213407821229049, 0.6436871508379889, 0.5766480446927376, 0.6855865921787712, 0.7526256983240225, 0.5766480446927378, 0.48726256983240257, 0.44256983240223463, 0.47050279329608935, 0.39229050279329625, 0.20793296089385477, 0.18837988826815644, 0.367150837988827, 0.33363128491620136, 0.5347486033519554, 0.786145251396648, 0.9537430167597767, 0.7582122905027935, 0.397877094972067, 0.5403351955307263, 0.5878212290502793, 0.3364245810055867, 0.22189944134078224, 0.5766480446927374, 0.9649162011173187, 0.6744134078212294, 0.33083798882681587, 0.5431284916201119, 0.6157541899441341, 0.749832402234637, 0.5710614525139666, 0.48726256983240235, 0.5570949720670393, 0.4174301675977655, 0.2218994413407822, 0.238659217877095, 0.6045810055865921, 0.7470391061452514, 0.5179888268156426, 0.5124022346368716, 0.4118435754189945, 0.19117318435754202, 0.32525139664804487, 0.31966480446927387, 0.16882681564245816, 0.009608938547486102, 0.3531843575418994, 0.6995530726256982, 0.7051396648044694, 0.5124022346368716, 0.47329608938547485, 0.5878212290502793, 0.2805586592178771, 0.19675977653631302, 0.47050279329608957, 0.3587709497206704, 0.244245810055866, 0.38949720670391064, 0.41463687150838, 0.28055865921787737, 0.1800000000000001, 0.26938547486033526, 0.45374301675977646, 0.48446927374301674, 0.4956424581005586, 0.2637988826815642, 0.12972067039106153, 0.2554189944134079, 0.27497206703910626, 0.261005586592179, 0.24703910614525154, 0.20513966480446932, -0.0518435754189943, -0.10770949720670384, 0.24424581005586607, 0.34201117318435775, 0.4705027932960895, 0.4565363128491622, 0.18000000000000016, 0.29731843575419004, 0.3783240223463688, 0.16882681564245813, 0.08223463687150846, 0.3224581005586594, 0.22189944134078227, 0.0654748603351956, 0.00681564245810061, -0.023910614525139637, 0.14089385474860336, 0.3112849162011175, 0.12692737430167622, 0.02357541899441351, -0.004357541899441347, -0.001564245810055792, 0.23865921787709515, 0.13251396648044703, -0.029497206703910546, 0.07106145251396656, -0.06301675977653633, -0.049050279329608995, 0.2358659217877096, 0.3364245810055868, 0.5738547486033523, 0.49005586592178807, 0.21631284916201132, 0.2386592178770951, 0.15486033519553086, -0.007150837988826686, 0.05150837988826826, 0.28893854748603365, 0.4397765363128491, 0.14368715083798866, 0.33363128491620114, 0.41743016759776547, 0.12692737430167614, 0.32245810055865937, 0.2470391061452515, -0.07977653631284902, 0.11296089385474875, 0.33083798882681575, 0.09061452513966492, -0.17474860335195522, -0.07977653631284909, 0.06826815642458112, 0.07944134078212302, 0.27217877094972076, 0.28614525139664826, 0.11575418994413428, 0.05988826815642468, 0.08502793296089395, 0.009608938547486134, 0.18558659217877096, 0.47050279329608946, 0.3727374301675979, 0.06826815642458114, -0.05743016759776528, 0.08223463687150843, -0.2585474860335196, -0.4205586592178771, -0.1216759776536312, -0.06860335195530717, 0.18558659217877102, 0.4313966480446928, 0.19955307262569846, -0.06860335195530719, 0.1381005586592178, 0.34759776536312853, 0.2135195530726259, -0.08256983240223467, 0.1101675977653632, 0.22469273743016788, 0.004022346368715245, 0.05150837988826826, 0.04312849162011187, -0.018324022346368582, -0.0658100558659217, -0.07139664804469262, -0.06581005586592165, 0.11854748603351964, -0.049050279329608926, -0.14681564245810053, 0.07944134078212298, -0.051843575418994335, -0.029497206703910553, 0.01240223463687163, -0.2529608938547485, 0.04312849162011173, 0.37273743016759786, -0.015530726256983013, -0.0769832402234635, 0.05988826815642466, -0.09653631284916192, -0.009944134078212208, -0.02949720670391054, -0.00715083798882668, 0.10178770949720685, -0.15240223463687147, -0.037877094972067066, 0.00960893854748611, -0.25016759776536296, -0.06022346368715076, 0.36435754189944136, 0.21351955307262577, 0.09340782122905036, 0.1995530726256984, 0.09061452513966493, 0.029162011173184513, 0.20793296089385488, -0.12167597765363122, -0.40659217877094966, 0.023575418994413483, 0.22748603351955313, -0.012737430167597596, -0.06581005586592159, 0.05150837988826823, 0.079441340782123, -0.06301675977653623, -0.009944134078212208, -0.004357541899441236, -0.0462569832402234, 0.1660335195530727, 0.04033519553072633, 0.0012290502793297024, -0.197094972067039, -0.09932960893854738, 0.11575418994413417, -0.08256983240223446, -0.07418994413407806, -0.06581005586592169, -0.1300558659217876, 0.015195530726257074, 0.17162011173184366, 0.08223463687150848, -0.2250279329608937, -0.16636871508379872, 0.19396648044692755, 0.19955307262569844, 0.015195530726257057, -0.07698324022346358, -0.029497206703910504, 0.015195530726257135, -0.09094972067039088, -0.17195530726256977, -0.09374301675977648, -0.018324022346368596, -0.30603351955307256, -0.42614525139664794, -0.04067039106145236, 0.3196648044692739, 0.11575418994413421, -0.032290502793296025, -0.05463687150837987, -0.16078212290502789, 0.26100558659217904, 0.32245810055865953, 0.04871508379888277, -0.27251396648044673, -0.10491620111731817, 0.07385474860335214, -0.09932960893854734, 0.026368715083798996, 0.085027932960894, -0.08256983240223452, -0.39262569832402217, -0.3032402234636869, -0.12446927374301667, -0.01832402234636863, 0.09340782122905039, 0.1939664804469275, 0.048715083798882855, -0.20547486033519535, 0.09340782122905045, 0.21910614525139682, 0.1408938547486035, 0.3811173184357543, 0.09899441340782125]
  out "CH0 (WV on) smoothed":dbl[](array[numeric])=[16.605999999999995, 15.347666666666663, 15.16711111111111, 15.422666666666668, 16.542111111111108, 17.308777777777774, 19.039333333333328, 21.639333333333326, 24.050444444444434, 26.647666666666655, 29.208777777777776, 31.203222222222234, 34.99488888888891, 39.94766666666669, 45.73655555555558, 53.18655555555559, 61.9254444444445, 72.65600000000003, 82.88655555555559, 91.12266666666667, 98.05044444444445, 103.47822222222223, 107.3282222222222, 110.05322222222219, 111.63099999999994, 113.01988888888883, 113.89211111111103, 112.26988888888883, 110.3504444444444, 107.8171111111111, 104.33655555555555, 102.91433333333333, 102.45599999999999, 101.44766666666666, 99.06711111111112, 97.18100000000001, 96.11155555555557, 94.17266666666669, 92.27544444444447, 90.00600000000003, 87.94766666666669, 85.52266666666668, 81.99211111111113, 79.00044444444447, 76.45044444444449, 73.1115555555556, 70.67822222222226, 68.76711111111115, 65.45044444444449, 62.65322222222227, 61.00600000000005, 59.44766666666672, 58.183777777777834, 57.000444444444504, 55.45600000000006, 53.686555555555614, 51.47266666666671, 48.900444444444474, 46.54766666666669, 45.04211111111114, 42.525444444444474, 39.98655555555558, 37.55322222222224, 34.778222222222226, 32.581, 30.183777777777784, 28.050444444444437, 26.008777777777773, 23.817111111111103, 21.830999999999992, 20.28655555555555, 18.667111111111108, 17.09488888888889, 15.814333333333334, 14.831, 14.669888888888888, 14.103222222222222, 13.431000000000003, 13.053222222222226, 12.467111111111116, 12.053222222222228, 11.328222222222227, 10.731000000000003, 10.750444444444447, 10.708777777777783, 10.208777777777783, 9.767111111111117, 9.992111111111114, 10.02266666666667, 9.814333333333337, 9.506000000000002, 8.972666666666669, 8.611555555555556, 7.825444444444442, 7.267111111111108, 7.1087777777777745, 7.164333333333332, 6.817111111111109, 6.236555555555553, 5.867111111111109, 5.480999999999997, 5.517111111111108, 5.430999999999997, 5.083777777777775, 4.914333333333331, 5.0671111111111085, 4.933777777777775, 4.669888888888886, 4.369888888888887, 4.2976666666666645, 4.530999999999997, 4.189333333333332, 3.8837777777777784, 3.8837777777777784, 4.053222222222221, 4.064333333333331, 3.7393333333333327, 3.706, 3.7282222222222217, 3.4810000000000008, 2.8310000000000013, 2.672666666666667, 3.1476666666666677, 3.2643333333333344, 3.2087777777777786, 3.1643333333333343, 2.8865555555555567, 2.4587777777777786, 2.7865555555555566, 2.908777777777779, 2.378222222222224, 2.4393333333333347, 2.3726666666666674, 2.0087777777777784, 2.0393333333333334, 2.1782222222222227, 2.6060000000000008, 2.692111111111112, 2.492111111111112, 2.3504444444444452, 1.8726666666666665, 1.903222222222222, 1.9254444444444445, 1.7171111111111104, 1.9059999999999993, 1.7448888888888883, 1.5698888888888884, 2.022666666666667, 2.0837777777777777, 1.7615555555555549, 1.7809999999999997, 2.1143333333333336, 2.0615555555555556, 1.839333333333333, 1.725444444444444, 1.5865555555555546, 1.4032222222222215, 1.3504444444444434, 1.3726666666666656, 1.3337777777777768, 1.5226666666666655, 1.533777777777777, 1.3171111111111105, 1.503222222222222, 1.5059999999999998, 1.3504444444444434, 1.433777777777777, 1.1754444444444438, 1.1587777777777772, 1.1976666666666658, 1.2309999999999994, 1.0976666666666666, 1.0115555555555553, 1.3171111111111102, 1.053222222222222, 0.8171111111111116, 0.9643333333333333, 1.0532222222222216, 1.1448888888888882, 0.7976666666666663, 0.7393333333333333, 1.1198888888888883, 1.2643333333333322, 0.9782222222222217, 0.583777777777778, 0.753222222222222, 0.8254444444444444, 0.8004444444444445, 0.8921111111111109, 0.7310000000000001, 0.5143333333333338, 0.44211111111111145, 0.34488888888888913, 0.36711111111111117, 0.7865555555555551, 0.8948888888888886, 0.6782222222222225, 0.8504444444444439, 0.7893333333333329, 0.3421111111111113, 0.46433333333333365, 0.6254444444444448, 0.8698888888888885, 0.9226666666666664, 0.5198888888888893, 0.4448888888888891, 0.45600000000000024, 0.5004444444444449, 0.5171111111111115, 0.30877777777777804, 0.3976666666666667, 0.5643333333333337, 0.5643333333333338, 0.8143333333333334, 0.7754444444444446, 0.5921111111111117, 0.5143333333333336, 0.35877777777777786, 0.24211111111111117, 0.2976666666666669, 0.3754444444444449, 0.4476666666666672, 0.6782222222222224, 0.7337777777777779, 0.5060000000000003, 0.358777777777778, 0.38100000000000034, 0.483777777777778, 0.6365555555555555, 0.6726666666666669, 0.6726666666666666, 0.617111111111111, 0.5115555555555557, 0.481, 0.5615555555555559, 0.8254444444444444, 0.578222222222222, 0.4921111111111113, 0.5421111111111112, 0.21433333333333324, 0.20322222222222222, 0.45044444444444465, 0.3921111111111113, 0.24211111111111117, 0.3310000000000002, 0.34488888888888913, 0.5671111111111112, 0.5032222222222223, 0.28100000000000014, 0.36711111111111117, 0.3754444444444445, 0.1671111111111113, 0.1948888888888891, 0.4032222222222224, 0.3532222222222223, 0.21711111111111117, 0.2254444444444445, 0.028222222222222204, 0.025444444444444436, 0.3810000000000001, 0.4698888888888893, 0.4004444444444448, 0.3365555555555557, 0.5115555555555559, 0.36711111111111133, 0.12822222222222238, 0.2671111111111113, 0.39488888888888907, 0.4254444444444446, 0.2087777777777778, 0.12266666666666673, 0.7726666666666666, 2.4060000000000006, 4.639333333333332, 7.339333333333331, 9.956000000000001, 10.331000000000003, 8.292111111111113, 5.575444444444443, 3.2865555555555543, 1.8365555555555557, 1.0698888888888884, 0.8448888888888891, 1.075444444444444, 1.1115555555555547, 1.0476666666666659, 1.1476666666666655, 1.14211111111111, 0.9032222222222215, 0.681, 0.5948888888888892, 0.3615555555555557, -0.05788888888888882, -0.010666666666666574, 0.22266666666666676, 0.2698888888888891, 0.692111111111111, 0.4504444444444442, 0.2643333333333336, 0.2782222222222225, -0.17177777777777756, -0.08011111111111092, 0.28655555555555573, 0.38933333333333353, 0.2671111111111112, 0.2504444444444446, 0.3115555555555556, -0.03566666666666646, 0.08933333333333371, 0.4560000000000002, 0.2948888888888889, 0.25044444444444447, 0.09211111111111117, -0.06899999999999998, -0.1634444444444445, 0.13377777777777783, 0.1810000000000001, -0.2439999999999999, -0.32177777777777766, 0.0032222222222223207, 0.2671111111111112, 0.01433333333333335, 0.07266666666666684, 0.11433333333333348, 0.21711111111111145, 0.3337777777777782, 0.09766666666666672, 0.12822222222222232, 0.019888888888888928, -0.11344444444444442, -0.14677777777777767, 0.047666666666666746, 0.28933333333333344, 0.05044444444444468, 0.24766666666666695, 0.38100000000000017, 0.019888888888888935, 0.183777777777778, 0.26433333333333364, 0.10600000000000015, 0.06988888888888893, 0.1143333333333333, -0.03011111111111109, 0.07822222222222239, 0.30600000000000016, 0.17544444444444454, 0.09766666666666673, 0.025444444444444485, 0.17822222222222245, 0.26433333333333353, 0.39211111111111124, 0.6115555555555559, 0.3365555555555558, 0.10877777777777799, 0.06433333333333349, 0.11155555555555555, 0.10877777777777779, 0.044888888888889034, 0.03933333333333347, -0.027333333333333223, 0.31155555555555586, 0.6476666666666671, 0.46988888888888913, 0.12544444444444458, -0.02177777777777773, -0.3884444444444443, -0.4662222222222221, 0.06433333333333337, -0.024555555555555414, -0.23566666666666652, -0.0078888888888888, -0.0967777777777777, -0.13566666666666663, -0.04122222222222214, -0.0384444444444443, 0.11988888888888899, -0.0828888888888888, -0.14677777777777762, 0.047666666666666746, 0.33377777777777784, 0.46155555555555566, 0.11155555555555569, -0.046777777777777696, -0.013444444444444363, 0.11433333333333341, 0.1976666666666667, 0.2310000000000001, -0.04122222222222216, -0.016222222222222193, -0.0051111111111109, -0.16899999999999982, 0.017111111111111216, 0.039333333333333456, 0.10322222222222227, 0.06988888888888897, 0.02544444444444452, -0.018999999999999913, -0.15788888888888877, -0.07177777777777769, 0.22822222222222227, 0.3365555555555556, 0.06711111111111123, -0.0884444444444443, 0.0615555555555557, 0.36155555555555596, 0.14488888888888918, 0.050444444444444514, 0.36988888888888904, 0.2615555555555557, 0.19211111111111118, -0.018999999999999947, -0.18288888888888877, -0.08566666666666657, 0.20322222222222244, 0.4254444444444447, 0.294888888888889, -0.1467777777777776, -0.02733333333333296, 0.01988888888888929, -0.1939999999999997, 0.2726666666666669, 0.2643333333333335, 0.019888888888888928, -0.041222222222222216, -0.0467777777777778, 0.15599999999999997, 0.07266666666666668, -0.01066666666666656, 0.21155555555555566, -0.0023333333333332706, 0.11711111111111136, 0.11433333333333362, -0.13566666666666657, 0.011555555555555545, 0.10322222222222215, 0.20599999999999996, 0.017111111111111174, -0.155111111111111, -0.09122222222222212, -0.13566666666666655, 0.042111111111111224, 0.21155555555555566, 0.1671111111111112, 0.06988888888888896, -0.0828888888888888, -0.07455555555555549, -0.10788888888888885, -0.11066666666666662, 0.24488888888888916, 0.24766666666666695, -0.16344444444444436, -0.24399999999999994, 0.07544444444444451, 0.10322222222222228, -0.09955555555555551, -0.2162222222222221, -0.24955555555555542, -0.07177777777777773, 0.03933333333333336, 0.014333333333333378, 0.15600000000000028, 0.01711111111111141, -0.10511111111111104, 0.1115555555555557, 0.2532222222222225, 0.2226666666666669, -0.06344444444444437, -0.1856666666666666, 0.1393333333333336, 0.16433333333333358, -0.14677777777777767, -0.2884444444444444, -0.07177777777777775, 0.1476666666666667, -0.030111111111111075, 0.14211111111111113, 0.4226666666666668, 0.1171111111111113, -0.24122222222222212, 0.07544444444444452, 0.20322222222222228, 0.17544444444444451, 0.3365555555555556, 0.36988888888888904, 0.11433333333333345, 0.08100000000000007, 0.25044444444444447, 0.03377777777777782, -0.105111111111111, 0.07822222222222226, 0.08655555555555558, -0.03844444444444439, -0.11622222222222217, -0.11622222222222223, 0.11711111111111114, 0.28655555555555556, 0.23377777777777783, 0.07544444444444454, -0.03844444444444436, 0.21711111111111137, 0.35322222222222244, 0.21711111111111112, 0.08377777777777778, -0.18844444444444416, -0.11899999999999972, -0.1495555555555555, -0.0939999999999999, -0.2356666666666667, -0.32177777777777783, 0.0921111111111112, -0.22455555555555526, -0.41622222222222194, -0.19677777777777766, -0.041222222222222216, 0.09488888888888895, 0.16155555555555567, 0.07544444444444448, -0.0467777777777777, 0.008777777777777811, 0.09211111111111119, -0.038444444444444406, -0.119, 0.06711111111111115, 0.13377777777777777, -0.12733333333333324, -0.04955555555555527, -0.01899999999999985, -0.0023333333333334927, 0.20322222222222208, -0.08288888888888885, -0.24955555555555547, 0.0504444444444445, 0.05600000000000005, -0.060666666666666626, -0.06622222222222218, -0.06622222222222218, -0.06899999999999992, -0.21344444444444438, 0.011555555555555555, -0.0328888888888888, -0.3689999999999999, -0.2523333333333333, -0.11622222222222214, -0.1634444444444444, -0.0051111111111110386, 0.10044444444444456, -0.049555555555555464, -0.09399999999999986, 0.1671111111111113, -0.03288888888888852, 0.014333333333333698, 0.3226666666666668, 0.1282222222222223, 0.14488888888888893, 0.30044444444444457, 0.09211111111111127, -0.11899999999999993]
  out "CH 0 Bin Readings":dbl[](array[numeric])=[28.0, 14.0, 22.0, 20.0, 19.0, 29.0, 26.0, 29.0, 18.0, 29.0, 34.0, 34.0, 33.0, 43.0, 44.0, 57.0, 57.0, 65.0, 70.0, 100.0, 76.0, 97.0, 99.0, 112.0, 99.0, 112.0, 108.0, 109.0, 98.0, 108.0, 111.0, 89.0, 82.0, 96.0, 111.0, 106.0, 101.0, 91.0, 97.0, 85.0, 107.0, 79.0, 78.0, 89.0, 104.0, 88.0, 75.0, 70.0, 70.0, 63.0, 74.0, 61.0, 55.0, 67.0, 54.0, 53.0, 60.0, 63.0, 56.0, 52.0, 47.0, 42.0, 46.0, 39.0, 40.0, 38.0, 37.0, 28.0, 30.0, 33.0, 21.0, 30.0, 29.0, 28.0, 20.0, 26.0, 29.0, 25.0, 21.0, 20.0, 15.0, 25.0, 18.0, 12.0, 15.0, 14.0, 26.0, 12.0, 20.0, 23.0, 18.0, 18.0, 22.0, 23.0, 17.0, 14.0, 15.0, 20.0, 10.0, 12.0, 11.0, 17.0, 7.0, 20.0, 17.0, 16.0, 13.0, 16.0, 5.0, 10.0, 13.0, 6.0, 10.0, 15.0, 16.0, 7.0, 13.0, 11.0, 11.0, 12.0, 14.0, 12.0, 9.0, 13.0, 13.0, 12.0, 15.0, 7.0, 15.0, 11.0, 13.0, 13.0, 10.0, 15.0, 9.0, 9.0, 5.0, 16.0, 8.0, 4.0, 12.0, 10.0, 11.0, 6.0, 11.0, 8.0, 9.0, 15.0, 14.0, 8.0, 14.0, 6.0, 19.0, 6.0, 7.0, 6.0, 13.0, 10.0, 7.0, 8.0, 13.0, 11.0, 10.0, 8.0, 6.0, 8.0, 9.0, 14.0, 9.0, 10.0, 8.0, 9.0, 11.0, 11.0, 12.0, 6.0, 7.0, 4.0, 9.0, 7.0, 12.0, 9.0, 15.0, 3.0, 8.0, 9.0, 10.0, 9.0, 11.0, 9.0, 12.0, 7.0, 7.0, 7.0, 8.0, 11.0, 11.0, 6.0, 6.0, 8.0, 10.0, 12.0, 14.0, 13.0, 9.0, 6.0, 5.0, 8.0, 11.0, 11.0, 7.0, 10.0, 9.0, 6.0, 6.0, 7.0, 7.0, 9.0, 7.0, 8.0, 7.0, 10.0, 6.0, 9.0, 4.0, 6.0, 3.0, 12.0, 11.0, 8.0, 4.0, 8.0, 7.0, 9.0, 4.0, 4.0, 14.0, 5.0, 6.0, 6.0, 4.0, 6.0, 10.0, 11.0, 4.0, 6.0, 6.0, 9.0, 7.0, 11.0, 7.0, 10.0, 8.0, 11.0, 9.0, 9.0, 3.0, 12.0, 12.0, 8.0, 7.0, 6.0, 6.0, 11.0, 9.0, 6.0, 7.0, 7.0, 8.0, 9.0, 13.0, 6.0, 8.0, 9.0, 5.0, 9.0, 13.0, 22.0, 15.0, 14.0, 11.0, 5.0, 10.0, 8.0, 8.0, 8.0, 12.0, 13.0, 11.0, 14.0, 7.0, 7.0, 8.0, 4.0, 11.0, 7.0, 8.0, 6.0, 8.0, 6.0, 6.0, 8.0, 9.0, 14.0, 7.0, 10.0, 7.0, 16.0, 15.0, 6.0, 6.0, 10.0, 6.0, 4.0, 3.0, 10.0, 8.0, 5.0, 6.0, 6.0, 4.0, 8.0, 5.0, 7.0, 5.0, 6.0, 10.0, 11.0, 6.0, 8.0, 10.0, 11.0, 8.0, 10.0, 4.0, 5.0, 8.0, 8.0, 6.0, 4.0, 5.0, 6.0, 4.0, 11.0, 7.0, 6.0, 6.0, 7.0, 7.0, 5.0, 6.0, 6.0, 4.0, 10.0, 3.0, 9.0, 8.0, 5.0, 5.0, 6.0, 12.0, 7.0, 9.0, 12.0, 4.0, 6.0, 7.0, 9.0, 9.0, 5.0, 10.0, 5.0, 5.0, 7.0, 11.0, 12.0, 5.0, 7.0, 6.0, 10.0, 8.0, 12.0, 10.0, 8.0, 5.0, 11.0, 8.0, 12.0, 7.0, 9.0, 5.0, 3.0, 7.0, 12.0, 8.0, 6.0, 5.0, 5.0, 6.0, 4.0, 8.0, 13.0, 5.0, 10.0, 10.0, 8.0, 4.0, 9.0, 12.0, 6.0, 7.0, 8.0, 7.0, 6.0, 4.0, 3.0, 8.0, 9.0, 9.0, 7.0, 7.0, 5.0, 11.0, 6.0, 5.0, 0.0, 8.0, 2.0, 3.0, 8.0, 9.0, 11.0, 8.0, 4.0, 7.0, 6.0, 4.0, 4.0, 6.0, 6.0, 4.0, 7.0, 6.0, 5.0, 7.0, 11.0, 2.0, 8.0, 5.0, 6.0, 9.0, 8.0, 10.0, 8.0, 8.0, 6.0, 11.0, 11.0, 7.0, 9.0, 7.0, 8.0, 6.0, 6.0, 12.0, 12.0, 12.0, 7.0, 11.0, 11.0, 6.0, 8.0, 8.0, 8.0, 7.0, 7.0, 7.0, 8.0, 6.0, 6.0, 13.0, 7.0, 7.0, 12.0, 8.0, 6.0, 5.0, 6.0, 5.0, 9.0, 7.0, 3.0, 7.0, 7.0, 6.0, 8.0, 5.0, 11.0, 8.0, 10.0, 9.0, 6.0, 7.0, 10.0, 8.0, 9.0, 5.0, 5.0, 11.0, 7.0, 9.0, 8.0, 6.0, 8.0, 12.0, 4.0, 9.0, 7.0, 3.0, 11.0, 7.0, 4.0, 12.0, 6.0, 7.0, 6.0, 7.0, 5.0, 10.0, 10.0, 5.0, 9.0, 8.0, 9.0, 9.0, 10.0, 15.0, 8.0, 10.0, 7.0, 7.0, 4.0, 7.0, 9.0, 4.0, 8.0, 3.0, 10.0, 3.0, 4.0, 5.0, 8.0, 6.0, 7.0, 4.0, 5.0, 7.0, 9.0, 6.0]
  out "Range Corrected Altitude Array":dbl[](array[numeric])=[1406.25, 5625.0, 12656.25, 22500.0, 35156.25, 50625.0, 68906.25, 90000.0, 113906.25, 140625.0, 170156.25, 202500.0, 237656.25, 275625.0, 316406.25, 360000.0, 406406.25, 455625.0, 507656.25, 562500.0, 620156.25, 680625.0, 743906.25, 810000.0, 878906.25, 950625.0, 1025156.25, 1102500.0, 1182656.25, 1265625.0, 1351406.25, 1440000.0, 1531406.25, 1625625.0, 1722656.25, 1822500.0, 1925156.25, 2030625.0, 2138906.25, 2250000.0, 2363906.25, 2480625.0, 2600156.25, 2722500.0, 2847656.25, 2975625.0, 3106406.25, 3240000.0, 3376406.25, 3515625.0, 3657656.25, 3802500.0, 3950156.25, 4100625.0, 4253906.25, 4410000.0, 4568906.25, 4730625.0, 4895156.25, 5062500.0, 5232656.25, 5405625.0, 5581406.25, 5760000.0, 5941406.25, 6125625.0, 6312656.25, 6502500.0, 6695156.25, 6890625.0, 7088906.25, 7290000.0, 7493906.25, 7700625.0, 7910156.25, 8122500.0, 8337656.25, 8555625.0, 8776406.25, 9000000.0, 9226406.25, 9455625.0, 9687656.25, 9922500.0, 10160156.25, 10400625.0, 10643906.25, 10890000.0, 11138906.25, 11390625.0, 11645156.25, 11902500.0, 12162656.25, 12425625.0, 12691406.25, 12960000.0, 13231406.25, 13505625.0, 13782656.25, 14062500.0, 14345156.25, 14630625.0, 14918906.25, 15210000.0, 15503906.25, 15800625.0, 16100156.25, 16402500.0, 16707656.25, 17015625.0, 17326406.25, 17640000.0, 17956406.25, 18275625.0, 18597656.25, 18922500.0, 19250156.25, 19580625.0, 19913906.25, 20250000.0, 20588906.25, 20930625.0, 21275156.25, 21622500.0, 21972656.25, 22325625.0, 22681406.25, 23040000.0, 23401406.25, 23765625.0, 24132656.25, 24502500.0, 24875156.25, 25250625.0, 25628906.25, 26010000.0, 26393906.25, 26780625.0, 27170156.25, 27562500.0, 27957656.25, 28355625.0, 28756406.25, 29160000.0, 29566406.25, 29975625.0, 30387656.25, 30802500.0, 31220156.25, 31640625.0, 32063906.25, 32490000.0, 32918906.25, 33350625.0, 33785156.25, 34222500.0, 34662656.25, 35105625.0, 35551406.25, 36000000.0, 36451406.25, 36905625.0, 37362656.25, 37822500.0, 38285156.25, 38750625.0, 39218906.25, 39690000.0, 40163906.25, 40640625.0, 41120156.25, 41602500.0, 42087656.25, 42575625.0, 43066406.25, 43560000.0, 44056406.25, 44555625.0, 45057656.25, 45562500.0, 46070156.25, 46580625.0, 47093906.25, 47610000.0, 48128906.25, 48650625.0, 49175156.25, 49702500.0, 50232656.25, 50765625.0, 51301406.25, 51840000.0, 52381406.25, 52925625.0, 53472656.25, 54022500.0, 54575156.25, 55130625.0, 55688906.25, 56250000.0, 56813906.25, 57380625.0, 57950156.25, 58522500.0, 59097656.25, 59675625.0, 60256406.25, 60840000.0, 61426406.25, 62015625.0, 62607656.25, 63202500.0, 63800156.25, 64400625.0, 65003906.25, 65610000.0, 66218906.25, 66830625.0, 67445156.25, 68062500.0, 68682656.25, 69305625.0, 69931406.25, 70560000.0, 71191406.25, 71825625.0, 72462656.25, 73102500.0, 73745156.25, 74390625.0, 75038906.25, 75690000.0, 76343906.25, 77000625.0, 77660156.25, 78322500.0, 78987656.25, 79655625.0, 80326406.25, 81000000.0, 81676406.25, 82355625.0, 83037656.25, 83722500.0, 84410156.25, 85100625.0, 85793906.25, 86490000.0, 87188906.25, 87890625.0, 88595156.25, 89302500.0, 90012656.25, 90725625.0, 91441406.25, 92160000.0, 92881406.25, 93605625.0, 94332656.25, 95062500.0, 95795156.25, 96530625.0, 97268906.25, 98010000.0, 98753906.25, 99500625.0, 100250156.25, 101002500.0, 101757656.25, 102515625.0, 103276406.25, 104040000.0, 104806406.25, 105575625.0, 106347656.25, 107122500.0, 107900156.25, 108680625.0, 109463906.25, 110250000.0, 111038906.25, 111830625.0, 112625156.25, 113422500.0, 114222656.25, 115025625.0, 115831406.25, 116640000.0, 117451406.25, 118265625.0, 119082656.25, 119902500.0, 120725156.25, 121550625.0, 122378906.25, 123210000.0, 124043906.25, 124880625.0, 125720156.25, 126562500.0, 127407656.25, 128255625.0, 129106406.25, 129960000.0, 130816406.25, 131675625.0, 132537656.25, 133402500.0, 134270156.25, 135140625.0, 136013906.25, 136890000.0, 137768906.25, 138650625.0, 139535156.25, 140422500.0, 141312656.25, 142205625.0, 143101406.25, 144000000.0, 144901406.25, 145805625.0, 146712656.25, 147622500.0, 148535156.25, 149450625.0, 150368906.25, 151290000.0, 152213906.25, 153140625.0, 154070156.25, 155002500.0, 155937656.25, 156875625.0, 157816406.25, 158760000.0, 159706406.25, 160655625.0, 161607656.25, 162562500.0, 163520156.25, 164480625.0, 165443906.25, 166410000.0, 167378906.25, 168350625.0, 169325156.25, 170302500.0, 171282656.25, 172265625.0, 173251406.25, 174240000.0, 175231406.25, 176225625.0, 177222656.25, 178222500.0, 179225156.25, 180230625.0, 181238906.25, 182250000.0, 183263906.25, 184280625.0, 185300156.25, 186322500.0, 187347656.25, 188375625.0, 189406406.25, 190440000.0, 191476406.25, 192515625.0, 193557656.25, 194602500.0, 195650156.25, 196700625.0, 197753906.25, 198810000.0, 199868906.25, 200930625.0, 201995156.25, 203062500.0, 204132656.25, 205205625.0, 206281406.25, 207360000.0, 208441406.25, 209525625.0, 210612656.25, 211702500.0, 212795156.25, 213890625.0, 214988906.25, 216090000.0, 217193906.25, 218300625.0, 219410156.25, 220522500.0, 221637656.25, 222755625.0, 223876406.25, 225000000.0, 226126406.25, 227255625.0, 228387656.25, 229522500.0, 230660156.25, 231800625.0, 232943906.25, 234090000.0, 235238906.25, 236390625.0, 237545156.25, 238702500.0, 239862656.25, 241025625.0, 242191406.25, 243360000.0, 244531406.25, 245705625.0, 246882656.25, 248062500.0, 249245156.25, 250430625.0, 251618906.25, 252810000.0, 254003906.25, 255200625.0, 256400156.25, 257602500.0, 258807656.25, 260015625.0, 261226406.25, 262440000.0, 263656406.25, 264875625.0, 266097656.25, 267322500.0, 268550156.25, 269780625.0, 271013906.25, 272250000.0, 273488906.25, 274730625.0, 275975156.25, 277222500.0, 278472656.25, 279725625.0, 280981406.25, 282240000.0, 283501406.25, 284765625.0, 286032656.25, 287302500.0, 288575156.25, 289850625.0, 291128906.25, 292410000.0, 293693906.25, 294980625.0, 296270156.25, 297562500.0, 298857656.25, 300155625.0, 301456406.25, 302760000.0, 304066406.25, 305375625.0, 306687656.25, 308002500.0, 309320156.25, 310640625.0, 311963906.25, 313290000.0, 314618906.25, 315950625.0, 317285156.25, 318622500.0, 319962656.25, 321305625.0, 322651406.25, 324000000.0, 325351406.25, 326705625.0, 328062656.25, 329422500.0, 330785156.25, 332150625.0, 333518906.25, 334890000.0, 336263906.25, 337640625.0, 339020156.25, 340402500.0, 341787656.25, 343175625.0, 344566406.25, 345960000.0, 347356406.25, 348755625.0, 350157656.25, 351562500.0, 352970156.25, 354380625.0, 355793906.25, 357210000.0, 358628906.25, 360050625.0, 361475156.25, 362902500.0, 364332656.25, 365765625.0, 367201406.25, 368640000.0, 370081406.25, 371525625.0, 372972656.25, 374422500.0, 375875156.25, 377330625.0, 378788906.25, 380250000.0, 381713906.25, 383180625.0, 384650156.25, 386122500.0, 387597656.25, 389075625.0, 390556406.25, 392040000.0, 393526406.25, 395015625.0, 396507656.25, 398002500.0, 399500156.25, 401000625.0, 402503906.25, 404010000.0, 405518906.25, 407030625.0, 408545156.25, 410062500.0, 411582656.25, 413105625.0, 414631406.25, 416160000.0, 417691406.25, 419225625.0, 420762656.25, 422302500.0, 423845156.25, 425390625.0, 426938906.25, 428490000.0, 430043906.25, 431600625.0, 433160156.25, 434722500.0, 436287656.25, 437855625.0, 439426406.25, 441000000.0]
  out "Altitude Array (km)":dbl[](array[numeric])=[0.0375, 0.075, 0.11249999999999999, 0.15, 0.1875, 0.225, 0.26249999999999996, 0.3, 0.33749999999999997, 0.37499999999999994, 0.4125, 0.44999999999999996, 0.48749999999999993, 0.525, 0.5625, 0.6, 0.6375, 0.6749999999999999, 0.7124999999999999, 0.75, 0.7875, 0.825, 0.8624999999999999, 0.8999999999999999, 0.9374999999999999, 0.975, 1.0125, 1.05, 1.0875000000000001, 1.125, 1.1625, 1.2, 1.2375, 1.2750000000000001, 1.3125, 1.35, 1.3875, 1.425, 1.4625000000000001, 1.5, 1.5375, 1.575, 1.6125, 1.6500000000000001, 1.6875, 1.725, 1.7625, 1.8, 1.8375, 1.875, 1.9125, 1.95, 1.9875, 2.025, 2.0625, 2.1, 2.1375, 2.175, 2.2125, 2.25, 2.2875, 2.325, 2.3625, 2.4, 2.4375, 2.475, 2.5125, 2.55, 2.5875, 2.625, 2.6625, 2.7, 2.7375, 2.775, 2.8125, 2.85, 2.8875, 2.925, 2.9625, 3.0, 3.0375, 3.075, 3.1125, 3.15, 3.1875, 3.225, 3.2625, 3.3, 3.3375, 3.375, 3.4125, 3.45, 3.4875, 3.525, 3.5625, 3.6, 3.6374999999999997, 3.675, 3.7125, 3.75, 3.7875, 3.8249999999999997, 3.8625, 3.9, 3.9375, 3.975, 4.012499999999999, 4.05, 4.0874999999999995, 4.124999999999999, 4.1625, 4.199999999999999, 4.2375, 4.2749999999999995, 4.312499999999999, 4.35, 4.387499999999999, 4.425, 4.4624999999999995, 4.499999999999999, 4.5375, 4.574999999999999, 4.6125, 4.6499999999999995, 4.687499999999999, 4.725, 4.762499999999999, 4.8, 4.8374999999999995, 4.874999999999999, 4.9125, 4.949999999999999, 4.9875, 5.0249999999999995, 5.062499999999999, 5.1, 5.137499999999999, 5.175, 5.2124999999999995, 5.249999999999999, 5.2875, 5.324999999999999, 5.3625, 5.3999999999999995, 5.437499999999999, 5.475, 5.512499999999999, 5.55, 5.5874999999999995, 5.624999999999999, 5.6625, 5.699999999999999, 5.7375, 5.7749999999999995, 5.812499999999999, 5.85, 5.887499999999999, 5.925, 5.9624999999999995, 5.999999999999999, 6.0375, 6.074999999999999, 6.1125, 6.1499999999999995, 6.187499999999999, 6.225, 6.262499999999999, 6.3, 6.3374999999999995, 6.374999999999999, 6.4125, 6.449999999999999, 6.4875, 6.5249999999999995, 6.562499999999999, 6.6, 6.637499999999999, 6.675, 6.7124999999999995, 6.749999999999999, 6.7875, 6.824999999999999, 6.8625, 6.8999999999999995, 6.937499999999999, 6.975, 7.012499999999999, 7.05, 7.0874999999999995, 7.124999999999999, 7.1625, 7.199999999999999, 7.237499999999999, 7.2749999999999995, 7.312499999999999, 7.35, 7.387499999999999, 7.424999999999999, 7.4624999999999995, 7.499999999999999, 7.5375, 7.574999999999999, 7.612499999999999, 7.6499999999999995, 7.687499999999999, 7.725, 7.762499999999999, 7.799999999999999, 7.8374999999999995, 7.874999999999999, 7.9125, 7.949999999999999, 7.987499999999999, 8.025, 8.0625, 8.1, 8.1375, 8.174999999999999, 8.212499999999999, 8.25, 8.2875, 8.325, 8.362499999999999, 8.399999999999999, 8.4375, 8.475, 8.5125, 8.549999999999999, 8.587499999999999, 8.625, 8.6625, 8.7, 8.737499999999999, 8.774999999999999, 8.8125, 8.85, 8.8875, 8.924999999999999, 8.962499999999999, 9.0, 9.0375, 9.075, 9.112499999999999, 9.149999999999999, 9.1875, 9.225, 9.2625, 9.299999999999999, 9.337499999999999, 9.375, 9.4125, 9.45, 9.487499999999999, 9.524999999999999, 9.5625, 9.6, 9.6375, 9.674999999999999, 9.712499999999999, 9.75, 9.7875, 9.825, 9.862499999999999, 9.899999999999999, 9.9375, 9.975, 10.0125, 10.049999999999999, 10.087499999999999, 10.125, 10.1625, 10.2, 10.237499999999999, 10.274999999999999, 10.3125, 10.35, 10.3875, 10.424999999999999, 10.462499999999999, 10.5, 10.5375, 10.575, 10.612499999999999, 10.649999999999999, 10.6875, 10.725, 10.7625, 10.799999999999999, 10.837499999999999, 10.875, 10.9125, 10.95, 10.987499999999999, 11.024999999999999, 11.0625, 11.1, 11.1375, 11.174999999999999, 11.212499999999999, 11.25, 11.2875, 11.325, 11.362499999999999, 11.399999999999999, 11.4375, 11.475, 11.5125, 11.549999999999999, 11.587499999999999, 11.625, 11.6625, 11.7, 11.737499999999999, 11.774999999999999, 11.8125, 11.85, 11.8875, 11.924999999999999, 11.962499999999999, 12.0, 12.0375, 12.075, 12.112499999999999, 12.149999999999999, 12.1875, 12.225, 12.2625, 12.299999999999999, 12.337499999999999, 12.375, 12.4125, 12.45, 12.487499999999999, 12.524999999999999, 12.5625, 12.6, 12.6375, 12.674999999999999, 12.712499999999999, 12.75, 12.7875, 12.825, 12.862499999999999, 12.899999999999999, 12.9375, 12.975, 13.0125, 13.049999999999999, 13.087499999999999, 13.125, 13.1625, 13.2, 13.237499999999999, 13.274999999999999, 13.3125, 13.35, 13.3875, 13.424999999999999, 13.462499999999999, 13.5, 13.5375, 13.575, 13.612499999999999, 13.649999999999999, 13.6875, 13.725, 13.7625, 13.799999999999999, 13.837499999999999, 13.875, 13.9125, 13.95, 13.987499999999999, 14.024999999999999, 14.0625, 14.1, 14.1375, 14.174999999999999, 14.212499999999999, 14.25, 14.2875, 14.325, 14.362499999999999, 14.399999999999999, 14.437499999999998, 14.475, 14.5125, 14.549999999999999, 14.587499999999999, 14.624999999999998, 14.6625, 14.7, 14.737499999999999, 14.774999999999999, 14.812499999999998, 14.85, 14.8875, 14.924999999999999, 14.962499999999999, 14.999999999999998, 15.0375, 15.075, 15.112499999999999, 15.149999999999999, 15.187499999999998, 15.225, 15.2625, 15.299999999999999, 15.337499999999999, 15.374999999999998, 15.4125, 15.45, 15.487499999999999, 15.524999999999999, 15.562499999999998, 15.6, 15.6375, 15.674999999999999, 15.712499999999999, 15.749999999999998, 15.7875, 15.825, 15.862499999999999, 15.899999999999999, 15.937499999999998, 15.975, 16.0125, 16.05, 16.087500000000002, 16.125, 16.1625, 16.2, 16.2375, 16.275000000000002, 16.3125, 16.35, 16.3875, 16.425, 16.462500000000002, 16.5, 16.5375, 16.575, 16.6125, 16.650000000000002, 16.6875, 16.725, 16.7625, 16.8, 16.837500000000002, 16.875, 16.9125, 16.95, 16.9875, 17.025000000000002, 17.0625, 17.1, 17.1375, 17.175, 17.212500000000002, 17.25, 17.2875, 17.325, 17.3625, 17.400000000000002, 17.4375, 17.475, 17.5125, 17.55, 17.587500000000002, 17.625, 17.6625, 17.7, 17.7375, 17.775000000000002, 17.8125, 17.85, 17.8875, 17.925, 17.962500000000002, 18.0, 18.0375, 18.075, 18.1125, 18.150000000000002, 18.1875, 18.225, 18.2625, 18.3, 18.337500000000002, 18.375, 18.4125, 18.45, 18.4875, 18.525000000000002, 18.5625, 18.6, 18.6375, 18.675, 18.712500000000002, 18.75, 18.7875, 18.825, 18.8625, 18.900000000000002, 18.9375, 18.975, 19.0125, 19.05, 19.087500000000002, 19.125, 19.1625, 19.2, 19.2375, 19.275000000000002, 19.3125, 19.35, 19.3875, 19.425, 19.462500000000002, 19.5, 19.5375, 19.575, 19.6125, 19.650000000000002, 19.6875, 19.725, 19.7625, 19.8, 19.837500000000002, 19.875, 19.9125, 19.95, 19.9875, 20.025000000000002, 20.0625, 20.1, 20.1375, 20.175, 20.212500000000002, 20.25, 20.2875, 20.325, 20.3625, 20.400000000000002, 20.4375, 20.475, 20.5125, 20.55, 20.587500000000002, 20.625, 20.6625, 20.7, 20.7375, 20.775000000000002, 20.8125, 20.85, 20.8875, 20.925, 20.962500000000002, 21.0]
  out "WV Offline Pulse Energy":dbl=1581.0
  out "WV Online Pulse Energy":dbl=1627.0
  in  "Instrument Control":T5(tab)=enum."WS"
  in  "Device In":refnum<visa-resource-name>="GPIB0::10::INSTR"
  in  "Settings":T6={"Module"=enum."WV Online TEC", "WV Online TEC"=23.067000000001702, "WV Online LD"=0.175, "WV Offline TEC"=29.4954500000005, "WV Offline LD"=0.17, "WV Etalon TEC"=26.6, "HSRL Etalon TEC"=22.51, "HSRL TEC"=18.630000000001097, "HSRL LD"=0.16} {"HSRL LD" min=0.0 max=0.18 step=0.001 format="%.3p"; "HSRL TEC" min=14.0 max=28.0 step=0.1 format="%.3g"; "WV Offline LD" min=0.0 max=0.18 step=0.001 format="%.3p"; "WV Online LD" min=0.0 max=0.18 step=0.001 format="%.3p"; "HSRL Etalon TEC" format="%.2g"; "WV Etalon TEC" format="%.2g"; "WV Offline TEC" min=16.0 max=30.0 step=0.1 format="%.3g"; "WV Online TEC" min=14.0 max=28.0 step=0.1 format="%.3g"}
  out "Readings":T7={"Pro8000"=TRUE, "WV OnLine TEC"=23.0738468, "WV Online TEC"=TRUE, "WV Online LD"=0.175105482, "WV Online LD"=TRUE, "WV Offline TEC"=29.5094547, "WV Offline TEC"=TRUE, "WV Offline LD"=0.170373052, "WV Offline LD"=TRUE, "WV EtalonTEC"=26.6305122, "WV Etalon TEC"=TRUE, "HSRL Etalon TEC"=23.4953423, "HSRL Etalon TEC"=TRUE, "HSRL TEC"=18.6411381, "HSRL TEC "=TRUE, "HSRL LD"=0.160271496, "HSRL LD"=TRUE} {"HSRL LD" format="%.3p"; "HSRL TEC" format="%.3g"; "WV Offline LD" format="%.3p"; "WV Online LD" format="%.3p"; "HSRL Etalon TEC" format="%.3g"; "WV EtalonTEC" format="%.3g"; "WV Offline TEC" format="%.3g"; "WV OnLine TEC" format="%.3g"}
  in  "Pulse B Polarity":enum32{"Low", "High"}(ring)=enum."High"
  in  "Pulse A Delay(ns)":u32=1040 min=80 max=327600
  in  "Pulse B Delay(ns)":u32=170000 min=80 max=327600 step=1
  in  "Accumulation Delay(ns)":u32=10 min=10 max=1270 step=1
  in  "Sync Pulse Polarity":enum32{"Low", "High"}(ring)=enum."High"
  in  "Pulse A Polarity":enum32{"Low", "High"}(ring)=enum."High"
  in  "Number of Bins":u32=560 min=2 max=4095 step=1
  in  "Number of Accumulates":u32=14285 min=1 max=32767 step=1
  in  "Time Resolution Per Bin(ns)":u32=250 min=5 max=1063 step=1
  out "AMCS_Profile":i32=31
  in  "WV Online Set (nm)":dbl=828.193 format="%.5f"
  out "WV Online Read (nm)":dbl=828.1929749620756 format="%.5f"
  out "WV Offline Read (nm)":dbl=828.2926338731692 format="%.5f"
  in  "WV Offline Set (nm)":dbl=828.29265 format="%.5f"
  in  "Bristol In":i32=3
  out "Bristol Out":i32
  out "Online_Diff":dbl=-2.503792438801611e-05 format="%#_3e"
  out "Oflline_Diff":dbl=-1.6126830814755522e-05 format="%#_3e"
  out "WV Online Locked":bool=TRUE
  out "WV Oflline Locked":bool=TRUE
  in  "calculate absorption cross sections":bool
  in  "Online_Tol":dbl=5e-05 format="%#_15g"
  in  "Cancel online":bool
  in  "Offline_Tol":dbl=5e-05 format="%#_15g"
  in  "Cancel Offline":bool
  in  "temp step size":dbl=0.0005 format="%#_6p"
  in  "HSRL_Tol":dbl=7.5e-05 format="%#_15g"
  out "HSRL_Diff":dbl=9.648186164668004e-06 format="%#_3e"
  in  "Cancel HSRL":bool
  out "HSRL Locked":bool=TRUE
  out "HSRL Read (nm)":dbl=780.2461296481862 format="%.5f"
  in  "HSRL Set (nm)":dbl=780.24612 format="%#.5f"
  in  "Smoothing Range":dbl=75.0
  in  "Total DIAL Integration Time (Minutes)":i32=3
  in  "Data Reads (number of loops)":i32=1
  in  "Total Aerosol Integration Time (Minutes)":dbl=0.08
  in  "Scalar Wait Time":u32
  out "Smoothed Bins":dbl=2.0
  out "gate size":dbl=37.5
  in  "Receiver Scale Factor":dbl=0.75
  in  "NewportIn":string
  in  "logging":bool
  out "Newport Device Key":string
  in  "SampleSize":i32=2
  out "NewportRef":refnum<k24>
  in  "Switch Comm Port":refnum<visa-resource-name>="COM3"
  out "FF_On_Ref":refnum<file>
  out "FF_On_Ptr":i64=4242736 format="%.2p"
  out "FF_Off_Ref":refnum<file>
  out "FF_Off_Ptr":i64=4238208 format="%.2p"
  out "NF_On_Ref":refnum<file>
  out "NF_On_Ptr":i64=4242736 format="%.2p"
  out "NF_Off_Ref":refnum<file>
  out "NF_Off_Ptr":i64=4238208 format="%.2p"
  out "DataOpen":bool=TRUE
  out "File Path_Far Field (out)":string="C:\\Users\\eol-lidar\\Desktop\\SharedTeleWVData\\171019FF\\06"
  out "File Path_Near Field (out)":string="C:\\Users\\eol-lidar\\Desktop\\SharedTeleWVData\\171019NF\\06"
  in  "Data File DIR (in)":string="C:\\Users\\eol-lidar\\Desktop\\SharedTeleWVData\\"
  out "TRHP":T8={"Temp C"=4.895909645909647, "RelH %"=48.92551892551892, "Press hPa"=838.5714285714286, "AbH g/m^3"=3.037240537240537}
  in  "WS visa":refnum<visa-resource-name>="COM2"
  in  "WS_On/Off":bool=TRUE
  in  "bins":u32=560 min=2 max=4095 step=1
  out "y offset":u32=10
  in  "ns scale":u32=250
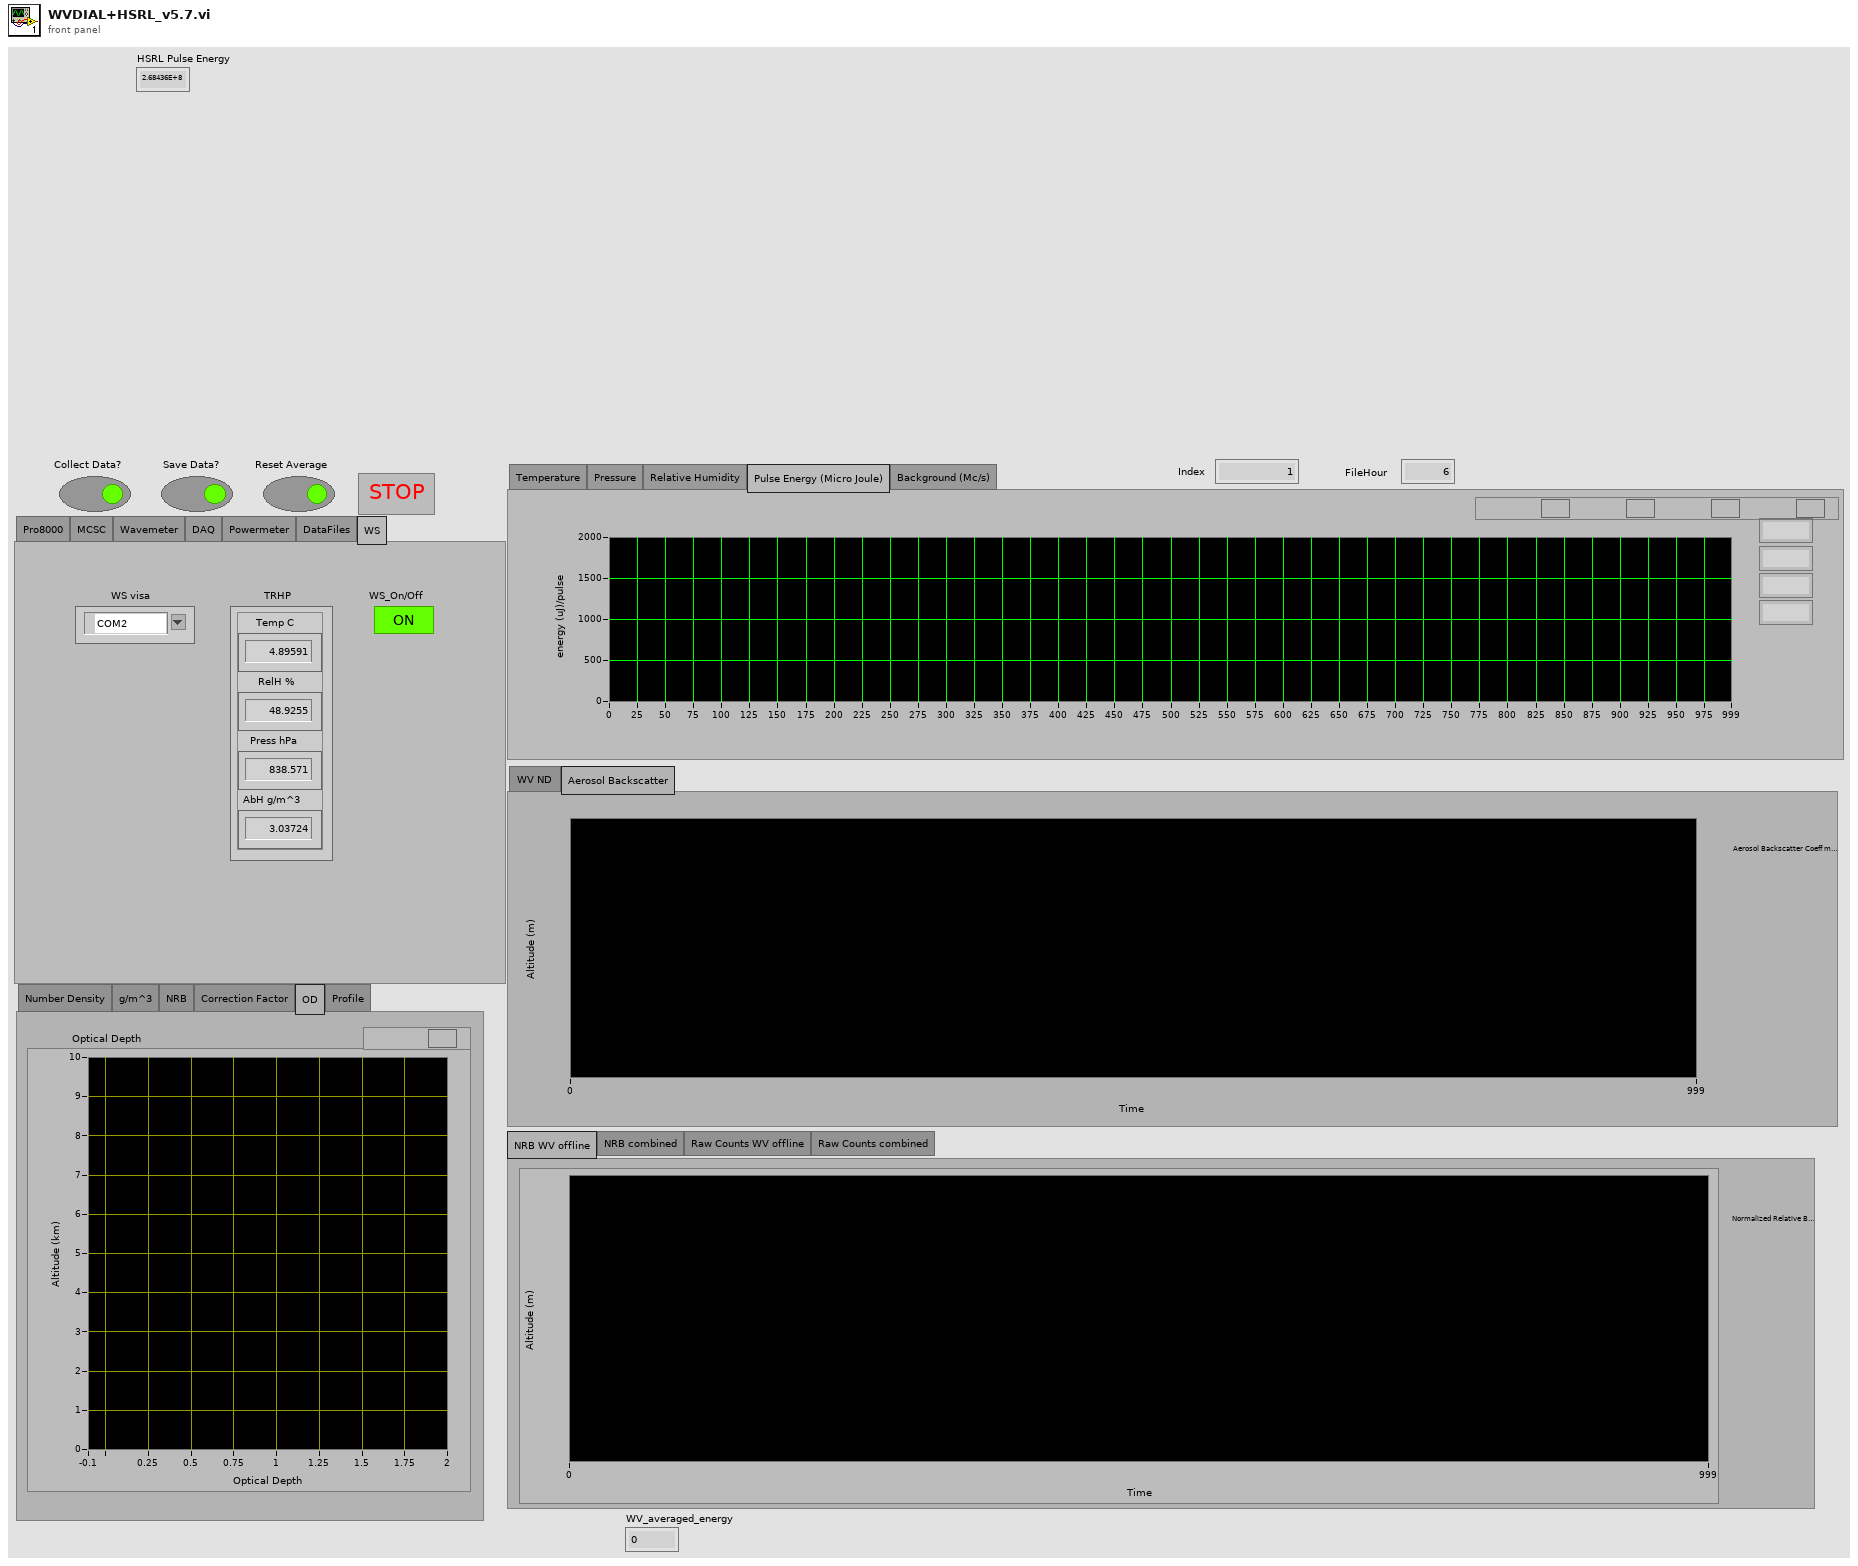
[diagram p1: front panel]
types:
  T1 = enum32{"NRB WV offline", "NRB combined", "Raw Counts WV offline", "Raw Counts combined"}
  T2 = enum32{"Number Density", "g/m^3", "NRB", "Correction Factor", "OD", "Profile"}
  T3 = enum32{"Temperature", "Pressure", "Relative Humidity", "Pulse Energy (Micro Joule)", "Background (Mc/s)"}
  T4 = cluster{"WV Online Pulse Energy":dbl, "WV_averaged_energy":dbl, "HSRL":dbl, "WV_averaged_energy":dbl}
  T5 = enum32{"Pro8000", "MCSC", "Wavemeter", "DAQ", "Powermeter", "DataFiles", "WS"}
  T6 = cluster{"Module":enum16{"WV Online TEC", "WV Online LD", "WV Offline TEC", "WV Offline LD", "WV Etalon TEC", "HSRL Etalon TEC", "HSRL TEC", "HSRL LD"}, "WV Online TEC":dbl, "WV Online LD":dbl, "WV Offline TEC":dbl, "WV Offline LD":dbl, "WV Etalon TEC":dbl, "HSRL Etalon TEC":dbl, "HSRL TEC":dbl, "HSRL LD":dbl}
  T7 = cluster{"Pro8000":bool, "WV OnLine TEC":dbl, "WV Online TEC":bool, "WV Online LD":dbl, "WV Online LD":bool, "WV Offline TEC":dbl, "WV Offline TEC":bool, "WV Offline LD":dbl, "WV Offline LD":bool, "WV EtalonTEC":dbl, "WV Etalon TEC":bool, "HSRL Etalon TEC":dbl, "HSRL Etalon TEC":bool, "HSRL TEC":dbl, "HSRL TEC ":bool, "HSRL LD":dbl, "HSRL LD":bool}
  T8 = cluster{"Temp C":dbl, "RelH %":dbl, "Press hPa":dbl, "AbH g/m^3":dbl}
  T9 = enum16{"Open_TL", "Close_TL", "Verify_ID", "TEC_Sensor", "SET", "READ", "ON", "OFF", "Set_Limits", "Read_Limits", "Enable_Status", "Read_Status"}
  T10 = enum16{"Initialize ILX", "Set ON T", "Set Off T", "Set ON I", "Set Off I", "Set On Lim", "Set Off Lim", "Read ILX", "TEC ON/OFF", "LASER ON/OFF", "Status?", "ILX OFF"}
  T11 = enum16{"open", "replace", "create", "open or create", "replace or create", "replace or create with confirmation"}
  T12 = enum16{"WV Online TEC", "WV Online LD", "WV Offline TEC", "WV Offline LD", "WV Etalon TEC", "HSRL Etalon TEC", "HSRL TEC", "HSRL LD"}
  T13 = cluster{"Temp":dbl, "RelH":dbl, "Press":dbl, "AbH":dbl}
  T14 = typedef "LVDateTimeRec.ctl" = cluster{"fractional second":dbl, "second":i32, "minute":i32, "hour":i32, "day of month":i32, "month":i32, "year":i32, "day of week":i32, "day of year":i32, "DST":i32}
  T15 = cluster{"WV Online Pulse Energy":dbl, "WV Offline Pulse Energy":dbl, "HSRL Pulse Energy":dbl, "WV_averaged_energy":dbl}
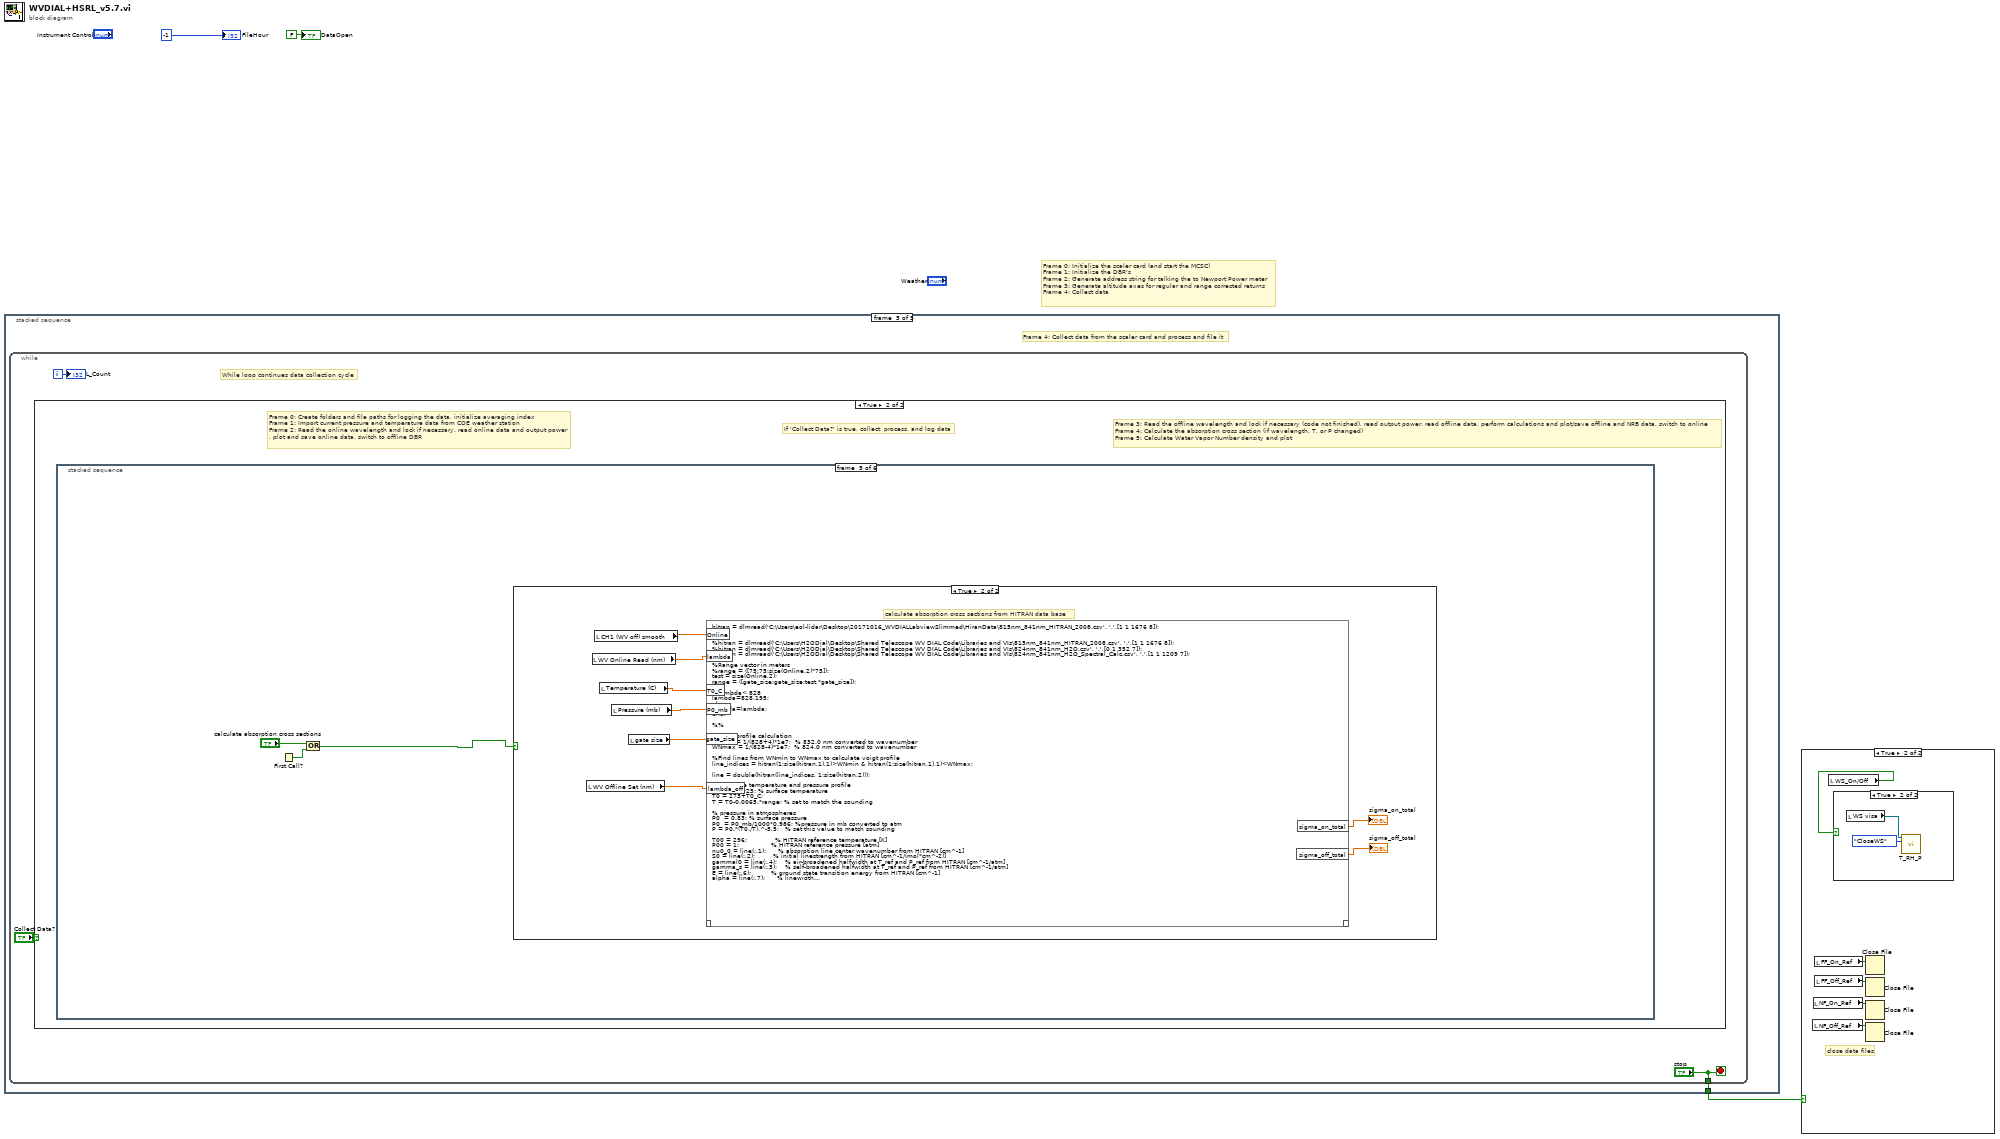
[diagram p0: block diagram]
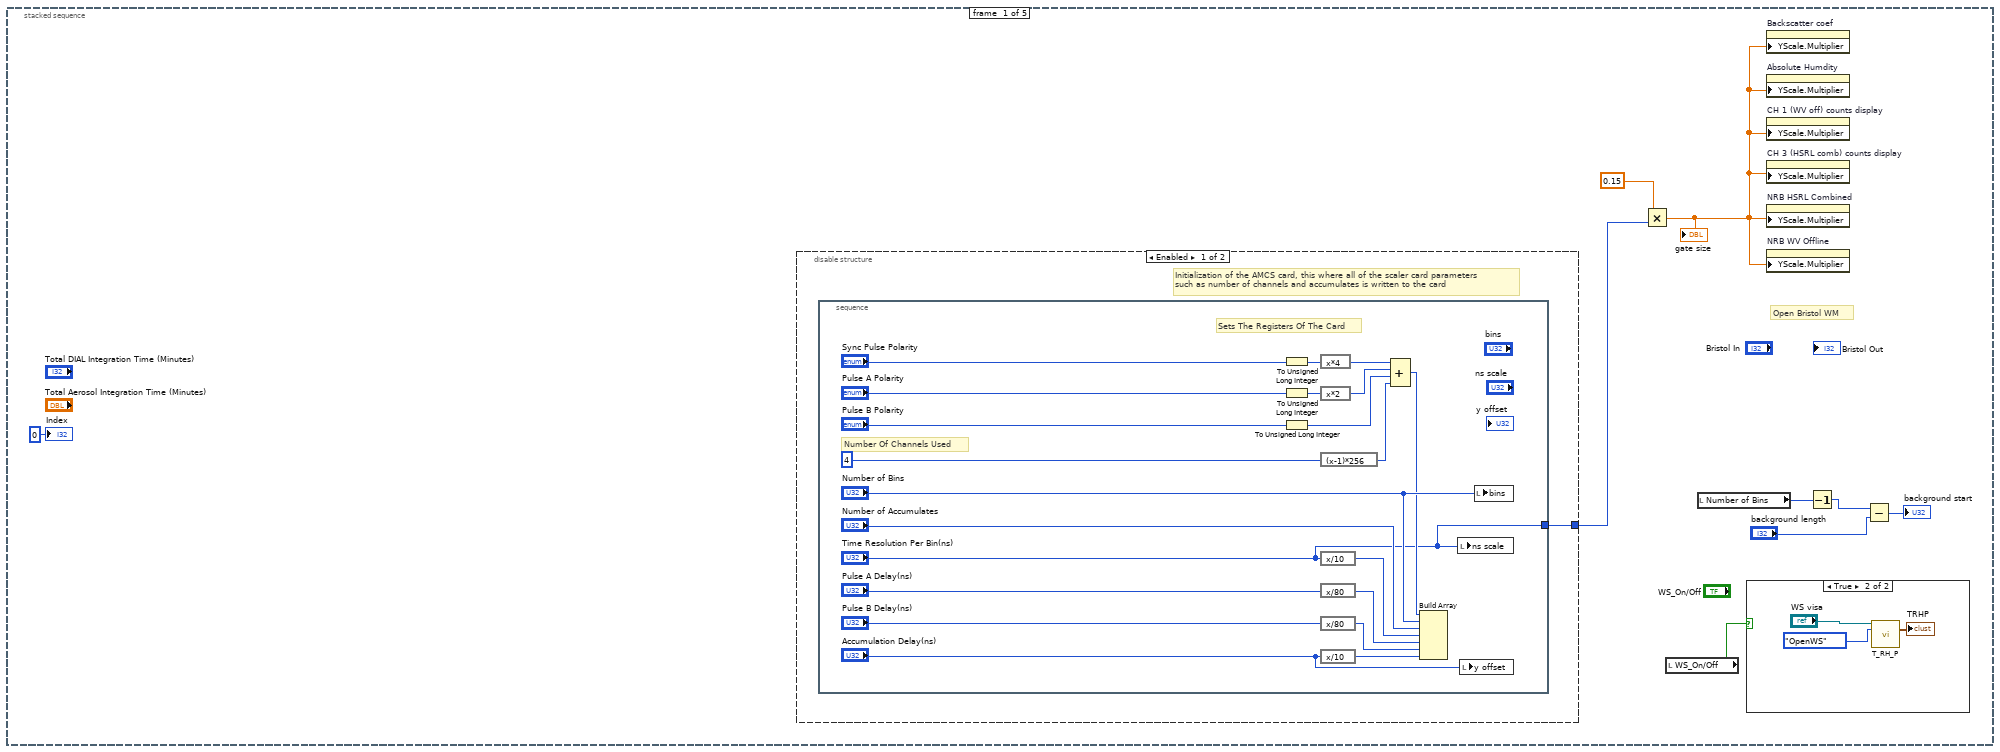
[diagram p4: hidden frame]
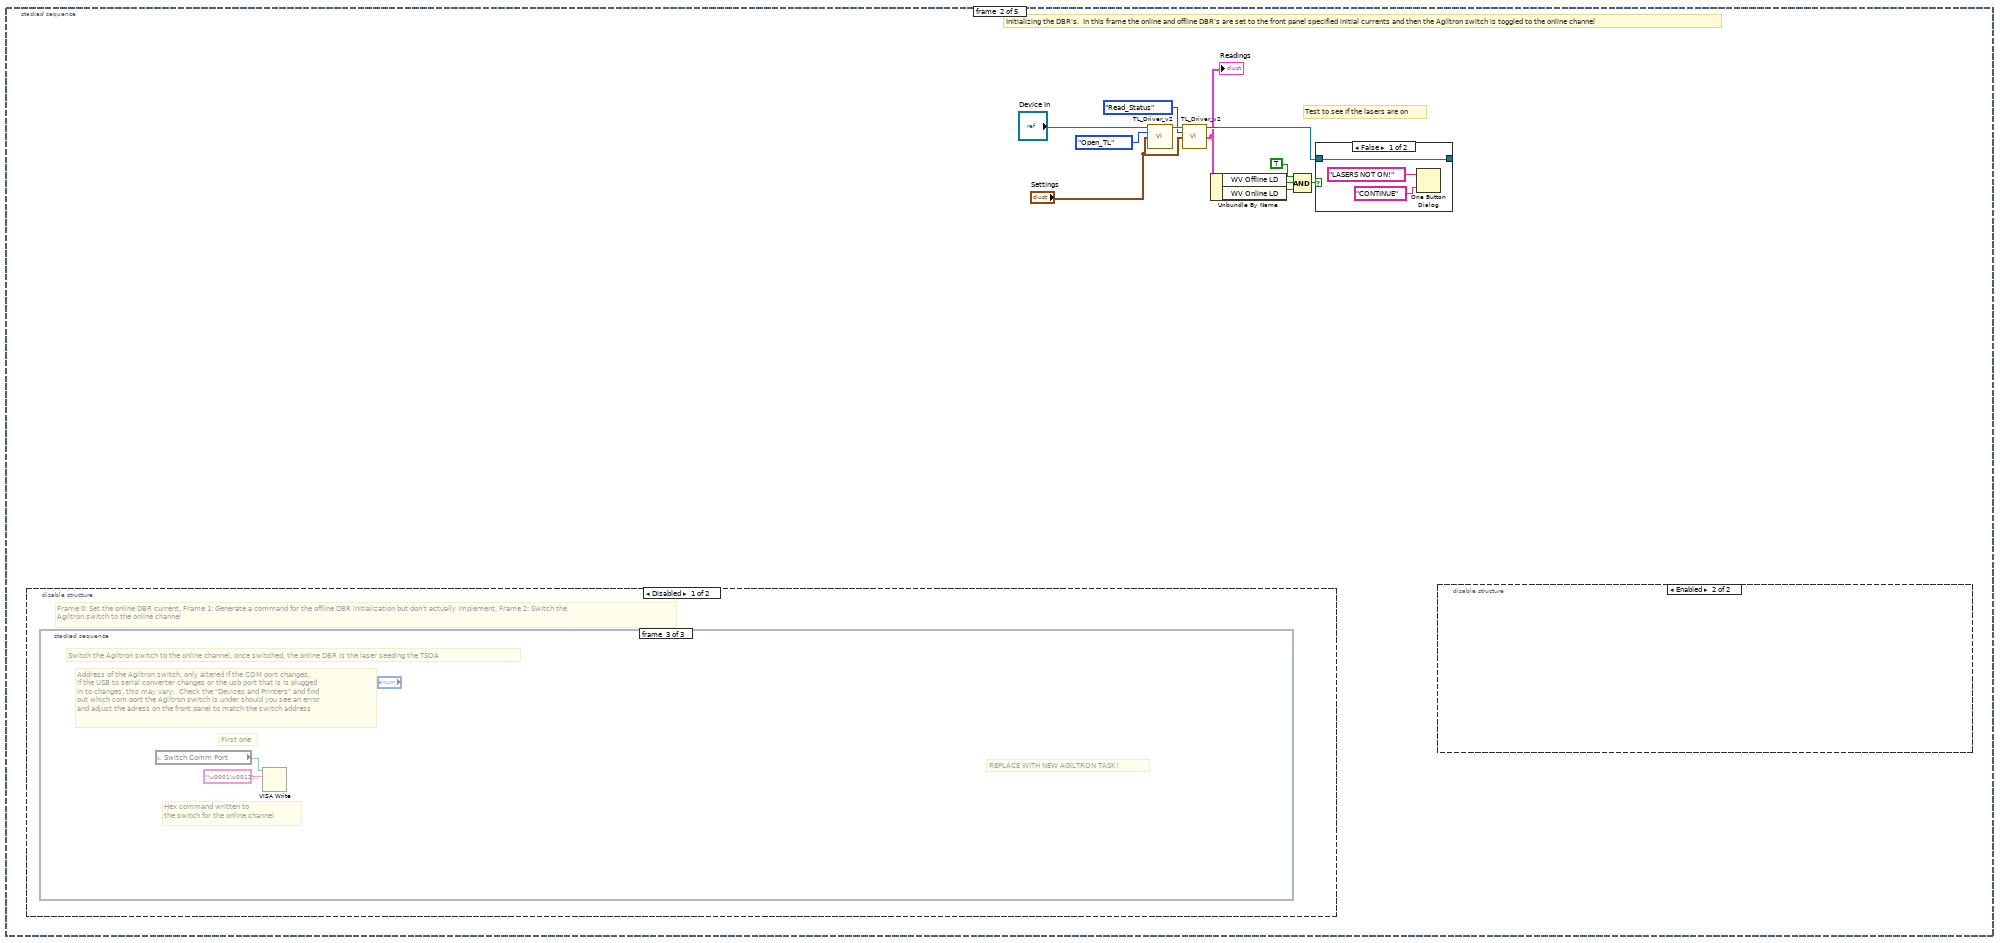
[diagram p7: hidden frame]
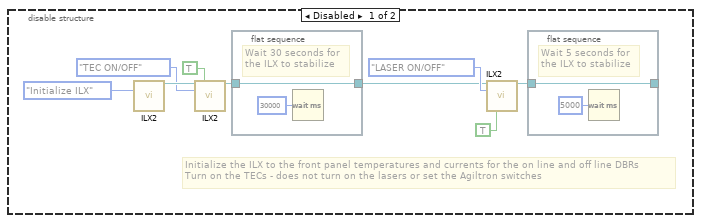
[diagram p9: hidden frame]
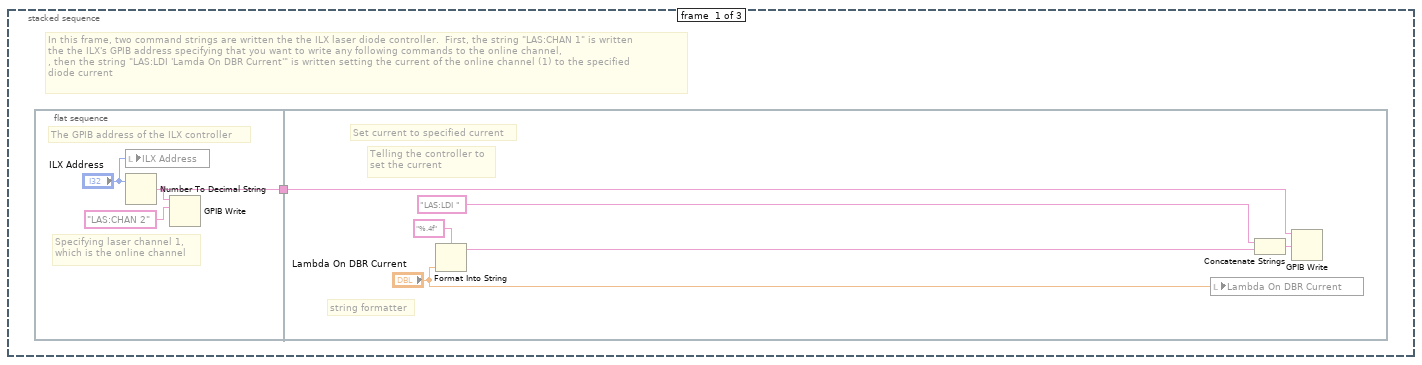
[diagram p10: hidden frame]
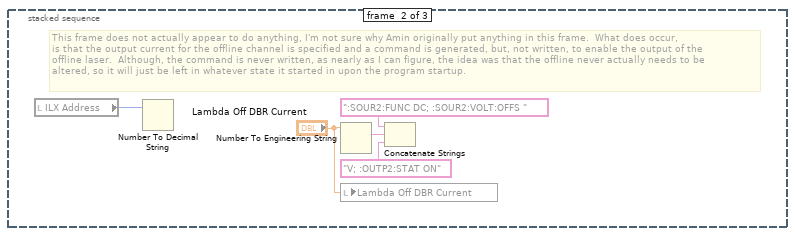
[diagram p11: hidden frame]
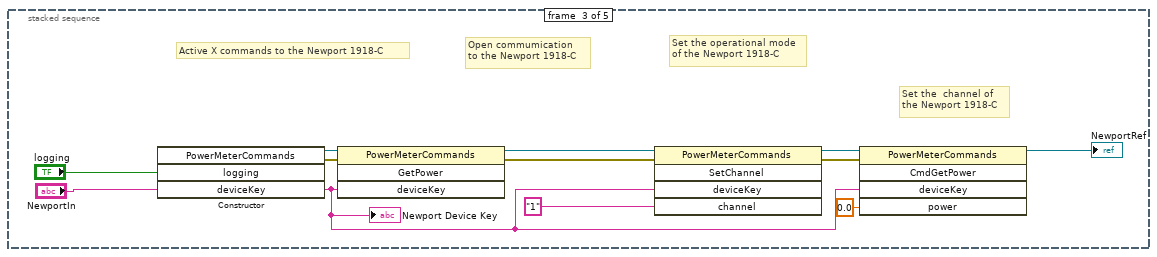
[diagram p13: hidden frame]
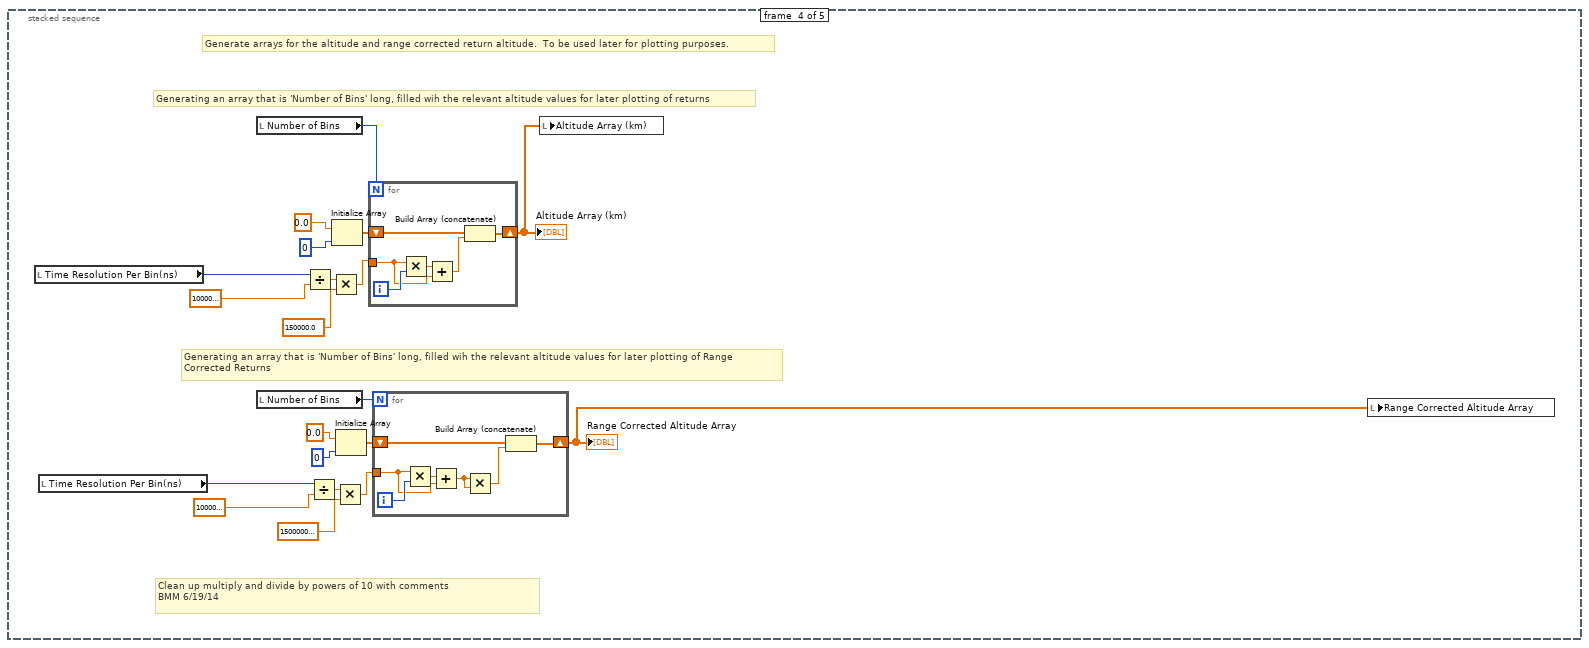
[diagram p14: hidden frame]
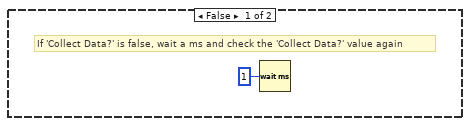
[diagram p15: hidden frame]
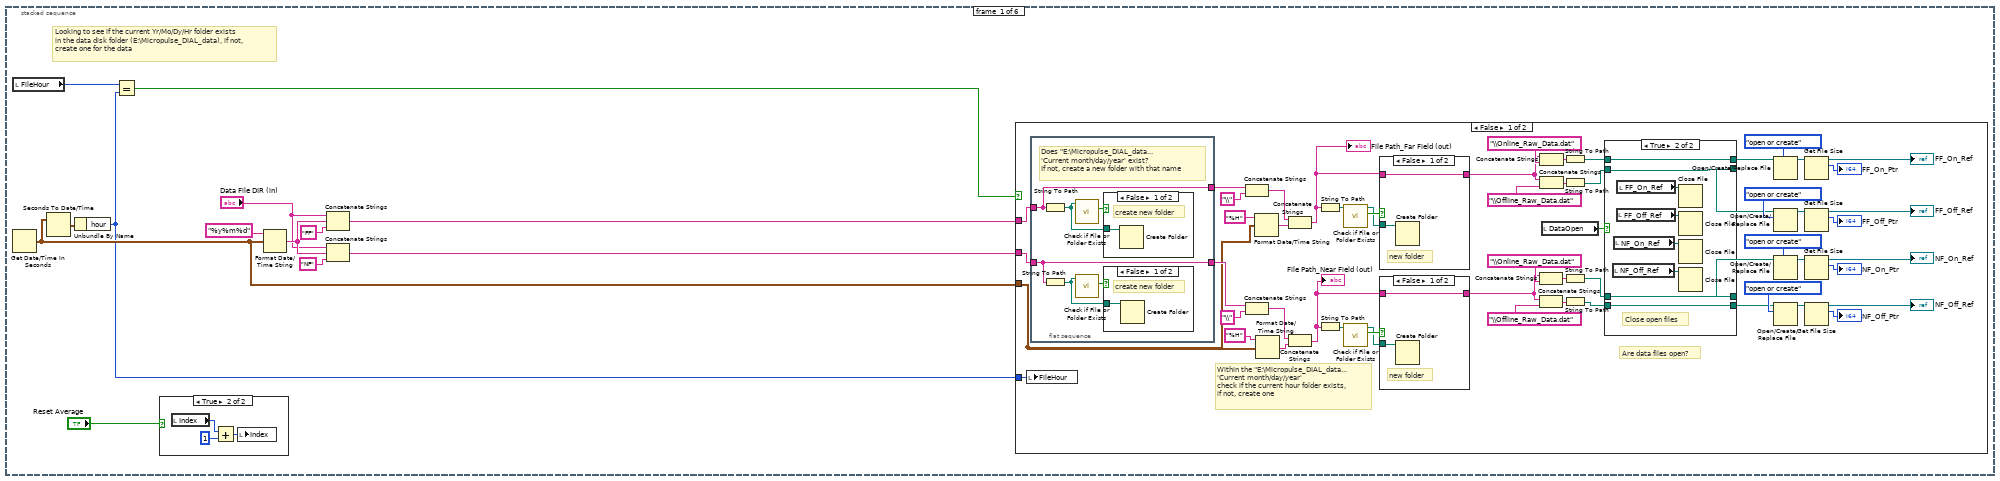
[diagram p16: hidden frame]
diagram:
  # "Frame 0: Initialize the scaler card (and start the MCSC)\nFrame 1: Initialize the DBR's\nFrame 2: Generate address string for talking the to Newport Power meter\nFrame 3: Generate altitude axes for regular and range corrected returns\nFrame 4: Collect data"
  n1 = stacked-sequence {
    tunnel: [_ _ _ _ w128] -> w3
    frame #0 {
      # "Open Bristol WM"
      n2 = disable-structure shown="Enabled" {
        disable-tunnel: [w16 _] -> w5
        frame Enabled {
          # "Initialization of the AMCS card, this where all of the scaler card parameters\nsuch as number of channels and accumulates is written to the card"
          n3 = stacked-sequence {
            tunnel: ["Time Resolution Per Bin(ns)"] -> w16
            frame #0 {
              # "Sets The Registers Of The Card"
              # "Number Of Channels Used"
              n4 = To Unsigned Long Integer(number="Sync Pulse Polarity") -> (unsigned 32bit integer=w18:u32)
              n5 = To Unsigned Long Integer(number="Pulse A Polarity") -> (unsigned 32bit integer=w22:u32)
              n6 = To Unsigned Long Integer(number="Pulse B Polarity") -> (unsigned 32bit integer=w20:u32)
              n7 = expression code="x*4"(w18) -> (w27:u32)
              n8 = expression code="x*2"(w22) -> (w26:u32)
              n9 = expression code="(x-1)*256"(u32 4 ("Number of Channels Used")) -> (w25:u32)
              n10 = expression code="x/10"("Time Resolution Per Bin(ns)") -> (w28:u32)
              n11 = expression code="x/80"("Pulse A Delay(ns)") -> (w35:u32)
              n12 = expression code="x/80"("Pulse B Delay(ns)") -> (w37:u32)
              n13 = expression code="x/10"("Accumulation Delay(ns)") -> (w36:u32)
              n14 = Compound Arithmetic op=ADD(w27, w26, w20, w25) -> (w24:u32)
              n15 = Build Array(w24, "Number of Bins", "Number of Accumulates", w28, w35, w37, w36) -> ()  [unwired: 1 out]
              n16 = local write "ns scale"("Time Resolution Per Bin(ns)") -> ()
              n17 = local write "y offset"("Accumulation Delay(ns)") -> ()
              n18 = local write "bins"("Number of Bins") -> ()
            }
          }
        }
        frame Disabled {
        }
      }
      n19 = Multiply(x=0.15, y=w5) -> (x*y=w4:dbl)
      "gate size" <- w4
      n20 = local read "WS_On/Off"() -> (w7:bool)
      n21 = local read "Number of Bins"() -> (w11:u32)
      n22 = case shown="True" w7 {
        frame False {
        }
        frame True {
          n23 = call "T_RH_P.vi"("VISA in"="WS visa", "WS_Commands"=enum16{"OpenWS", "ReadTRHP", "CloseWS"}."OpenWS") -> ("TRHP"=→"TRHP":T13)  [unwired: 11 in, 2 out]
        }
      }
      n24 = property on="Backscatter coef" class="IntChart (strict)"("YScale.Multiplier"=w4) -> ()  [unwired: 2 in, 2 out]
      n25 = property on="Absolute Humdity" class="IntChart (strict)"("YScale.Multiplier"=w4) -> ()  [unwired: 2 in, 2 out]
      n26 = property on="CH 1 (WV off) counts display" class="IntChart (strict)"("YScale.Multiplier"=w4) -> ()  [unwired: 2 in, 2 out]
      n27 = property on="CH 3 (HSRL comb) counts display" class="IntChart (strict)"("YScale.Multiplier"=w4) -> ()  [unwired: 2 in, 2 out]
      n28 = property on="NRB HSRL Combined" class="IntChart (strict)"("YScale.Multiplier"=w4) -> ()  [unwired: 2 in, 2 out]
      n29 = property on="NRB WV Offline" class="IntChart (strict)"("YScale.Multiplier"=w4) -> ()  [unwired: 2 in, 2 out]
      n30 = Decrement(x=w11) -> (x-1=w10:u32)
      n31 = Subtract(x=w10, y="background length") -> (x-y=→"background start":u32)
      "Index" <- 0 ("Index")
    }
    frame #1 {
      # "Test to see if the lasers are on"
      # "Initializing the DBR's.  In this frame the online and offline DBR's are set to the front panel specified initial currents and then the Agiltron switch is toggled to the online channel"
      n32 = disable-structure shown="Disabled" {
        frame Disabled {
          # "Frame 0: Set the online DBR current, Frame 1: Generate a command for the offline DBR initialization but don't actually implement, Frame 2: Switch the \nAgiltron switch to the online channel"
          n33 = stacked-sequence {
            frame #0 {
              # "In this frame, two command strings are written the the ILX laser diode controller.  First, the string \"LAS:CHAN 1\" is written\nthe the ILX's GPIB address specifying that you want to write any following commands to the online channel,\n, then the string \"LAS:LDI 'Lamda On DBR Current'\" is written setting the current of the online channel (1) to the specified \ndiode current"
              n34 = flat-sequence {
                tunnel: [w68] -> w66
                tunnel: w66 -> [w70]
                frame #0 {
                  # "The GPIB address of the ILX controller"
                  # "Specifying laser channel 1,\nwhich is the online channel"
                  n35 = local write "ILX Address"("ILX Address") -> ()
                  n36 = Number To Decimal String(number="ILX Address") -> (decimal integer string=w68:string)  [unwired: 1 in]
                  n37 = GPIB Write(0:w68, 1:"LAS:CHAN 2") -> ()  [unwired: 3 in, 2 out]
                }
                frame #1 {
                  # "Telling the controller to\nset the current"
                  # "string formatter"
                  # "Set current to specified current"
                  n38 = Format Into String(format string="%.4f" ("Format String"), "Lambda On DBR Current") -> (resulting string=w73:string)  [unwired: 2 in, 1 out]
                  n39 = local write "Lambda On DBR Current"("Lambda On DBR Current") -> ()
                  n40 = Concatenate Strings("LAS:LDI ", w73) -> (w74:string)
                  n41 = GPIB Write(0:w70, 1:w74) -> ()  [unwired: 3 in, 2 out]
                }
              }
            }
            frame #1 {
              # "This frame does not actually appear to do anything, I'm not sure why Amin originally put anything in this frame.  What does occur, \nis that the output current for the offline channel is specified and a command is generated, but, not written, to enable the output of the\noffline laser.  Although, the command is never written, as nearly as I can figure, the idea was that the offline never actually needs to be \naltered, so it will just be left in whatever state it started in upon the program startup."
              n42 = local read "ILX Address"() -> (w76:i32)
              n43 = Number To Decimal String(number=w76) -> ()  [unwired: 1 in, 1 out]
              n44 = Number To Engineering String(4:"Lambda Off DBR Current") -> (0:w80:string)  [unwired: 3 in]
              n45 = local write "Lambda Off DBR Current"("Lambda Off DBR Current") -> ()
              n46 = Concatenate Strings(":SOUR2:FUNC DC; :SOUR2:VOLT:OFFS ", w80, "V; :OUTP2:STAT ON") -> ()  [unwired: 1 out]
            }
            frame #2 {
              # "REPLACE WITH NEW AGILTRON TASK!"
              # "First one"
              # "Address of the Agiltron switch, only altered if the COM port changes,\nif the USB to serial converter changes or the usb port that is is plugged\nin to changes, this may vary.  Check the \"Devices and Printers\" and find \nout which com port the Agiltron switch is under should you see an error \nand adjust the adress on the front panel to match the switch address"
              # "Hex command written to \nthe switch for the online channel"
              # "Switch the Agiltron switch to the online channel, once switched, the online DBR is the laser seeding the TSOA"
              n47 = local read "Switch Comm Port"() -> (w81:refnum<visa-resource-name>)
              n48 = VISA Write(VISA resource name=w81, write buffer="\u0001\u0012\u0000\u0002") -> ()  [unwired: 1 in, 3 out]
            }
          }
        }
        frame Enabled {
        }
      }
      n49 = call "TL_Driver_v2.vi"("Device In"="Device In", "Commands"=T9."Open_TL", "Settings"="Settings") -> ("Device Out"=w46:refnum<visa-resource-name>)  [unwired: 9 in, 3 out]
      n50 = call "TL_Driver_v2.vi"("Device In"=w46, "Commands"=T9."Read_Status", "Settings"="Settings") -> ("Device Out"=w44:refnum<visa-resource-name>, "Readings"=w38:T7)  [unwired: 9 in, 2 out]
      "Readings" <- w38
      n51 = Unbundle By Name(w38) -> ("WV Offline LD"=w41:bool, "WV Online LD"=w42:bool)
      n52 = Compound Arithmetic op=AND(TRUE, w41, w42) -> (w40:bool)
      n53 = case shown="False" w40 {
        tunnel: w44 -> [w49 w52]
        tunnel: [w49 w52] -> _
        frame False {
          n54 = One Button Dialog(message="LASERS NOT ON!", button name ("OK")="CONTINUE") -> ()  [unwired: 1 out]
        }
        frame True {
        }
      }
      n55 = disable-structure shown="Enabled" {
        frame Disabled {
          # "Initialize the ILX to the front panel temperatures and currents for the on line and off line DBRs\nTurn on the TECs - does not turn on the lasers or set the Agiltron switches"
          n56 = call "ILX2.vi"("ILX Command"=T10."Initialize ILX") -> ("Device Out"=w60:refnum<visa-resource-name>)  [unwired: 10 in, 4 out]
          n57 = call "ILX2.vi"("Device In"=w60, "TEC Control"=TRUE, "ILX Command"=T10."TEC ON/OFF") -> ("Device Out"=w57:refnum<visa-resource-name>)  [unwired: 8 in, 4 out]
          n58 = flat-sequence {
            tunnel: w57 -> [w64]
            tunnel: [w64] -> w54
            frame #0 {
              # "Wait 30 seconds for\nthe ILX to stabilize"
              n59 = Wait (ms)(milliseconds to wait=u32 30000) -> ()  [unwired: 1 out]
            }
          }
          n60 = call "ILX2.vi"("Device In"=w54, "ILX Command"=T10."LASER ON/OFF", "Laser Control"=TRUE ("TEC Control")) -> ("Device Out"=w53:refnum<visa-resource-name>)  [unwired: 8 in, 4 out]
          n61 = flat-sequence {
            tunnel: w53 -> [w62]
            tunnel: [w62] -> _
            frame #0 {
              # "Wait 5 seconds for\nthe ILX to stabilize"
              n62 = Wait (ms)(milliseconds to wait=u32 5000) -> ()  [unwired: 1 out]
            }
          }
        }
        frame Enabled {
        }
      }
    }
    frame #2 {
      # "Active X commands to the Newport 1918-C"
      # "Set the  channel of\nthe Newport 1918-C"
      # "Set the operational mode\nof the Newport 1918-C"
      # "Open commumication\nto the Newport 1918-C"
      n63 = constructor class="PowerMeterCommands"("logging"="logging", "deviceKey"="NewportIn") -> (reference out=w94:refnum<k24>, error out=w91:errorcluster, "deviceKey"=w86:string)  [unwired: 3 in, 2 out]
      "Newport Device Key" <- w86
      n64 = invoke class="PowerMeterCommands" method="GetPower"(reference=w94, error in=w91, "deviceKey"=w86) -> (reference out=w93:refnum<k24>, error out=w90:errorcluster)  [unwired: 1 in, 2 out]
      n65 = invoke class="PowerMeterCommands" method="SetChannel"(reference=w93, error in=w90, "deviceKey"=w86, "channel"="1") -> (reference out=w87:refnum<k24>, error out=w89:errorcluster)  [unwired: 1 in, 3 out]
      n66 = invoke class="PowerMeterCommands" method="CmdGetPower"(reference=w87, error in=w89, "deviceKey"=w86, "power"=sgl 0.0) -> (reference out=→"NewportRef":refnum<k24>)  [unwired: 1 in, 4 out]
    }
    frame #3 {
      # "Clean up multiply and divide by powers of 10 with comments\nBMM 6/19/14"
      # "Generating an array that is 'Number of Bins' long, filled wih the relevant altitude values for later plotting of Range \nCorrected Returns"
      # "Generating an array that is 'Number of Bins' long, filled wih the relevant altitude values for later plotting of returns"
      # "Generate arrays for the altitude and range corrected return altitude.  To be used later for plotting purposes."
      n67 = local read "Time Resolution Per Bin(ns)"() -> (w107:u32)
      n68 = local read "Time Resolution Per Bin(ns)"() -> (w97:u32)
      n69 = local read "Number of Bins"() -> (w110:u32)
      n70 = local read "Number of Bins"() -> (w100:u32)
      n71 = Divide(x=w107, y=1000000000.0) -> (x/y=w105:dbl)
      n72 = Divide(x=w97, y=1000000000.0) -> (x/y=w95:dbl)
      n73 = Multiply(x=w105, y=150000.0) -> (x*y=w108:dbl)
      n74 = Initialize Array(0.0, 0) -> (w113:dbl[])
      n75 = Multiply(x=w95, y=150000000.0) -> (x*y=w98:dbl)
      n76 = Initialize Array(0.0, 0) -> (w103:dbl[])
      n77 = for {
        N: w110 -> [_]
        shift-right: [w126] -> w111
        shift-left: w113 -> [w127]
        tunnel: w108 -> [w123]
        i -> [w125]
        n78 = Multiply(x=w123, y=w125) -> (x*y=w124:dbl)
        n79 = Add(x=w124, y=w123) -> (x+y=w122:dbl)
        n80 = Build Array (concatenate)(w127, w122) -> (w126:dbl[])
      }
      "Altitude Array (km)" <- w111
      n81 = for {
        N: w100 -> [_]
        shift-right: [w120] -> w101
        shift-left: w103 -> [w121]
        tunnel: w98 -> [w116]
        i -> [w119]
        n82 = Multiply(x=w116, y=w119) -> (x*y=w117:dbl)
        n83 = Add(x=w117, y=w116) -> (x+y=w115:dbl)
        n84 = Multiply(x=w115, y=w115) -> (x*y=w118:dbl)
        n85 = Build Array (concatenate)(w121, w118) -> (w120:dbl[])
      }
      "Range Corrected Altitude Array" <- w101
      n86 = local write "Altitude Array (km)"(w111) -> ()
      n87 = local write "Range Corrected Altitude Array"(w101) -> ()
    }
    frame #4 {
      # "Frame 4: Collect data from the scaler card and process and file it"
      n88 = while {
        tunnel: ["stop"] -> w128
        i -> [w129]
        stop <- "stop" stop-if-true
        # "While loop continues data collection cycle"
        n89 = case shown="True" "Collect Data?" {
          frame False {
            # "If 'Collect Data?' is false, wait a ms and check the 'Collect Data?' value again"
            n90 = Wait (ms)(milliseconds to wait=u32 1) -> ()  [unwired: 1 out]
          }
          frame True {
            # "Frame 3: Read the offline wavelength and lock if necessary (code not finished), read output power, read offline data, perform calculations and plot/save offline and NRB data, switch to online\nFrame 4: Calculate the absorption cross section (if wavelength, T, or P changed)\nFrame 5: Calculate Water Vapor Number density and plot"
            # "Frame 0: Create folders and file paths for logging the data, initialize averaging index\nFrame 1: Import current pressure and temperature data from COE weather station\nFrame 2: Read the online wavelength and lock if necessary, read online data and output power\n, plot and save online data, switch to offline DBR"
            # "If 'Collect Data?' is true, collect, process, and log data"
            n91 = stacked-sequence {
              frame #0 {
                # "Looking to see if the current Yr/Mo/Dy/Hr folder exists\nin the data disk folder (E:\\Micropulse_DIAL_data), if not,\ncreate one for the data"
                n92 = local read "FileHour"() -> (w142:i32)
                n93 = Get Date/Time In Seconds() -> (seconds since 1Jan1904=w134:timestamp)
                n94 = Seconds To Date/Time(time stamp (now)=w134) -> (date time rec=w144:T14)  [unwired: 1 in]
                n95 = Unbundle By Name(w144) -> ("hour"=w133:i32)
                n96 = Equal?(x=w142, y=w133) -> (x = y?=w143:bool)
                n97 = case shown="True" "Reset Average" {
                  frame False {
                    n98 = local write "Index"(0 ("Index")) -> ()
                  }
                  frame True {
                    n99 = local read "Index"() -> (w232:i32)
                    n100 = Add(x=w232, y=1) -> (x+y=w231:i32)
                    n101 = local write "Index"(w231) -> ()
                  }
                }
                n102 = Format Date/Time String(time format string (%c)="%y%m%d", seconds (now)=w134) -> (date/time string=w138:string)  [unwired: 1 in]
                n103 = Concatenate Strings("Data File DIR (in)", w138, "FF" ("string")) -> (w140:string)
                n104 = Concatenate Strings("Data File DIR (in)", w138, "NF" ("string")) -> (w135:string)
                n105 = case shown="False" w143 {
                  tunnel: w140 -> [w202 _]
                  tunnel: w135 -> [w201 _]
                  tunnel: w134 -> [w188 _]
                  tunnel: w133 -> [w164 _]
                  frame False {
                    # "Are data files open?"
                    # "Within the \"E:\\Micropulse_DIAL_data...\n'Current month/day/year' \ncheck if the current hour folder exists,\nif not, create one"
                    n106 = local write "FileHour"(w164) -> ()
                    n107 = flat-sequence {
                      tunnel: [w222] -> w189
                      tunnel: w202 -> [w221]
                      tunnel: w201 -> [w222]
                      tunnel: [w221] -> w190
                      frame #0 {
                        # "Does \"E:\\Micropulse_DIAL_data...\n'Current month/day/year' exist?\nIf not, create a new folder with that name"
                        n108 = String To Path(string=w221) -> (path=w226:path)
                        n109 = String To Path(string=w222) -> (path=w224:path)
                        n110 = call <vilib>:"Check if File or Folder Exists.vi"("path"=w226) -> ("file or folder exists?"=w225:bool)  [unwired: 8 in, 2 out]
                        n111 = call <vilib>:"Check if File or Folder Exists.vi"("path"=w224) -> ("file or folder exists?"=w223:bool)  [unwired: 8 in, 2 out]
                        n112 = case shown="False" w225 {
                          tunnel: w226 -> [w228 _]
                          frame False {
                            # "create new folder"
                            n113 = Create Folder(path (use dialog)=w228) -> ()  [unwired: 2 in, 3 out]
                          }
                          frame True {
                            # "Folder exists\ndo nothing"
                          }
                        }
                        n114 = case shown="False" w223 {
                          tunnel: w224 -> [w227 _]
                          frame False {
                            # "create new folder"
                            n115 = Create Folder(path (use dialog)=w227) -> ()  [unwired: 2 in, 3 out]
                          }
                          frame True {
                            # "Folder exists\ndo nothing"
                          }
                        }
                      }
                    }
                    n116 = Concatenate Strings(w190, "\\" ("string")) -> (w197:string)
                    n117 = Concatenate Strings(w189, "\\" ("string")) -> (w192:string)
                    n118 = Format Date/Time String(time format string (%c)="%H", seconds (now)=w188) -> (date/time string=w200:string)  [unwired: 1 in]
                    n119 = Format Date/Time String(time format string (%c)="%H", seconds (now)=w188) -> (date/time string=w195:string)  [unwired: 1 in]
                    n120 = Concatenate Strings(w197, w200) -> (w160:string)
                    "File Path_Far Field (out)" <- w160
                    n121 = Concatenate Strings(w192, w195) -> (w161:string)
                    "File Path_Near Field (out)" <- w161
                    n122 = String To Path(string=w160) -> (path=w198:path)
                    n123 = String To Path(string=w161) -> (path=w193:path)
                    n124 = call <vilib>:"Check if File or Folder Exists.vi"("path"=w198) -> ("file or folder exists?"=w187:bool, "dup path"=w185:path)  [unwired: 8 in, 1 out]
                    n125 = call <vilib>:"Check if File or Folder Exists.vi"("path"=w193) -> ("file or folder exists?"=w186:bool, "dup path"=w184:path)  [unwired: 8 in, 1 out]
                    n126 = case shown="False" w187 {
                      tunnel: w185 -> [w219 _]
                      tunnel: w160 -> [w218 w220]
                      tunnel: [w218 w220] -> w158
                      frame False {
                        # "new folder"
                        n127 = Create Folder(path (use dialog)=w219) -> ()  [unwired: 2 in, 3 out]
                      }
                      frame True {
                        # "Folder exists\ndo nothing"
                      }
                    }
                    n128 = case shown="False" w186 {
                      tunnel: w184 -> [w216 _]
                      tunnel: w161 -> [w215 w217]
                      tunnel: [w215 w217] -> w159
                      frame False {
                        # "new folder"
                        n129 = Create Folder(path (use dialog)=w216) -> ()  [unwired: 2 in, 3 out]
                      }
                      frame True {
                        # "Folder exists\ndo nothing"
                      }
                    }
                    n130 = Concatenate Strings(w159, "\\Online_Raw_Data.dat" ("string")) -> (w178:string)
                    n131 = Concatenate Strings(w159, "\\Offline_Raw_Data.dat" ("string")) -> (w177:string)
                    n132 = Concatenate Strings(w158, "\\Online_Raw_Data.dat" ("string")) -> (w183:string)
                    n133 = Concatenate Strings(w158, "\\Offline_Raw_Data.dat" ("string")) -> (w182:string)
                    n134 = local read "DataOpen"() -> (w175:bool)
                    n135 = String To Path(string=w183) -> (path=w174:path)
                    n136 = String To Path(string=w182) -> (path=w173:path)
                    n137 = String To Path(string=w178) -> (path=w172:path)
                    n138 = String To Path(string=w177) -> (path=w171:path)
                    n139 = case shown="True" w175 {
                      tunnel: w174 -> [w206 w210]
                      tunnel: [w206 w210] -> w168
                      tunnel: w173 -> [w205 w209]
                      tunnel: [w205 w209] -> w167
                      tunnel: w172 -> [w204 w208]
                      tunnel: [w204 w208] -> w166
                      tunnel: [w203 w207] -> w165
                      tunnel: w171 -> [w203 w207]
                      frame False {
                        # "No files open\ndo nothing"
                      }
                      frame True {
                        # "Close open files"
                        n140 = local read "NF_Off_Ref"() -> (w212:refnum<file>)
                        n141 = local read "NF_On_Ref"() -> (w211:refnum<file>)
                        n142 = local read "FF_Off_Ref"() -> (w214:refnum<file>)
                        n143 = local read "FF_On_Ref"() -> (w213:refnum<file>)
                        n144 = Close File(refnum=w213) -> ()  [unwired: 1 in, 2 out]
                        n145 = Close File(refnum=w214) -> ()  [unwired: 1 in, 2 out]
                        n146 = Close File(refnum=w211) -> ()  [unwired: 1 in, 2 out]
                        n147 = Close File(refnum=w212) -> ()  [unwired: 1 in, 2 out]
                      }
                    }
                    n148 = Open/Create/Replace File(file path (use dialog)=w168, operation (0:open)=T11."open or create") -> (refnum out=w154:refnum<file>)  [unwired: 4 in, 2 out]
                    n149 = Open/Create/Replace File(file path (use dialog)=w167, operation (0:open)=T11."open or create") -> (refnum out=w155:refnum<file>)  [unwired: 4 in, 2 out]
                    n150 = Open/Create/Replace File(file path (use dialog)=w166, operation (0:open)=T11."open or create") -> (refnum out=w156:refnum<file>)  [unwired: 4 in, 2 out]
                    n151 = Open/Create/Replace File(file path (use dialog)=w165, operation (0:open)=T11."open or create") -> (refnum out=w157:refnum<file>)  [unwired: 4 in, 2 out]
                    n152 = Get File Size(file=w154) -> (refnum out=→"FF_On_Ref":refnum<file>, size (in bytes)=→"FF_On_Ptr":i64)  [unwired: 1 in, 1 out]
                    n153 = Get File Size(file=w155) -> (refnum out=→"FF_Off_Ref":refnum<file>, size (in bytes)=→"FF_Off_Ptr":i64)  [unwired: 1 in, 1 out]
                    n154 = Get File Size(file=w156) -> (refnum out=→"NF_On_Ref":refnum<file>, size (in bytes)=→"NF_On_Ptr":i64)  [unwired: 1 in, 1 out]
                    n155 = Get File Size(file=w157) -> (refnum out=→"NF_Off_Ref":refnum<file>, size (in bytes)=→"NF_Off_Ptr":i64)  [unwired: 1 in, 1 out]
                  }
                  frame True {
                    # "Don't need to do anything!"
                  }
                }
              }
              frame #1 {
                # "Writing and plotting retrieved\nweather parameters"
                # "Matlab script goes online and retrieves most recent press, temp, and relative humidity data \nfrom the weather station on the roof of Cobleigh"
                # "Importing the current weather conditions from the COE weather station"
                n156 = disable-structure shown="Disabled" {
                  frame Disabled {
                    n157 = script code="%try\n%s=urlread('http://www.coe.montana.edu/ee/weather/mostCurrentCSV.php');\n%amin=textscan(s,'%s %s %s %s %s %s %s %s %s %s %s %s %s');\n%data=amin{1}{2};\n%[test remain]=strtok(data,',');\n%remain=str2num(remain);\n%press=remain(3)./1000;\n%temp=remain(5);\n%RH=remain(7);\n%catch\npress=.850;\ntemp=20;\nRH=40;\n%end"() -> ()  [unwired: 1 in, 4 out]
                  }
                  frame Enabled {
                  }
                }
                n158 = local read "WS_On/Off"() -> (w233:bool)
                n159 = case shown="True" w233 {
                  frame False {
                  }
                  frame True {
                    n160 = local read "WS visa"() -> (w238:refnum<visa-resource-name>)
                    n161 = call "T_RH_P.vi"("VISA in"=w238, "WS_Commands"=enum16{"OpenWS", "ReadTRHP", "CloseWS"}."ReadTRHP") -> ("TRHP"=w234:T13)  [unwired: 11 in, 2 out]
                    n162 = local write "TRHP"(w234) -> ()
                    n163 = Unbundle By Name(w234) -> ("Temp"=→"Temperature (C)":dbl, "RelH"=→"Relative Humdity (%)":dbl, "Press"=→"Pressure (mb)":dbl)
                  }
                }
              }
              frame #2 {
                # "Frame 3: Read, process, and plot online data\nFrame 4:\nFrame 5: Write the data to the folders from Frame 0 of outter sequence"
                # "Frame 0: Read the online wavelength and adjust to locking tolerance if out of range, Switch to offline DBR\nFrame 1: Read the output power from the Newport meter, calculate and plot the output pulse energy\nFrame 2: Wait 'Scalar Wait Time' for buffer to clear other wavelength data"
                # "Online"
                n164 = stacked-sequence {
                  frame #0 {
                    # "Read the online wavelength and continue adjusting the online DBR if outside the wavelength tolerance\nuntil it is within tolerance"
                    n165 = while {
                      i -> [w241]
                      stop <- w240 stop-if-true
                      # "Frame 2: Decrement DBR current if above tolerance\nFrame 3: Increment DBR current if below tolerance"
                      # "Frame 0: Read the current wavelength from the wavemeter\nFrame 1: Calculate the difference between desired and actual wavelength"
                      # "Continue reading and adjusting online DBR current until within locking tolerance"
                      n166 = stacked-sequence {
                        tunnel: w241 -> [w243 _ _ _ _]
                        tunnel: [_ _ w259 _ _] -> w240
                        frame #0 {
                          n167 = Equal To 0?(x=w243) -> (x = 0?=w242:bool)
                          n168 = case shown="True" w242 {
                            frame False {
                            }
                            frame True {
                              # "Set the wavemeter switch to WV Online"
                              n169 = flat-sequence {
                                frame #0 {
                                n170 = Build Array(FALSE ("Boolean")) -> (w246:bool[])
                                n171 = call-poly <vilib>:"DAQmx Write.vi"("task/channels in"=refnum<k21> "BristolWM", "data"=w246) -> ()  [unwired: 11 in, 3 out]
                                }
                                frame #1 {
                                n172 = Build Array(FALSE ("Boolean")) -> (w249:bool[])
                                n173 = call-poly <vilib>:"DAQmx Write.vi"("task/channels in"=refnum<k21> "HSRL_WV_switch", "data"=w249) -> ()  [unwired: 11 in, 3 out]
                                }
                              }
                            }
                          }
                        }
                        frame #1 {
                          # "Reading the wavelength from the wavemeter"
                          n174 = flat-sequence {
                            tunnel: [w252] -> w251
                            tunnel: w251 -> [w255]
                            tunnel: [w254] -> w250
                            tunnel: w250 -> [w258]
                            frame #0 {
                              n175 = local read "Bristol In"() -> (w253:i32)
                              n176 = dll-call lib="C:/Users/eol-lidar/Desktop/20171016_WVDIALLabviewSlimmed/DLLs/CLDevIface.dll" fn="CLOpenUSBSerialDevice"("commPort"=w253) -> ("return type"=w252:i32)  [unwired: 4 in, 2 out]
                            }
                            frame #1 {
                              n177 = dll-call lib="C:/Users/eol-lidar/Desktop/20171016_WVDIALLabviewSlimmed/DLLs/CLDevIface.dll" fn="CLGetLambdaReading"("devHandle"=w255) -> ("return type"=→"WV Online Read (nm)":dbl, "devHandle"=w254:i32)  [unwired: 3 in, 2 out]
                            }
                            frame #2 {
                              n178 = dll-call lib="C:/Users/eol-lidar/Desktop/20171016_WVDIALLabviewSlimmed/DLLs/CLDevIface.dll" fn="CLCloseDevice"("commPort"=w258) -> ("return type"=w257:i32)  [unwired: 4 in, 2 out]
                              n179 = local write "Bristol Out"(w257) -> ()
                            }
                          }
                        }
                        frame #2 {
                          # "If WL difference is within tolerance, stop looping, and illuminate 'Wavelength Lock Online' indicator"
                          # "Calculating the difference between the actual and desired online wavelength"
                          n180 = local read "WV Online Read (nm)"() -> (w262:dbl)
                          n181 = local read "Online_Tol"() -> (w267:dbl)
                          n182 = Multiply(x=-1.0, y=w267) -> (x*y=w268:dbl)
                          n183 = Subtract(x=w262, y="WV Online Set (nm)") -> (x-y=w263:dbl)
                          "Online_Diff" <- w263
                          n184 = Greater?(x=w263, y=w268) -> (0:w264:bool)
                          n185 = Less?(x=w263, y=w267) -> (x < y?=w265:bool)
                          n186 = And(x=w264, y=w265) -> (x .and. y?=w261:bool)
                          "WV Online Locked" <- w261
                          n187 = Or(x=w261, y="Cancel online") -> (x .or. y?=w259:bool)
                        }
                        frame #3 {
                          # "If the wavelength difference is greater that 0.0002 nm, decrement the \nDBR current by 0.01 mA"
                          n188 = local read "Online_Diff"() -> (w272:dbl)
                          n189 = Greater Or Equal?(x=w272, y="Online_Tol") -> (x >= y?=w271:bool)
                          n190 = case shown="True" w271 {
                            frame False {
                              # "Wavelength difference is not greater than 0.0002 nm, do nothing"
                            }
                            frame True {
                              # "Generating a command string\nto decrement the current"
                              # "WL difference is greater than 0.0002 nm,\ndecrement the DBR current by 0.01 mA"
                              n191 = local read "Settings"() -> (w279:T6)
                              n192 = local read "temp step size"() -> (w274:dbl)
                              n193 = Unbundle By Name(w279) -> ("WV Online TEC"=w278:dbl)
                              n194 = local read "Device In"() -> (w275:refnum<visa-resource-name>)
                              n195 = Subtract(x=w278, y=w274) -> (x-y=w277:dbl)
                              n196 = Bundle By Name(cluster=w279, "WV Online TEC"=w277, "Module"=T12."WV Online TEC") -> (w281:T6)
                              n197 = call "TL_Driver_v2.vi"("Device In"=w275, "Commands"=T9."SET", "Settings"=w281) -> ("Readings"=w280:T7)  [unwired: 9 in, 3 out]
                              n198 = local write "Settings"(w281) -> ()
                              n199 = local write "Readings"(w280) -> ()
                            }
                          }
                        }
                        frame #4 {
                          # "If WL difference is < 0.0002 nm, increment the DBR current"
                          n200 = local read "Online_Tol"() -> (w283:dbl)
                          n201 = local read "Online_Diff"() -> (w286:dbl)
                          n202 = Multiply(x=-1.0, y=w283) -> (x*y=w282:dbl)
                          n203 = Less Or Equal?(x=w286, y=w282) -> (x <= y?=w285:bool)
                          n204 = case shown="True" w285 {
                            frame False {
                              # "WL difference is no <= to -0.0002 nm, do nothing"
                            }
                            frame True {
                              # "WL difference is < -0.0002,\nincrement the DBR current by 0.01 mA"
                              # "Generating a command string\nto decrement the current"
                              n205 = local read "Settings"() -> (w295:T6)
                              n206 = local read "temp step size"() -> (w288:dbl)
                              n207 = Unbundle By Name(w295) -> ("WV Online TEC"=w292:dbl)
                              n208 = local read "Device In"() -> (w289:refnum<visa-resource-name>)
                              n209 = Add(x=w292, y=w288) -> (x+y=w291:dbl)
                              n210 = Bundle By Name(cluster=w295, "WV Online TEC"=w291, "Module"=T12."WV Online TEC") -> (w294:T6)
                              n211 = call "TL_Driver_v2.vi"("Device In"=w289, "Commands"=T9."SET", "Settings"=w294) -> ("Readings"=w293:T7)  [unwired: 9 in, 3 out]
                              n212 = local write "Settings"(w294) -> ()
                              n213 = local write "Readings"(w293) -> ()
                            }
                          }
                        }
                      }
                    }
                  }
                  frame #1 {
                    # "Converting to pulse energy, assumes 5 percent pickoff"
                    # "Reading the Newport Power meter"
                    # "Reading the output power of the laser transmitter from the Newport power meter, once read, convert to corresponding pulse energy and plot"
                    n214 = local read "Newport Device Key"() -> (w304:string)
                    n215 = local read "NewportRef"() -> (w300:refnum<k24>)
                    n216 = disable-structure shown="Enabled" {
                      frame Enabled {
                        # "Plotting the online and offling pulse energies"
                        n217 = local read "WV Online Pulse Energy"() -> (w316:dbl)
                        n218 = local read "WV Offline Pulse Energy"() -> (w312:dbl)
                        n219 = local read "HSRL Pulse Energy"() -> (w315:dbl)
                        n220 = local read "WV_averaged_energy"() -> (w313:dbl)
                        n221 = Bundle("WV Online Pulse Energy"=w316, "WV Offline Pulse Energy"=w312, "HSRL Pulse Energy"=w315, "WV_averaged_energy"=w313) -> (→"Pulse Energy (Micro Joule)":T15)  [unwired: 1 in]
                      }
                      frame Disabled {
                      }
                    }
                    n222 = Number To Decimal String(number="SampleSize") -> (decimal integer string=w302:string)  [unwired: 1 in]
                    n223 = invoke class="PowerMeterCommands" method="PerformDAQ"(reference=w300, "deviceKey"=w304, "interval"="1", "sampleSize"=w302) -> ("PerformDAQ"=w305:dbl[])  [unwired: 2 in, 5 out]
                    n224 = call-poly <vilib>:"Mean.vi"("X"=w305) -> ("mean"=w303:dbl)  [unwired: 1 out]
                    n225 = Multiply(x=w303, y=1000.0) -> (x*y=w310:dbl)
                    n226 = Divide(x=w310, y=0.05) -> (x/y=w308:dbl)
                    n227 = global read "AMCS_Data.vi" "AMCS_PowerMon"() -> (w298:u32[])
                    n228 = Divide(x=w308, y=7.0) -> (x/y=→"WV_averaged_energy":dbl)
                    n229 = Index Array(array=w298, index=6) -> (element=→"WV Online Pulse Energy":u32)
                  }
                  frame #2 {
                    # "Wait 'Scalar Wait Time' for the next available batch of scalar card data"
                    n230 = local read "AMCS_Profile"() -> (w317:i32)
                    n231 = disable-structure shown="Disabled" {
                      frame Disabled {
                        # "Waiting 'Scalar Wait Time'"
                        n232 = Wait (ms)(milliseconds to wait="Scalar Wait Time") -> ()  [unwired: 1 out]
                      }
                      frame Enabled {
                      }
                    }
                    n233 = while {
                      tunnel: [w324] -> w318
                      tunnel: [w320] -> _
                      tunnel: w317 -> [w320]
                      stop <- w322 stop-if-true
                      n234 = global read "AMCS_Data.vi" "AMCS_Profile"() -> (w324:i32)
                      n235 = Wait (ms)(milliseconds to wait=u32 10) -> ()  [unwired: 1 out]
                      n236 = Equal?(x=w324, y=w320) -> (x = y?=w323:bool)
                      n237 = case shown="False" w323 {
                        tunnel: [TRUE FALSE] -> w322
                        frame False {
                        }
                        frame True {
                        }
                      }
                    }
                    "AMCS_Profile" <- w318
                  }
                  frame #3 {
                    # "convert time per range bin to meters\nand calculate smoothed bins using\nsmoothing range"
                    # "Plotting online cross section and smoothed online data"
                    # "Calculate the bin by bin mean of the data"
                    # "Collect 'Integration Period (Seconds)' number\nof scalar data"
                    # "Reading, processing, and plotting the online data"
                    n238 = local read "Data Reads (number of loops)"() -> (w328:i32)
                    n239 = local read "bins"() -> (w327:u32)
                    n240 = for {
                      N: w328 -> [_]
                      tunnel: [w382] -> w368 mode=indexing
                      tunnel: [w377] -> w333 mode=indexing
                      tunnel: w327 -> [w376]
                      # "Scalar Data is retrieved from Global \nVariable that scaler.vi is writing to,"
                      n241 = global read "AMCS_Data.vi" "AMCS_Data"() -> (w385:u16[][])
                      n242 = disable-structure shown="Disabled" {
                        frame Disabled {
                          n243 = global read "Scalar_Data_3.vi" "Scalar Data 3"() -> ()  [unwired: 1 out]
                          n244 = global read "Scalar_Data.vi" "Scalar Data"() -> ()  [unwired: 1 out]
                        }
                        frame Enabled {
                        }
                      }
                      n245 = Index Array(array=w385, index (row) #1=0 ("index (row)"), index (row) #2=2 ("index (row)")) -> (element #1=w381:u16[], element #2=w379:u16[])  [unwired: 2 in]
                      n246 = Array Subset(array=w381, index=0, length=w376) -> (w382:u16[])
                      n247 = Array Subset(array=w379, index=0, length=w376) -> (w377:u16[])
                    }
                    n248 = Transpose 2D Array(2D array=w368) -> (transposed array=w372:u16[][])
                    n249 = Transpose 2D Array(2D array=w333) -> (transposed array=w355:u16[][])
                    n250 = for {
                      tunnel: w355 -> [w375] mode=indexing
                      tunnel: [w374] -> w356 mode=indexing
                      n251 = call-poly <vilib>:"Mean.vi"("X"=w375) -> ("mean"=w374:dbl)  [unwired: 1 out]
                    }
                    n252 = for {
                      tunnel: w372 -> [w387] mode=indexing
                      tunnel: [w386] -> w373 mode=indexing
                      n253 = call-poly <vilib>:"Mean.vi"("X"=w387) -> ("mean"=w386:dbl)  [unwired: 1 out]
                    }
                    n254 = Array Subset(array=w373, index=1 ("dimension size"), length=w327) -> (w360:dbl[])
                    n255 = Array Subset(array=w356, index=1 ("dimension size"), length=w327) -> (w353:dbl[])
                    n256 = local read "background length"() -> (w340:i32)
                    n257 = local read "background start"() -> (w341:u32)
                    n258 = Array Size(array=w360) -> (size(s)=w357:i32)
                    n259 = Array Size(array=w353) -> (size(s)=w350:i32)
                    n260 = Initialize Array(1.0 ("element"), w357) -> (w359:dbl[])
                    n261 = Initialize Array(1.0 ("element"), w350) -> (w352:dbl[])
                    n262 = Multiply(x=w360, y=w359) -> (x*y=w361:dbl[])
                    "CH 0 Bin Readings" <- w361
                    n263 = Multiply(x=w353, y=w352) -> (x*y=w344:dbl[])
                    "CH 2 Bin Readings" <- w344
                    n264 = local read "Total DIAL Integration Time (Minutes)"() -> (w364:i32)
                    n265 = local read "Total Aerosol Integration Time (Minutes)"() -> (w330:dbl)
                    n266 = local read "Time Resolution Per Bin(ns)"() -> (w336:u32)
                    n267 = Array Subset(array=w361, index=w341, length=w340) -> (w370:dbl[])
                    n268 = Array Subset(array=w344, index=w341, length=w340) -> (w346:dbl[])
                    n269 = Divide(x=w330, y=w328) -> (x/y=w331:dbl)
                    n270 = call-poly <vilib>:"Mean.vi"("X"=w370) -> ("mean"=w369:dbl)  [unwired: 1 out]
                    n271 = Multiply(x=w331, y=60.0) -> (x*y=w329:dbl)
                    n272 = call-poly <vilib>:"Mean.vi"("X"=w346) -> ("mean"=w347:dbl)  [unwired: 1 out]
                    n273 = Divide(x=w364, y=w328) -> (x/y=w362:dbl)
                    n274 = local read "Index"() -> (w345:i32)
                    n275 = Subtract(x=w361, y=w369) -> (x-y=w366:dbl[])
                    n276 = Subtract(x=w344, y=w347) -> (x-y=w348:dbl[])
                    n277 = Multiply(x=w362, y=60.0) -> (x*y=w342:dbl)
                    n278 = To Double Precision Float(number=w336) -> (double precision float=w337:dbl)
                    n279 = Multiply(x=w337, y=0.15) -> (x*y=w339:dbl)
                    n280 = call "Ring Buffer CH2 rev2.vi"("Index"=w345, "Profiles to Average"=w329, "Input Array"=w348) -> ("AvgArray"=w349:dbl[])  [unwired: 7 in, 1 out]
                    n281 = call "Ring Buffer CH0 rev2.vi"("Index"=w345, "Profiles to Average"=w342, "Input Array"=w366) -> ("AvgArray"=w365:dbl[])  [unwired: 7 in, 1 out]
                    n282 = Divide(x="Smoothing Range", y=w339) -> (x/y=w334:dbl)
                    "Smoothed Bins" <- w334
                    n283 = call "Smooth Arrray.vi"("smooth size"=w334, "Raw Array"=w365) -> ("Smoothed Array"=→"CH0 (WV on) smoothed":dbl[])  [unwired: 9 in]
                    n284 = call "Smooth Arrray.vi"("smooth size"=w334, "Raw Array"=w349) -> ("Smoothed Array"=→"CH2 (molecular) smoothed":dbl[])  [unwired: 9 in]
                    n285 = disable-structure shown="Disabled" {
                      frame Disabled {
                        n286 = script code="format long;\ncounts=sum(Online);\nif counts >=0.5e6\ntime=time;\nelse\ntime=time\nend"() -> ()  [unwired: 3 in, 2 out]
                      }
                      frame Enabled {
                      }
                    }
                  }
                  frame #4 {
                    # "Toggling the Agiltron switch to the offline DBR seed laser"
                    n287 = disable-structure shown="Disabled" {
                      frame Disabled {
                        n288 = flat-sequence {
                          frame #0 {
                            # "Second one"
                            # "Command the switch to switch to position 2\ncorresponding to the offline DBR"
                            # "Hex string command \ncorrespond to offline"
                            n289 = VISA Write(VISA resource name="Switch Comm Port", write buffer="\u0001\u0012\u0000\u0001") -> ()  [unwired: 1 in, 3 out]
                          }
                        }
                      }
                      frame Enabled {
                      }
                    }
                  }
                  frame #5 {
                    # "Save the recently collected online data if 'Save Data?' is true"
                    n290 = case shown="True" "Save Data?" {
                      frame False {
                        # "'Save Data?' is false, do nothing"
                      }
                      frame True {
                        # "'Save Data?' is true, save onfline data to the Data Disk"
                        # "Write only one copy of data at this time"
                        # "Retrieve Julian Date"
                        n291 = local read "Readings"() -> (w394:T7)
                        n292 = local read "Time Resolution Per Bin(ns)"() -> (w402:u32)
                        n293 = Unbundle By Name(w394) -> ("WV OnLine TEC"=w393:dbl)
                        n294 = local read "Number of Accumulates"() -> (w400:u32)
                        n295 = Unbundle By Name(w394) -> ("HSRL TEC"=w392:dbl)
                        n296 = local read "WV Online Read (nm)"() -> (w395:dbl)
                        n297 = local write "DataOpen"(TRUE ("DataOpen")) -> ()
                        n298 = local read "Number of Bins"() -> (w401:u32)
                        n299 = local read "WV_averaged_energy"() -> (w391:dbl)
                        n300 = local read "HSRL Read (nm)"() -> (w396:dbl)
                        n301 = local read "WV Online Pulse Energy"() -> (w423:dbl)
                        n302 = local read "CH 0 Bin Readings"() -> (w425:dbl[])
                        n303 = To Double Precision Float(number=w402) -> (double precision float=w397:dbl)
                        n304 = To Double Precision Float(number=w401) -> (double precision float=w398:dbl)
                        n305 = To Double Precision Float(number=w400) -> (double precision float=w399:dbl)
                        n306 = local read "CH 2 Bin Readings"() -> (w422:dbl[])
                        n307 = call "Julian_Date_2.vi"() -> ("Julian Date"=w424:dbl)  [unwired: 11 in]
                        n308 = Build Array (concatenate)(w424, w395, w393, w423, w397, w398, w399, w425) -> (w417:dbl[])
                        n309 = Build Array (concatenate)(w424, w396, w392, w391, w397, w398, w399, w422) -> (w407:dbl[])
                        n310 = local read "NF_On_Ref"() -> (w405:refnum<file>)
                        n311 = local read "FF_On_Ref"() -> (w421:refnum<file>)
                        n312 = local read "NF_On_Ptr"() -> (w406:i64)
                        n313 = local read "FF_On_Ptr"() -> (w420:i64)
                        n314 = Set File Position(offset (in bytes) (0)=w420, refnum=w421) -> (refnum out=w418:refnum<file>, error out=w415:errorcluster)  [unwired: 2 in]
                        n315 = Set File Position(offset (in bytes) (0)=w406, refnum=w405) -> (refnum out=w411:refnum<file>, error out=w409:errorcluster)  [unwired: 2 in]
                        n316 = Write to Binary File(file (use dialog)=w411, data=w407, error in=w409, 5:FALSE ("prepend array or string size? (T)")) -> (refnum out=w410:refnum<file>, error out=w408:errorcluster)  [unwired: 2 in, 1 out]
                        n317 = Write to Binary File(file (use dialog)=w418, data=w417, error in=w415, 5:FALSE ("prepend array or string size? (T)")) -> (refnum out=w416:refnum<file>, error out=w414:errorcluster)  [unwired: 2 in, 1 out]
                        n318 = Get File Position(4:w408, 7:w410) -> (2:w404:i64)  [unwired: 2 out]
                        n319 = Get File Position(4:w414, 7:w416) -> (2:w413:i64)  [unwired: 2 out]
                        n320 = local write "NF_On_Ptr"(w404) -> ()
                        n321 = local write "FF_On_Ptr"(w413) -> ()
                      }
                    }
                  }
                }
              }
              frame #3 {
                # "Frame 3: Read offline data, calculate aerosol data, and plot offline and normalized relative backscatter\nFrame 4:\nFrame 5: Save the offline data and related information"
                # "Frame 0: Read the offline wavelength and lock if necessary, Switch to online DBR\nFrame 1: Read the output power from the Newport power meter\nFrame 2: Wait 'Scalar Wait Time' for buffers to clear of online contiminated data"
                # "offline"
                n322 = stacked-sequence {
                  frame #0 {
                    # "Following Locking the Offline wavelength, check and lock the HSRL 780 nm wavelength"
                    # "Every 60 data collection cycles, read the offline DBR wavelength, and if outside of wavelength tolerance, adjust DBR current until within tolerance"
                    n323 = local read "L_Count"() -> (w427:i32)
                    n324 = Quotient & Remainder(x=w427, y=60.0) -> (x-y*floor(x/y)=w428:dbl)  [unwired: 1 out]
                    n325 = Equal To 0?(x=w428) -> (x = 0?=w426:bool)
                    n326 = case shown="True" w426 {
                      frame False {
                      }
                      frame True {
                        n327 = flat-sequence {
                          frame #0 {
                            n328 = while {
                              i -> [w433]
                              stop <- w431 stop-if-true
                              # "If WL difference is within tolerance, stop looping, and illuminate 'Wavelength Lock Offline' indicator"
                              # "Frame 2: Decrement DBR if above tolerance\nFrame 3: Increment DBR if below tolerance"
                              # "Frame 0: Read the wavelength from the wavemeter\nFrame 1: Calculate the difference between desired and actual wavelength"
                              # "Continue reading and adjusting offline DBR until within locking tolerance"
                              n329 = stacked-sequence {
                                tunnel: w433 -> [w435 _ _ _ _]
                                tunnel: [_ _ w449 _ _] -> w430
                                frame #0 {
                                n330 = Equal To 0?(x=w435) -> (x = 0?=w434:bool)
                                n331 = case shown="True" w434 {
                                frame False {
                                }
                                frame True {
                                # "Set the TSOA switch to\namplify the offline wavelength"
                                n332 = Build Array(TRUE ("Boolean")) -> (w437:bool[])
                                n333 = call-poly <vilib>:"DAQmx Write.vi"("task/channels in"=refnum<k21> "BristolWM", "data"=w437) -> ()  [unwired: 11 in, 3 out]
                                n334 = Wait (ms)(milliseconds to wait=u32 3200) -> ()  [unwired: 1 out]
                                }
                                }
                                }
                                frame #1 {
                                # "Reading the wavelength from the wavemeter"
                                n335 = flat-sequence {
                                tunnel: [w442] -> w441
                                tunnel: w441 -> [w445]
                                tunnel: [w444] -> w440
                                tunnel: w440 -> [w448]
                                frame #0 {
                                n336 = local read "Bristol In"() -> (w443:i32)
                                n337 = dll-call lib="C:/Users/eol-lidar/Desktop/20171016_WVDIALLabviewSlimmed/DLLs/CLDevIface.dll" fn="CLOpenUSBSerialDevice"("commPort"=w443) -> ("return type"=w442:i32)  [unwired: 4 in, 2 out]
                                }
                                frame #1 {
                                n338 = dll-call lib="C:/Users/eol-lidar/Desktop/20171016_WVDIALLabviewSlimmed/DLLs/CLDevIface.dll" fn="CLGetLambdaReading"("devHandle"=w445) -> ("return type"=→"WV Offline Read (nm)":dbl, "devHandle"=w444:i32)  [unwired: 3 in, 2 out]
                                }
                                frame #2 {
                                n339 = dll-call lib="C:/Users/eol-lidar/Desktop/20171016_WVDIALLabviewSlimmed/DLLs/CLDevIface.dll" fn="CLCloseDevice"("commPort"=w448) -> ("return type"=w447:i32)  [unwired: 4 in, 2 out]
                                n340 = local write "Bristol Out"(w447) -> ()
                                }
                                }
                                }
                                frame #2 {
                                # "Calculating the difference between the actual and desired online wavelength"
                                n341 = local read "Offline_Tol"() -> (w451:dbl)
                                n342 = local read "WV Offline Read (nm)"() -> (w457:dbl)
                                n343 = Multiply(x=-1.0, y=w451) -> (x*y=w450:dbl)
                                n344 = Subtract(x=w457, y="WV Offline Set (nm)") -> (x-y=w453:dbl)
                                "Oflline_Diff" <- w453
                                n345 = Greater?(x=w453, y=w450) -> (0:w454:bool)
                                n346 = Less?(x=w453, y=w451) -> (x < y?=w455:bool)
                                n347 = And(x=w454, y=w455) -> (x .and. y?=w449:bool)
                                "WV Oflline Locked" <- w449
                                n348 = case shown="True" w449 {
                                frame False {
                                }
                                frame True {
                                # "Set the Wavemeter switch to\nthe HSRL wavelength"
                                n349 = Build Array(TRUE ("Boolean")) -> (w459:bool[])
                                n350 = call-poly <vilib>:"DAQmx Write.vi"("task/channels in"=refnum<k21> "HSRL_WV_switch", "data"=w459) -> ()  [unwired: 11 in, 3 out]
                                n351 = Wait (ms)(milliseconds to wait=u32 3200) -> ()  [unwired: 1 out]
                                }
                                }
                                }
                                frame #3 {
                                # "If the wavelength difference is greater that 0.0002 nm, decrement the \nDBR current by 0.01 mA"
                                n352 = local read "Oflline_Diff"() -> (w464:dbl)
                                n353 = Greater Or Equal?(x=w464, y="Offline_Tol") -> (x >= y?=w463:bool)
                                n354 = case shown="True" w463 {
                                frame False {
                                # "Wavelength difference is not greater than 0.0002 nm, do nothing"
                                }
                                frame True {
                                # "Generating a command string\nto decrement the current"
                                n355 = local read "Settings"() -> (w471:T6)
                                n356 = Unbundle By Name(w471) -> ("WV Offline TEC"=w469:dbl)
                                n357 = Subtract(x=w469, y="temp step size") -> (x-y=w468:dbl)
                                n358 = local read "Device In"() -> (w466:refnum<visa-resource-name>)
                                n359 = Bundle By Name(cluster=w471, "WV Offline TEC"=w468, "Module"=T12."WV Offline TEC") -> (w472:T6)
                                n360 = call "TL_Driver_v2.vi"("Device In"=w466, "Commands"=T9."SET", "Settings"=w472) -> ("Readings"=w473:T7)  [unwired: 9 in, 3 out]
                                n361 = local write "Settings"(w472) -> ()
                                n362 = local write "Readings"(w473) -> ()
                                }
                                }
                                }
                                frame #4 {
                                # "If WL difference is < 0.0002 nm, increment the DBR temperature"
                                n363 = local read "Oflline_Diff"() -> (w476:dbl)
                                n364 = Less Or Equal?(x=w476, y=-0.0001) -> (x <= y?=w474:bool)
                                n365 = case shown="True" w474 {
                                frame False {
                                # "WL difference is no <= to -0.0002 nm, do nothing"
                                }
                                frame True {
                                # "Generating a command string\nto decrement the current"
                                # "WL difference is less than 0.0002 nm,\nincrement the DBR current by 0.01 mA"
                                n366 = local read "Settings"() -> (w484:T6)
                                n367 = Unbundle By Name(w484) -> ("WV Offline TEC"=w482:dbl)
                                n368 = local read "temp step size"() -> (w478:dbl)
                                n369 = Add(x=w482, y=w478) -> (x+y=w481:dbl)
                                n370 = local read "Device In"() -> (w479:refnum<visa-resource-name>)
                                n371 = Bundle By Name(cluster=w484, "WV Offline TEC"=w481, "Module"=T12."WV Offline TEC") -> (w485:T6)
                                n372 = call "TL_Driver_v2.vi"("Device In"=w479, "Commands"=T9."SET", "Settings"=w485) -> ("Readings"=w483:T7)  [unwired: 9 in, 3 out]
                                n373 = local write "Settings"(w485) -> ()
                                n374 = local write "Readings"(w483) -> ()
                                }
                                }
                                }
                              }
                              n375 = Or(x=w430, y="Cancel Offline") -> (x .or. y?=w431:bool)
                            }
                          }
                          frame #1 {
                            n376 = while {
                              i -> [w489]
                              stop <- w487 stop-if-true
                              # "If WL difference is within tolerance, stop looping, and illuminate 'Wavelength Lock Offline' indicator"
                              # "Frame 2: Decrement DBR if above tolerance\nFrame 3: Increment DBR if below tolerance"
                              # "Frame 0: Read the wavelength from the wavemeter\nFrame 1: Calculate the difference between desired and actual wavelength"
                              # "Continue reading and adjusting offline DBR until within locking tolerance"
                              n377 = stacked-sequence {
                                tunnel: w489 -> [w491 _ _ _ _]
                                tunnel: [_ _ w504 _ _] -> w486
                                frame #0 {
                                n378 = Equal To 0?(x=w491) -> (x = 0?=w490:bool)
                                n379 = case shown="True" w490 {
                                frame False {
                                }
                                frame True {
                                # "Set the Wavemeter to\nthe non HSRL wavelength"
                                n380 = Build Array(TRUE ("Boolean")) -> (w492:bool[])
                                n381 = call-poly <vilib>:"DAQmx Write.vi"("task/channels in"=refnum<k21> "HSRL_WV_switch", "data"=w492) -> ()  [unwired: 11 in, 3 out]
                                }
                                }
                                }
                                frame #1 {
                                # "Reading the wavelength from the wavemeter"
                                n382 = flat-sequence {
                                tunnel: [w497] -> w496
                                tunnel: w496 -> [w500]
                                tunnel: [w499] -> w495
                                tunnel: w495 -> [w503]
                                frame #0 {
                                n383 = local read "Bristol In"() -> (w498:i32)
                                n384 = dll-call lib="C:/Users/eol-lidar/Desktop/20171016_WVDIALLabviewSlimmed/DLLs/CLDevIface.dll" fn="CLOpenUSBSerialDevice"("commPort"=w498) -> ("return type"=w497:i32)  [unwired: 4 in, 2 out]
                                }
                                frame #1 {
                                n385 = dll-call lib="C:/Users/eol-lidar/Desktop/20171016_WVDIALLabviewSlimmed/DLLs/CLDevIface.dll" fn="CLGetLambdaReading"("devHandle"=w500) -> ("return type"=→"HSRL Read (nm)":dbl, "devHandle"=w499:i32)  [unwired: 3 in, 2 out]
                                }
                                frame #2 {
                                n386 = dll-call lib="C:/Users/eol-lidar/Desktop/20171016_WVDIALLabviewSlimmed/DLLs/CLDevIface.dll" fn="CLCloseDevice"("commPort"=w503) -> ("return type"=w502:i32)  [unwired: 4 in, 2 out]
                                n387 = local write "Bristol Out"(w502) -> ()
                                }
                                }
                                }
                                frame #2 {
                                # "Calculating the difference between the actual and desired online wavelength"
                                n388 = local read "HSRL_Tol"() -> (w506:dbl)
                                n389 = local read "HSRL Read (nm)"() -> (w512:dbl)
                                n390 = Multiply(x=-1.0, y=w506) -> (x*y=w505:dbl)
                                n391 = Subtract(x=w512, y="HSRL Set (nm)") -> (x-y=w508:dbl)
                                "HSRL_Diff" <- w508
                                n392 = Greater?(x=w508, y=w505) -> (0:w509:bool)
                                n393 = Less?(x=w508, y=w506) -> (x < y?=w510:bool)
                                n394 = And(x=w509, y=w510) -> (x .and. y?=w504:bool)
                                "HSRL Locked" <- w504
                                n395 = case shown="True" w504 {
                                frame False {
                                }
                                frame True {
                                # "Set the Wavementer switch to WV Online"
                                n396 = Build Array(FALSE ("Boolean")) -> (w514:bool[])
                                n397 = Build Array(FALSE ("Boolean")) -> (w518:bool[])
                                n398 = call-poly <vilib>:"DAQmx Write.vi"("task/channels in"=refnum<k21> "BristolWM", "data"=w518) -> ("error out"=w513:errorcluster)  [unwired: 11 in, 2 out]
                                n399 = call-poly <vilib>:"DAQmx Write.vi"("task/channels in"=refnum<k21> "HSRL_WV_switch", "data"=w514, "error in"=w513) -> ()  [unwired: 10 in, 3 out]
                                n400 = Wait (ms)(milliseconds to wait=u32 3200) -> ()  [unwired: 1 out]
                                }
                                }
                                }
                                frame #3 {
                                # "If the wavelength difference is greater that 0.0002 nm, decrement the \nDBR current by 0.01 mA"
                                n401 = local read "HSRL_Diff"() -> (w523:dbl)
                                n402 = Greater Or Equal?(x=w523, y="HSRL_Tol") -> (x >= y?=w522:bool)
                                n403 = case shown="True" w522 {
                                frame False {
                                # "Wavelength difference is not greater than 0.0002 nm, do nothing"
                                }
                                frame True {
                                # "Generating a command string\nto decrement the current"
                                n404 = local read "Settings"() -> (w530:T6)
                                n405 = local read "temp step size"() -> (w524:dbl)
                                n406 = Unbundle By Name(w530) -> ("HSRL TEC"=w529:dbl)
                                n407 = Subtract(x=w529, y=w524) -> (x-y=w528:dbl)
                                n408 = local read "Device In"() -> (w526:refnum<visa-resource-name>)
                                n409 = Bundle By Name(cluster=w530, "HSRL TEC"=w528, "Module"=T12."HSRL TEC") -> (w531:T6)
                                n410 = call "TL_Driver_v2.vi"("Device In"=w526, "Commands"=T9."SET", "Settings"=w531) -> ("Readings"=w532:T7)  [unwired: 9 in, 3 out]
                                n411 = local write "Settings"(w531) -> ()
                                n412 = local write "Readings"(w532) -> ()
                                }
                                }
                                }
                                frame #4 {
                                # "If WL difference is < 0.0002 nm, increment the DBR temperature"
                                n413 = local read "HSRL_Diff"() -> (w535:dbl)
                                n414 = Less Or Equal?(x=w535, y=-0.0001) -> (x <= y?=w533:bool)
                                n415 = case shown="True" w533 {
                                frame False {
                                # "WL difference is no <= to -0.0002 nm, do nothing"
                                }
                                frame True {
                                # "Generating a command string\nto decrement the current"
                                # "WL difference is less than 0.0002 nm,\nincrement the DBR current by 0.01 mA"
                                n416 = local read "Settings"() -> (w543:T6)
                                n417 = local read "temp step size"() -> (w536:dbl)
                                n418 = Unbundle By Name(w543) -> ("HSRL TEC"=w541:dbl)
                                n419 = Add(x=w541, y=w536) -> (x+y=w540:dbl)
                                n420 = local read "Device In"() -> (w538:refnum<visa-resource-name>)
                                n421 = Bundle By Name(cluster=w543, "HSRL TEC"=w540, "Module"=T12."HSRL TEC") -> (w544:T6)
                                n422 = call "TL_Driver_v2.vi"("Device In"=w538, "Commands"=T9."SET", "Settings"=w544) -> ("Readings"=w542:T7)  [unwired: 9 in, 3 out]
                                n423 = local write "Settings"(w544) -> ()
                                n424 = local write "Readings"(w542) -> ()
                                }
                                }
                                }
                              }
                              n425 = Or(x=w486, y="Cancel HSRL") -> (x .or. y?=w487:bool)
                            }
                          }
                        }
                      }
                    }
                  }
                  frame #1 {
                    # "Reading the power meter"
                    # "Updating the pulse energy plot"
                    # "Converting to pulse energy"
                    # "Reading the offline output power, converting to pulse energy,  and updating the Pulse energy plot"
                    n426 = local read "SampleSize"() -> (w556:i32)
                    n427 = local read "Newport Device Key"() -> (w557:string)
                    n428 = local read "WV Online Pulse Energy"() -> (w562:dbl)
                    n429 = local read "WV Offline Pulse Energy"() -> (w561:dbl)
                    n430 = local read "HSRL Pulse Energy"() -> (w546:dbl)
                    n431 = local read "WV_averaged_energy"() -> (w545:dbl)
                    n432 = local read "NewportRef"() -> (w554:refnum<k24>)
                    n433 = Number To Decimal String(number=w556) -> (decimal integer string=w558:string)  [unwired: 1 in]
                    n434 = invoke class="PowerMeterCommands" method="PerformDAQ"(reference=w554, "deviceKey"=w557, "interval"="1", "sampleSize"=w558) -> ("PerformDAQ"=w559:dbl[])  [unwired: 2 in, 5 out]
                    n435 = Bundle("WV Online Pulse Energy"=w562, "WV Offline Pulse Energy"=w561, "HSRL Pulse Energy"=w546, "WV_averaged_energy"=w545) -> (w547:T15)  [unwired: 1 in]
                    n436 = local write "Pulse Energy (Micro Joule)"(w547) -> ()
                    n437 = call-poly <vilib>:"Mean.vi"("X"=w559) -> ("mean"=w555:dbl)  [unwired: 1 out]
                    n438 = Multiply(x=w555, y=1000.0) -> (x*y=w566:dbl)
                    n439 = Divide(x=w566, y=0.05) -> (x/y=w564:dbl)
                    n440 = Divide(x=w564, y=7.0) -> ()  [unwired: 1 out]
                    n441 = global read "AMCS_Data.vi" "AMCS_PowerMon"() -> (w550:u32[])
                    n442 = global read "AMCS_Data.vi" "AMCS_PowerMon"() -> (w553:u32[])
                    n443 = Index Array(array=w550, index=1) -> (element=→"HSRL Pulse Energy":u32)
                    n444 = Index Array(array=w553, index=0) -> (element=→"WV Offline Pulse Energy":u32)
                  }
                  frame #2 {
                    # "Added in the ability to interactively control the ThorLab  setting (just etalon temp for now)"
                    # "Wait 'Scalar Wait Time' for buffers to clear of online contiminated offline data"
                    n445 = disable-structure shown="Disabled" {
                      frame Disabled {
                        # "Wait 'Scalar Wait Time'"
                        n446 = local read "Scalar Wait Time"() -> (w583:u32)
                        n447 = Wait (ms)(milliseconds to wait=w583) -> ()  [unwired: 1 out]
                      }
                      frame Enabled {
                      }
                    }
                    n448 = event shown="[2] \"Settings.HSRL Etalon TEC\": Value Change" {
                      selector: _ -> [_ _ _]
                      dyn-events: _ -> [_ _ _]
                      timeout: 1 -> [_ _ _]
                      event Timeout {
                        n449 = event-data() -> ()  [unwired: 1 in, 2 out]
                      }
                      event "Settings.WV Etalon TEC": Value Change {
                        # "Generating a command string\nto update the etalon"
                        n450 = event-data() -> ()  [unwired: 1 in, 5 out]
                        n451 = local read "Settings"() -> (w573:T6)
                        n452 = Unbundle By Name(w573) -> ("WV Etalon TEC"=w575:dbl)
                        n453 = local read "Device In"() -> (w569:refnum<visa-resource-name>)
                        n454 = Bundle By Name(cluster=w573, "WV Etalon TEC"=w575, "Module"=T12."WV Etalon TEC") -> (w571:T6)
                        n455 = call "TL_Driver_v2.vi"("Device In"=w569, "Commands"=T9."SET", "Settings"=w571) -> ("Readings"=w572:T7)  [unwired: 9 in, 3 out]
                        n456 = local write "Readings"(w572) -> ()
                        n457 = local write "Settings"(w571) -> ()
                      }
                      event "Settings.HSRL Etalon TEC": Value Change {
                        # "Generating a command string\nto update the etalon"
                        n458 = event-data() -> ()  [unwired: 1 in, 5 out]
                        n459 = local read "Settings"() -> (w580:T6)
                        n460 = Unbundle By Name(w580) -> ("HSRL Etalon TEC"=w582:dbl)
                        n461 = local read "Device In"() -> (w576:refnum<visa-resource-name>)
                        n462 = Bundle By Name(cluster=w580, "HSRL Etalon TEC"=w582, "Module"=T12."HSRL Etalon TEC") -> (w578:T6)
                        n463 = call "TL_Driver_v2.vi"("Device In"=w576, "Commands"=T9."SET", "Settings"=w578) -> ("Readings"=w579:T7)  [unwired: 9 in, 3 out]
                        n464 = local write "Readings"(w579) -> ()
                        n465 = local write "Settings"(w578) -> ()
                      }
                    }
                  }
                  frame #3 {
                    w600 = 1
                    w629 = 1 ("dimension size")
                    # "Plotting the normalized relative \nbackscatter"
                    # "Calculating the normalized relative backscatter"
                    # "File path in MATLAB script is of old dial is:\nF:\\Micropulse DIAL\\Micropulse DIAL Matlab\\\nFinal Overlap Function.mat')];"
                    # "Read in latest scalar card data from \n'Scalar Data' global variable that \nscaler.vi is writing to, then wait 1 sec\nfor next batch of data"
                    # "Calculating/Plotting smoothed data,\ncross sections etc."
                    # "Pick off data with\nout header"
                    # "Calculate mean bin by bin mean"
                    # "Reading in 'Integration Period (Seconds)' of data"
                    # "Read the offline data from the scalar card, perform smoothing, calculate normalized relative backscatter, and plot"
                    # "Collects Data From Card,\nSends It To The Chart,\nAnd Saves A Copy As A\nFile If Option Selected On\nFront Panel"
                    n466 = local read "Total DIAL Integration Time (Minutes)"() -> (w645:i32)
                    n467 = local read "bins"() -> (w584:u32)
                    n468 = for {
                      N: "Data Reads (number of loops)" -> [_]
                      tunnel: [w657] -> w620 mode=indexing
                      tunnel: [w653] -> w619 mode=indexing
                      tunnel: w584 -> [w654]
                      n469 = global read "AMCS_Data.vi" "AMCS_Data"() -> (w660:u16[][])
                      n470 = disable-structure shown="Disabled" {
                        frame Disabled {
                          n471 = global read "Scalar_Data_4.vi" "Scalar Data 4"() -> ()  [unwired: 1 out]
                          n472 = global read "Scalar_Data_2.vi" "Scalar Data 2"() -> ()  [unwired: 1 out]
                        }
                        frame Enabled {
                        }
                      }
                      n473 = Index Array(array=w660, index (row) #1=1 ("index (row)"), index (row) #2=3 ("index (row)")) -> (element #1=w659:u16[], element #2=w656:u16[])  [unwired: 2 in]
                      n474 = Array Subset(array=w656, index=0, length=w654) -> (w653:u16[])
                      n475 = Array Subset(array=w659, index=0, length=w654) -> (w657:u16[])
                    }
                    n476 = Divide(x=w645, y="Data Reads (number of loops)") -> (x/y=w643:dbl)
                    n477 = local read "Total Aerosol Integration Time (Minutes)"() -> (w646:dbl)
                    n478 = Multiply(x=w643, y=60.0) -> (x*y=w633:dbl)
                    n479 = local read "background length"() -> (w624:i32)
                    n480 = local read "background start"() -> (w625:u32)
                    n481 = Transpose 2D Array(2D array=w620) -> (transposed array=w651:u16[][])
                    n482 = Transpose 2D Array(2D array=w619) -> (transposed array=w638:u16[][])
                    n483 = Divide(x=w646, y="Data Reads (number of loops)") -> (x/y=w647:dbl)
                    n484 = for {
                      N: w584 -> [_]
                      tunnel: w651 -> [w666] mode=indexing
                      tunnel: [w665] -> w652 mode=indexing
                      tunnel: w638 -> [w664] mode=indexing
                      tunnel: [w663] -> _ mode=indexing
                      tunnel: [w663] -> w635 mode=indexing
                      n485 = call-poly <vilib>:"Mean.vi"("X"=w666) -> ("mean"=w665:dbl)  [unwired: 1 out]
                      n486 = call-poly <vilib>:"Mean.vi"("X"=w664) -> ("mean"=w663:dbl)  [unwired: 1 out]
                    }
                    n487 = Multiply(x=w647, y=60.0) -> (x*y=w616:dbl)
                    n488 = Array Subset(array=w635, index=w629, length=w584) -> (w636:dbl[])
                    "CH3 Bin Readings" <- w636
                    n489 = Array Subset(array=w652, index=w629, length=w584) -> (w634:dbl[])
                    "CH1  Bin Readings" <- w634
                    n490 = Array Subset(array=w636, index=w625, length=w624) -> (w637:dbl[])
                    n491 = Array Subset(array=w634, index=w625, length=w624) -> (w650:dbl[])
                    n492 = local read "Smoothed Bins"() -> (w621:dbl)
                    n493 = call-poly <vilib>:"Mean.vi"("X"=w637) -> ("mean"=w606:dbl)  [unwired: 1 out]
                    n494 = call-poly <vilib>:"Mean.vi"("X"=w650) -> ("mean"=w611:dbl)  [unwired: 1 out]
                    n495 = local read "Index"() -> (w617:i32)
                    n496 = Subtract(x=w636, y=w606) -> (x-y=w618:dbl[])
                    n497 = Subtract(x=w634, y=w611) -> (x-y=w632:dbl[])
                    n498 = call "Ring Buffer CH1 short rev2.vi"("Index"=w617, "Profiles to Average"=w633, "Input Array"=w632) -> ("AvgArray"=w649:dbl[], "RingBufferOut"=→"CH1 RingBuffer long":dbl[][])  [unwired: 7 in]
                    n499 = call "Ring Buffer CH3 short rev2.vi"("Index"=w617, "Profiles to Average"=w616, "Input Array"=w618) -> ("AvgArray"=w627:dbl[], "RingBufferOut"=→"CH3 RingBuffer short":dbl[][])  [unwired: 7 in]
                    n500 = Reshape Array(w632, w629, w584) -> (→"CH 1 (WV off) counts display":dbl[][])
                    n501 = Reshape Array(w618, w629, w584) -> (→"CH 3 (HSRL comb) counts display":dbl[][])
                    n502 = local read "Time Resolution Per Bin(ns)"() -> (w607:u32)
                    n503 = local read "Number of Accumulates"() -> (w605:u32)
                    n504 = call "Smooth Arrray.vi"("smooth size"=w621, "Raw Array"=w649) -> ("Smoothed Array"=w585:dbl[])  [unwired: 9 in]
                    "CH1 (WV off) smooth" <- w585
                    n505 = call "Smooth Arrray.vi"("smooth size"=w621, "Raw Array"=w627) -> ("Smoothed Array"=w623:dbl[])  [unwired: 9 in]
                    "CH3 (HSRL combined) smooth" <- w623
                    n506 = local read "Temperature (C)"() -> (w642:dbl)
                    n507 = local read "Pressure (mb)"() -> (w641:dbl)
                    n508 = To Double Precision Float(number=w605) -> (double precision float=w604:dbl)
                    n509 = To Double Precision Float(number=w607) -> (double precision float=w603:dbl)
                    n510 = Reciprocal(x=w603) -> (1/x=w614:dbl)
                    n511 = script code="%accum_num=10000;     % scaler card setting number of accumulations\nt_bin = t_bin_in/1e9                 % scaler card setting time per bin\n%t_d = 37.3e-9;                % APD dead time from spec sheet\n\n% conversion from accumulated counts to count rate  (c/s)\nc_convert = 1./t_bin./accum_num;\nCR_WV = p_raw_WV.*c_convert;\nCR_HSRL = p_raw_HSRL.*c_convert;\nCR_total_WV = (p_raw_WV+b_WV).*c_convert;\nCR_total_HSRL = (p_raw_HSRL+b_HSRL).*c_convert;\nb_CR_WV =b_WV.*c_convert;\nb_CR_HSRL =b_HSRL.*c_convert;\n \n% create a range array\nsize_p =  size(p_raw_WV,2);\ngate = t_bin*3e8/2;\nr = (gate:gate:size_p*gate)./1e3; \n   \n%APD correction factor\n D_WV = 1./(1-(t_d*CR_total_WV));\n D_HSRL = 1./(1-(t_d*CR_total_HSRL));\n\n %Calculating normalize relative backscatter profile\n nrb_WV = CR_WV.*D_WV.*r.^2.*1e-6;\n nrb_HSRL = CR_HSRL.*D_HSRL.*r.^2.*1e-6;"("E"=6.0 ("Real"), "temp"=w642, "press"=w641, "p_raw_WV"=w585, "b_WV"=w611, "b_HSRL"=w606, "p_raw_HSRL"=w623, "accum_num"=w604, "t_d"="dead time", "t_bin_in"=w603) -> ("nrb_WV"=w593:cdb[], "D_WV"=w590:dbl[], "nrb_HSRL"=w592:cdb[], "D_HSRL"=w589:dbl[])  [unwired: 1 in, 1 out]
                    n512 = Divide(x=w614, y=w604) -> (x/y=w612:dbl)
                    n513 = Multiply(x=1000000000.0, y=w612) -> (x*y=w609:dbl)
                    n514 = Multiply(x=w609, y=w611) -> (x*y=w610:dbl)
                    n515 = Multiply(x=w609, y=w606) -> (x*y=w608:dbl)
                    n516 = Bundle(w610, w608) -> (→"?":cluster{dbl, dbl})  [unwired: 1 in]
                    n517 = local read "bins"() -> (w599:u32)
                    n518 = local read "Altitude Array (km)"() -> (w595:dbl[])
                    n519 = Build Array(w593, w592) -> (w597:cdb[][])
                    n520 = Build Array(w590, w589) -> (w588:dbl[][])
                    n521 = Reshape Array(w592, w600, w599) -> (→"NRB HSRL Combined":cdb[][])
                    n522 = Reshape Array(w593, w600, w599) -> (→"NRB WV Offline":cdb[][])
                    n523 = Build Array(w595, w595) -> (w594:dbl[][])
                    n524 = call "Convert to Dynamic Data7"("2D Array"=w588) -> ("Dynamic Data Type"=w587:dynamicdata)  [unwired: 3 in]
                    n525 = call "Convert to Dynamic Data3"("2D Array"=w597) -> ("Dynamic Data Type"=w596:dynamicdata)  [unwired: 3 in]
                    n526 = call "Convert to Dynamic Data4"("2D Array"=w594) -> ("Dynamic Data Type"=w591:dynamicdata)  [unwired: 3 in]
                    n527 = call "Build XY Graph2"("Y Input"=w591, "X Input"=w596) -> ("XY Graph"=→"NRB plot":cluster{"Y":dbl[], "Y":dbl[]}[])  [unwired: 3 in, 6 out]
                    n528 = call "Build XY Graph4"("Y Input"=w591, "X Input"=w587) -> ("XY Graph"=→"Correction":cluster{"Y":dbl[], "Y":dbl[]}[])  [unwired: 3 in, 6 out]
                  }
                  frame #4 {
                    # "REPLACE WITH NEW AGILTRON TASK!"
                    # "Toggle Agiltron switch to online DBR"
                    n529 = disable-structure shown="Disabled" {
                      frame Disabled {
                        # "ABSORBING"
                        n530 = flat-sequence {
                          frame #0 {
                            # "Third one"
                            # "Command the switch to switch to position 1\ncorresponding to the online DBR"
                            # "Hex string command \ncorrespond to online"
                            n531 = local read "Switch Comm Port"() -> (w670:refnum<visa-resource-name>)
                            n532 = VISA Write(VISA resource name=w670, write buffer="\u0001\u0012\u0000\u0002") -> ()  [unwired: 1 in, 3 out]
                          }
                        }
                        n533 = Build Array(FALSE ("Boolean")) -> (w669:bool[])
                        n534 = call-poly <vilib>:"DAQmx Write.vi"("task/channels in"=refnum<k21> "AgiltronSwitch", "data"=w669) -> ()  [unwired: 11 in, 3 out]
                      }
                      frame Enabled {
                      }
                    }
                  }
                  frame #5 {
                    # "If 'Save Data?' is true, save all relavant offline info"
                    n535 = local read "Save Data?"() -> (w672:bool)
                    n536 = case shown="True" w672 {
                      frame False {
                        # "'Save Data?' is false, do nothing"
                      }
                      frame True {
                        # "Write only one data file at this time"
                        # "Retrive Julian Date"
                        # "'Save Data?' is true, save offline data to the Data Disk"
                        n537 = local read "Readings"() -> (w675:T7)
                        n538 = Unbundle By Name(w675) -> ("WV Offline TEC"=w676:dbl)
                        n539 = local read "HSRL Pulse Energy"() -> (w674:dbl)
                        n540 = Unbundle By Name(w675) -> ("HSRL TEC"=w677:dbl)
                        n541 = local read "HSRL Read (nm)"() -> (w678:dbl)
                        n542 = local read "WV Offline Read (nm)"() -> (w699:dbl)
                        n543 = local read "WV Offline Pulse Energy"() -> (w673:dbl)
                        n544 = local read "Relative Humdity (%)"() -> (w702:dbl)
                        n545 = local read "CH3 Bin Readings"() -> (w697:dbl[])
                        n546 = local read "CH1  Bin Readings"() -> (w703:dbl[])
                        n547 = local read "Temperature (C)"() -> (w700:dbl)
                        n548 = local read "Pressure (mb)"() -> (w701:dbl)
                        n549 = call "Julian_Date_2.vi"() -> ("Julian Date"=w698:dbl)  [unwired: 11 in]
                        n550 = Build Array (concatenate)(w698, w699, w676, w673, w700, w701, w702, w703) -> (w683:dbl[])
                        n551 = Build Array (concatenate)(w698, w678, w677, w674, w700, w701, w702, w697) -> (w680:dbl[])
                        n552 = local read "FF_Off_Ref"() -> (w685:refnum<file>)
                        n553 = local read "NF_Off_Ref"() -> (w682:refnum<file>)
                        n554 = local read "FF_Off_Ptr"() -> (w684:i64)
                        n555 = local read "NF_Off_Ptr"() -> (w681:i64)
                        n556 = Set File Position(offset (in bytes) (0)=w684, refnum=w685) -> (refnum out=w696:refnum<file>, error out=w694:errorcluster)  [unwired: 2 in]
                        n557 = Set File Position(offset (in bytes) (0)=w681, refnum=w682) -> (refnum out=w692:refnum<file>, error out=w690:errorcluster)  [unwired: 2 in]
                        n558 = Write to Binary File(file (use dialog)=w696, data=w683, error in=w694, 5:FALSE ("prepend array or string size? (T)")) -> (refnum out=w695:refnum<file>, error out=w693:errorcluster)  [unwired: 2 in, 1 out]
                        n559 = Write to Binary File(file (use dialog)=w692, data=w680, error in=w690, 5:FALSE ("prepend array or string size? (T)")) -> (refnum out=w691:refnum<file>, error out=w689:errorcluster)  [unwired: 2 in, 1 out]
                        n560 = Get File Position(4:w693, 7:w695) -> (2:w686:i64)  [unwired: 2 out]
                        n561 = Get File Position(4:w689, 7:w691) -> (2:w679:i64)  [unwired: 2 out]
                        n562 = local write "FF_Off_Ptr"(w686) -> ()
                        n563 = local write "NF_Off_Ptr"(w679) -> ()
                      }
                    }
                  }
                }
              }
              frame #4 {
                n564 = First Call?() -> (First Call?: T/F=w706:bool)
                n565 = Or(x="calculate absorption cross sections", y=w706) -> (x .or. y?=w704:bool)
                n566 = case shown="True" w704 {
                  frame False {
                  }
                  frame True {
                    # "calculate absorption cross sections from HITRAN data base"
                    n567 = local read "WV Offline Set (nm)"() -> (w710:dbl)
                    n568 = local read "WV Online Read (nm)"() -> (w713:dbl)
                    n569 = local read "CH1 (WV off) smooth"() -> (w714:dbl[])
                    n570 = local read "Temperature (C)"() -> (w712:dbl)
                    n571 = local read "Pressure (mb)"() -> (w711:dbl)
                    n572 = local read "gate size"() -> (w707:dbl)
                    n573 = script code="hitran = dlmread('C:\\Users\\eol-lidar\\Desktop\\20171016_WVDIALLabviewSlimmed\\HiranData\\815nm_841nm_HITRAN_2008.csv', ',',[1 1 1676 8]);\n\n\n%hitran = dlmread('C:\\Users\\H2ODial\\Desktop\\Shared Telescope WV DIAL Code\\Libraries and VIs\\815nm_841nm_HITRAN_2008.csv', ',',[1 1 1676 8]);\n%hitran = dlmread('C:\\Users\\H2ODial\\Desktop\\Shared Telescope WV DIAL Code\\Libraries and VIs\\824nm_841nm_H2O.csv', ',',[0 1 352 7]);\n%hitran = dlmread('C:\\Users\\H2ODial\\Desktop\\Shared Telescope WV DIAL Code\\Libraries and VIs\\824nm_841nm_H2O_Spectral_Calc.csv', ',',[1 1 1209 7]);\n\n%Range vector in meters\n%range = ([75:75:size(Online,2)*75]);\ntest = size(Online,2);\nrange = ([gate_size:gate_size:test.*gate_size]); \n\nif lambda< 828\nlambda=828.195;\nelse\nlambda=lambda;\nend;\n\n%%\n\n%Voigt profile calculation\nWNmin = 1/(828+4)*1e7;  % 832.0 nm converted to wavenumber\nWNmax = 1/(828-4)*1e7;  % 824.0 nm converted to wavenumber\n\n%Find lines from WNmin to WNmax to calculate voigt profile\nline_indices = hitran(1:size(hitran,1),1)>WNmin & hitran(1:size(hitran,1),1)<WNmax;\n\nline = double(hitran(line_indices, 1:size(hitran,2)));\n\n%Calculate temperature and pressure profile\nT0 = 273+25; % surface temperature\nT0 = 273+T0_C;\nT = T0-0.0065.*range; % set to match the sounding\n\n% pressure in atmospheres\nP0  = 0.83; % surface pressure\nP0  = P0_mb/1000*0.986; %pressure in mb converted to atm\nP = P0.*(T0./T).^-5.5;   % set this value to match sounding\n\nT00 = 296;              % HITRAN reference temperature [K]\nP00 = 1;                % HITRAN reference pressure [atm]\nnu0_0 = line(:,1);      % absorption line center wavenumber from HITRAN [cm^-1]\nS0 = line(:,2);         % initial linestrength from HITRAN [cm^-1/(mol*cm^-2)]   \ngammal0 = line(:,4);    % air-broadened halfwidth at T_ref and P_ref from HITRAN [cm^-1/atm]\ngamma_s = line(:,5);    % self-broadened halfwidth at T_ref and P_ref from HITRAN [cm^-1/atm]\nE = line(:,6);          % ground state transition energy from HITRAN [cm^-1]  \nalpha = line(:,7);      % linewidth temperature dependence factor from HITRAN\ndelta = line(:,8);      % pressure shift from HiTRAN [cm^-1 atm^-1]\nnu_on = 1/(lambda)*1e7;\nnu_off = 1/(lambda_off)*1e7;\n\nfor i = 1:size(Online,2); % calculate the absorption cross section at each range\n  \n    nu0 = nu0_0+delta.*(P(i)./P00); % unclear if it should be Pi/P00  \n    gammal = gammal0.*(P(i)./P00).*((T00./T(i)).^alpha);    %Calculate Lorentz lineweidth at P(i) and T(i)\n\n    const.m = 18.015E-3./6.022E23; % mass of a single water molecule\n    const.k_B = 1.3806488e-23; % (J/K)\n    const.c = 299792458; % (m/s) (exact)\n \n    gammad = (nu0).*((2.0.*const.k_B.*T(i).*log(2.0))./(const.m.*const.c^2)).^(0.5);  %Calculate HWHM Doppler linewidth at T(i)\n     \n    % term 1 in the Voigt profile\n    y = (gammal./gammad).*((log(2.0)).^(0.5));\n    \n    % term 2 in the Voigt profile\n    x_on = ((nu_on-nu0)./gammad).*(log(2.0)).^(0.5);\n    x_off = ((nu_off-nu0)./gammad).*(log(2.0)).^(0.5);\n    \n    %setting up Voigt convolution\n    t = (-(size(line,1))/2:1:size(line,1)/2-1); %set up the integration spectral step size\n    t = repmat(t',1,length(x_on))';\n    x_on = repmat(x_on,1,length(t));\n    x_off = repmat(x_off,1,length(t));\n    y = repmat(y,1,length(t));\n    f_on = (exp(-t.^2.0))./(y.^2.0+(x_on-t).^2.0);  % combined Voigt term 1 and 2\n    f_off = (exp(-t.^2.0))./(y.^2.0+(x_off-t).^2.0);\n    %Voigt integration over all of the lines at the on and offline locations\n    z_on = trapz(t(1,:),f_on,2);\n    z_off =  trapz(t(1,:),f_off,2);\n    integral_on = z_on;\n    integral_off = z_off;\n    %Calculate linestrength at temperature T\n    S = S0.*((T00./T(i)).^(1.5)).*exp(1.439.*E.*((1./T00)-(1./T(i))));\n \n    %Calculate the Voigt profile\n    K_on = (y(:,1)./pi).*integral_on;\n    K_off = (y(:,1)./pi).*integral_off;\n    \n    %Calculate the Voigt profile absorption cross section [cm^2]\n    sigmav_on = S.*(1./gammad).*(((log(2.0))./pi).^(0.5)).*K_on; %.*far_wing_on;\n    sigmav_off = S.*(1./gammad).*(((log(2.0))./pi).^(0.5)).*K_off; %.*far_wing_off;\n    \n    %Sum contributions from all of the surrounding lines\n    sigma_on_total(i) = sum(sigmav_on);\n    sigma_off_total(i) = sum(sigmav_off);\n    \nend;"("lambda"=w713, "lambda_off"=w710, "P0_mb"=w711, "T0_C"=w712, "Online"=w714, "gate_size"=w707) -> ("sigma_on_total"=→"sigma_on_total":dbl[], "sigma_off_total"=→"sigma_off_total":dbl[])  [unwired: 1 in, 1 out]
                  }
                }
              }
              frame #5 {
                # "normalization factor\nfrom 300 to 450m"
                # "OPTICAL DEPTH PLOT"
                # "Data Processing Far Channel"
                # "Calculating the range resolved water vapor number density and plotting"
                n574 = local read "gate size"() -> (w729:dbl)
                n575 = local read "CH3 (HSRL combined) smooth"() -> (w769:dbl[])
                n576 = local read "CH2 (molecular) smoothed"() -> (w768:dbl[])
                n577 = local read "CH0 (WV on) smoothed"() -> (w748:dbl[])
                n578 = local read "CH1 (WV off) smooth"() -> (w747:dbl[])
                n579 = local read "Temperature (C)"() -> (w727:dbl)
                n580 = local read "sigma_off_total"() -> (w771:dbl[])
                n581 = local read "sigma_on_total"() -> (w770:dbl[])
                n582 = local read "Pressure (mb)"() -> (w728:dbl)
                n583 = script code="backscatter_ratio = combined./molecular;\n\n% calculate the temp and pressure profiles from surface measurement\nT0 = 273+T0_C;\n% create a range array\n range = ([0:gate_size:(size(combined,2)-1)*gate_size]); \n T = T0-0.0065.*range; \n P0  = P0_mb/1000*0.986; %pressure in mb converted to atm\n P = P0.*(T0./T).^-5.5;   \n const.k_B = 1.363806488e-23; % (J/K)\n const.k_B = 1.363806488e-23*9.89*10^-6; % (atm m^3/K)\n% backscatter coefficient in m^-1 sr^-1\nbeta_m_profile = 5.45.*10^(-32).*(550/780.2)^4.*P./(T.*const.k_B);\n\nbeta_m_array = repmat(beta_m_profile, size(backscatter_ratio,1), 1);\nbeta_bs = ((backscatter_ratio.*receiver_scale_factor)-1).*beta_m_profile"("molecular"=w768, "combined"=w769, "gate_size"=w729, "T0_C"=w727, "P0_mb"=w728, "receiver_scale_factor"="Receiver Scale Factor") -> ("beta_bs"=w715:dbl[], "beta_m_profile"=w717:dbl[])  [unwired: 1 in, 2 out]
                n584 = script code="%Time averaging in seconds.  600 Seconds =10 minutes\ntemporal_average = 600;\n%Spatial averaging in bins.  150 meters\nspatial_average = 150./gate_size;\n%Creating r and r+deltar vectors..this can also be acsomplished using the diff command\np_oni = Online(:,1:size(Online,2)-1);\np_onii = Online(:,2:size(Online,2));\np_offi = Offline(:,1:size(Offline,2)-1);\np_offii = Offline(:,2:size(Offline,2));\nInside = (p_oni.*p_offii)./(p_onii.*p_offi);\ndel_cross = 1./(2.*(sigma_on_total(1:size(Online,2)-1)-sigma_off_total(1:size(Offline,2)-1)).*gate_size*100);\ndel_cross(isinf(del_cross)) = 0;\n%Calculating Number density\nN = del_cross.*log(Inside);\n%Spatial smoothing of the profiles\nfilter1 = ones(1,4)./4;\nN_1 = N;\nN_1_avg = filter2(filter1,N_1);\nfilter1 = ones(1,10)./10;\nN_2 = N;\nN_2_avg = filter2(filter1,N_2);\nN_new = zeros(size(N,1),size(N,2));\n%Using different averaging windows for different altitudes \nN_avg=[N_1_avg(:,1:40)';N_2_avg(:,41:size(N,2))']';\nw = N_avg.*1e6.*18.015./6.022e23"("Online"=w748, "Offline"=w747, "sigma_on_total"=w770, "sigma_off_total"=w771, "gate_size"=w729) -> ("N_avg"=w731:cdb[], "w"=w732:cdb[])  [unwired: 1 in, 1 out]
                n585 = local read "Number of Bins"() -> (w737:u32)
                n586 = local read "Altitude Array (km)"() -> (w716:dbl[])
                n587 = local read "Time Resolution Per Bin(ns)"() -> (w746:u32)
                n588 = local read "Number of Bins"() -> (w725:u32)
                n589 = Logarithm Base 10(1:w715) -> (0:w722:dbl[])
                n590 = Reshape Array(w732, 1, w737) -> (→"Absolute Humdity":cdb[][])
                n591 = Build Array(w717, w715) -> (w719:dbl[][])
                n592 = Reshape Array(w722, 1, w725) -> (→"Backscatter coef":dbl[][])
                n593 = call "Convert to Dynamic Data9"("Array"=w731) -> ("Dynamic Data Type"=w735:dynamicdata)  [unwired: 3 in]
                n594 = To Double Precision Float(number=w746) -> (double precision float=w767:dbl)
                n595 = call "Convert to Dynamic Data6"("Array"=w732) -> ("Dynamic Data Type"=w733:dynamicdata)  [unwired: 3 in]
                n596 = Multiply(x=0.15, y=w767) -> (x*y=w765:dbl)
                n597 = call "Convert to Dynamic Data8"("Array"=w716) -> ("Dynamic Data Type"=w736:dynamicdata)  [unwired: 3 in]
                n598 = call "Convert to Dynamic Data5"("Array"=w716) -> ("Dynamic Data Type"=w734:dynamicdata)  [unwired: 3 in]
                n599 = call "Build XY Graph"("Y Input"=w736, "X Input"=w735) -> ("XY Graph"=→"Water Vapor Number Density":cluster{"Y":dbl[], "Y":dbl[]}[])  [unwired: 3 in, 6 out]
                n600 = call "Build XY Graph3"("Y Input"=w734, "X Input"=w733) -> ("XY Graph"=→"Absolute Humidity":cluster{"Y":dbl[], "Y":dbl[]}[])  [unwired: 3 in, 6 out]
                n601 = Divide(x=300.0, y=w765) -> (x/y=w762:dbl)
                n602 = Divide(x=450.0, y=w765) -> (x/y=w761:dbl)
                n603 = call "Convert to Dynamic Data11"("2D Array"=w719) -> ("Dynamic Data Type"=w718:dynamicdata)  [unwired: 3 in]
                n604 = call "Convert to Dynamic Data10"("Array"=w716) -> ("Dynamic Data Type"=w720:dynamicdata)  [unwired: 3 in]
                n605 = To Long Integer(number=w762) -> (32bit integer=w760:i32)
                n606 = To Long Integer(number=w761) -> (32bit integer=w759:i32)
                n607 = Decrement(x=w760) -> (x-1=w757:i32)
                n608 = Decrement(x=w759) -> (x-1=w758:i32)
                n609 = call "Build XY Graph5"("Y Input"=w720, "X Input"=w718) -> ("XY Graph"=→"aerosol profile":cluster{"Y":dbl[], "Y":dbl[]}[])  [unwired: 3 in, 6 out]
                n610 = Array Subset(array=w748, index=w757, length=w758) -> (w756:dbl[])
                n611 = Array Subset(array=w747, index=w757, length=w758) -> (w755:dbl[])
                n612 = call-poly <vilib>:"Mean.vi"("X"=w756) -> ("mean"=w754:dbl)  [unwired: 1 out]
                n613 = call-poly <vilib>:"Mean.vi"("X"=w755) -> ("mean"=w753:dbl)  [unwired: 1 out]
                n614 = Divide(x=w754, y=w753) -> (x/y=w752:dbl)
                n615 = Multiply(x=w747, y=w752) -> (x*y=w751:dbl[])
                n616 = Divide(x=w748, y=w751) -> (x/y=w750:dbl[])
                n617 = Natural Logarithm(1:w750) -> (0:w749:dbl[])
                n618 = Multiply(x=-1.0, y=w749) -> (x*y=w743:dbl[])
                n619 = call "Convert to Dynamic Data"("Array"=w743) -> ("Dynamic Data Type"=w745:dynamicdata)  [unwired: 3 in]
                n620 = call "Convert to Dynamic Data2"("Array"=w716) -> ("Dynamic Data Type"=w742:dynamicdata)  [unwired: 3 in]
                n621 = call "Build OD Plot"("Y Input"=w742, "X Input"=w745) -> ("XY Graph"=→"Optical Depth":cluster{"Y":dbl[], "Y":dbl[]}[])  [unwired: 3 in, 6 out]
              }
            }
          }
        }
        "L_Count" <- w129
      }
    }
  }
  n622 = case shown="True" w3 {
    frame False {
    }
    frame True {
      # "close data files"
      n623 = local read "NF_Off_Ref"() -> (w773:refnum<file>)
      n624 = local read "NF_On_Ref"() -> (w774:refnum<file>)
      n625 = local read "FF_Off_Ref"() -> (w775:refnum<file>)
      n626 = local read "FF_On_Ref"() -> (w776:refnum<file>)
      n627 = local read "WS_On/Off"() -> (w772:bool)
      n628 = case shown="True" w772 {
        frame False {
        }
        frame True {
          n629 = local read "WS visa"() -> (w777:refnum<visa-resource-name>)
          n630 = call "T_RH_P.vi"("VISA in"=w777, "WS_Commands"=enum16{"OpenWS", "ReadTRHP", "CloseWS"}."CloseWS") -> ()  [unwired: 11 in, 3 out]
        }
      }
      n631 = Close File(refnum=w776) -> ()  [unwired: 1 in, 2 out]
      n632 = Close File(refnum=w775) -> ()  [unwired: 1 in, 2 out]
      n633 = Close File(refnum=w774) -> ()  [unwired: 1 in, 2 out]
      n634 = Close File(refnum=w773) -> ()  [unwired: 1 in, 2 out]
    }
  }
  "FileHour" <- -1 ("FileHour")
  "DataOpen" <- FALSE
